vi "Beampointing_Multi_TRA2_BELLA_BTL.vi"() -> ()   [LabVIEW 2020]
uses:
  Shared/GUI_Template/GUI_master/tcp_new_data_event.ctl
  Shared/GUI_Template/GUI_master/tcp new data cluster.ctl
  Ctrs/beam detection.ctl
  GUI_Beampointing_single_TRA/Ctrs/move.ctl
  General GUIs/Device GUIs/GUI_Cameras/Controls/Crosshair type def.ctl
  <vilib>/Utility/file.llb/Read From Spreadsheet File (string).vi
  <userlib>/_OpenG.lib/array/array.llb/Filter 1D Array with Scalar (String)__ogtk.vi
  <vilib>/Analysis/NI_AALBase.lvlib
  <vilib>/vision/NI_Vision_Development_Module.lvlib
  <vilib>/Utility/file.llb/Write To Spreadsheet File (string).vi
panel:
  out "error out 3":errorcluster
  out "Array 3":sgl[](array[numeric])
  in  "GUIdevice 97":string="BELLA_ESP_2"
  in  "GUIdevice 98":string="BellaESP"
  in  "Position.Axis 1::97":dbl=77.0 caption="Motor Axis 1" min=-10.0 max=10.0 format="%#_6f"
  in  "Position.Axis 2::97":dbl=77.0 caption="Motor Axis 1" min=-12.0 max=10.0 format="%#_6f"
  in  "Position.Axis 3::97":dbl=77.0 caption="Motor Axis 1" min=-12.0 max=12.0 format="%#_6f"
  in  "Position.Axis 1::98":dbl=77.0 caption="Motor Axis 1" min=-8.0 max=6.0 format="%#_6f"
  in  "Position.Axis 2::98":dbl=77.0 caption="Motor Axis 1" min=-6.0 max=6.0 format="%#_6f"
  in  "Position.Axis 3::98":dbl=77.0 caption="Motor Axis 1" min=-10.0 max=10.0 format="%#_6f"
  in  "save path":path=path "W:/BP_DATA"
  out "size(s) 6":i32
  out "config path":string
  out "motor refs 7":refnum<vi>[](array[refnum])
  out "Moving Y":string
  out "Moving X":string
  out "particles":T1(array[cluster])
  out "motor refs 6":refnum<vi>[](array[refnum])
  out "millisecond timer value":u32
  out "motor refs 5":refnum<vi>[](array[refnum])
  out "appended path":path
  out "motor refs 4":refnum<vi>[](array[refnum])
  in  "active Axis ref 3":cluster{"Ref X":refnum<vi>, "Ref Y":refnum<vi>}
  out "motor refs 3":refnum<vi>[](array[refnum])
  in  "active man refs":cluster{"Ref X":refnum<vi>, "Ref Y":refnum<vi>}
  out "motor refs 2":refnum<vi>[](array[refnum])
  in  "Numeric":dbl
  out "Current State":string
  in  "output cluster 2":T5 {"detection para"."smal para"."Measurement Parameter" items=["Center of Mass X", "Center of Mass Y", "First Pixel X", "First Pixel Y", "Bounding Rect Left", "Bounding Rect Top", "Bounding Rect Right", "Bounding Rect Bottom", "Max Feret Diameter Start X", "Max Feret Diameter Start Y", "Max Feret Diameter End X", "Max Feret Diameter End Y", "Max Horiz. Segment Length Left", "Max Horiz. Segment Length Right", "Max Horiz. Segment Length Row", "-", "Bounding Rect Width", "Bounding Rect Height", "Bounding Rect Diagonal", "Perimeter", "Convex Hull Perimeter", "Holes' Perimeter", "Max Feret Diameter", "Equivalent Ellipse Major Axis", "Equivalent Ellipse Minor Axis", "Equivalent Ellipse Minor Axis (Feret)", "Equivalent Rect Long Side", "Equivalent Rect Short Side", "Equivalent Rect Diagonal", "Equivalent Rect Short Side (Feret)", "Average Horiz. Segment Length", "Average Vert. Segment Length", "Hydraulic Radius", "Waddel Disk Diameter", "-", "Area", "Holes' Area", "Particle & Holes' Area", "Convex Hull Area", "Image Area", "-", "Number of Holes", "Number of Horiz. Segments", "Number of Vert. Segments", "-", "Orientation", "Max Feret Diameter Orientation", "-", "% Area/Image Area", "% Area/(Particle & Holes' Area)", "Ratio of Equivalent Ellipse Axes", "Ratio of Equivalent Rect Sides", "-", "Elongation Factor", "Compactness Factor", "Heywood Circularity Factor", "Type Factor", "-", "Sum X", "Sum Y", "Sum XX", "Sum XY", "Sum YY", "Sum XXX", "Sum XXY", "Sum XYY", "Sum YYY", "-", "Moment of Inertia XX", "Moment of Inertia XY", "Moment of Inertia YY", "Moment of Inertia XXX", "Moment of Inertia XXY", "Moment of Inertia XYY", "Moment of Inertia YYY", "Norm. Moment of Inertia XX", "Norm. Moment of Inertia XY", "Norm. Moment of Inertia YY", "Norm. Moment of Inertia XXX", "Norm. Moment of Inertia XXY", "Norm. Moment of Inertia XYY", "Norm. Moment of Inertia YYY", "Hu Moment 1", "Hu Moment 2", "Hu Moment 3", "Hu Moment 4", "Hu Moment 5", "Hu Moment 6", "Hu Moment 7"]; "detection para"."smal para"."Range Lower Value" format="%.2f"; "detection para"."smal para"."Range Upper Value" format="%.2f"; "detection para"."detection method" items=["clustering", "entropy", "metric", "moments", "inter-class variance"]; "detection para"."Filter" items=["No Filter", "Median Filter", "Low Pass Filter"]}
  out "CCDs":string[](array[string])
  in  "GUIdevice 12":string
  in  "GUIdevice 11":string
  in  "GUIdevice 10":string
  in  "GUIdevice 9":string
  out "error out 2":errorcluster
  in  "active cams":string[](array[string])
  in  "Motor Y":dbl[][](array[numeric])
  in  "Motor X":dbl[][](array[numeric])
  out "Names":string[](array[string])
  in  "Offset X stats":dbl[][](array[numeric])
  in  "Offset Y stats":dbl[][](array[numeric])
  out "Box":T6(array[cluster])
  in  "Tab Cams":enum32{"Config ", "Main", "History"}(tab)=enum."Main"
  in  "associated motors":T7 {"Motor CCD 12" items=["M1", "M2", "M4", "M5"]; "Motor CCD 11" items=["M1", "M2", "M4", "M5"]; "Motor CCD 10" items=["M1", "M2", "M4", "M5"]; "Motor CCD 9" items=["M1", "M2", "M4", "M5"]; "Motor CCD 8" items=["M1", "M2", "M4", "M5"]; "Motor CCD 7" items=["M1", "M2", "M4", "M5"]; "Motor CCD 6" items=["M1", "M2", "M4", "M5"]; "Motor CCD 5" items=["M1", "M2", "M4", "M5"]; "Motor CCD 4" items=["M1", "M2", "M4", "M5"]; "Motor CCD 3" items=["M1", "M2", "M4", "M5"]; "Motor CCD 2" items=["M1", "M2", "M4", "M5"]; "Motor CCD 1" items=["M1", "M2", "M4", "M5"]}
  out "Cameras":T8
  out "Status":cluster{i32, i32, "Centroid X":dbl[][]}(graph)
  in  "Exposure:12":dbl=0.095 min=0.0001 max=1.0 format="%#_6f"
  in  "Triggerdelay::12":dbl=0.003 min=0.0 max=0.09 format="%#_6f"
  in  "Exposure::11":dbl=0.095 min=0.0001 max=1.0 format="%#_6f"
  in  "Triggerdelay::11":dbl=0.003 min=0.0 max=0.09 format="%#_6f"
  in  "Exposure::10":dbl=0.095 min=0.0001 max=1.0 format="%#_6f"
  in  "Triggerdelay::10":dbl=0.003 min=0.0 max=0.09 format="%#_6f"
  in  "Exposure::9":dbl=0.095 min=0.0001 max=1.0 format="%#_6f"
  in  "Triggerdelay::9":dbl=0.003 min=0.0 max=0.09 format="%#_6f"
  in  "Trigger::9":bool
  in  "Trigger::10":bool caption="Trigger:10"
  in  "Trigger::11":bool
  in  "Trigger::12":bool
  in  "Target.Y::9":dbl=45.0 caption="T9y" min=0.0 max=2000.0 format="%#_6f"
  in  "Target.X::9":dbl=47.0 caption="Tx9" min=0.0 max=2000.0 format="%#_6f"
  in  "Target.Y::10":dbl=45.0 caption="T10y" min=0.0 max=2000.0 format="%#_6f"
  in  "Target.X::10":dbl=47.0 caption="T10x" min=0.0 max=2000.0 format="%#_6f"
  in  "Target.Y::11":dbl=45.0 caption="T11y" min=0.0 max=2000.0 format="%#_6f"
  in  "Target.X::11":dbl=47.0 caption="T11x" min=0.0 max=2000.0 format="%#_6f"
  in  "Target.Y::12":dbl=45.0 caption="T12y" min=0.0 max=2000.0 format="%#_6f"
  in  "Target.X::12":dbl=47.0 caption="T12x" min=0.0 max=2000.0 format="%#_6f"
  in  "Exposure::8":dbl=0.095 min=0.0001 max=1.0 format="%#_6f"
  in  "Triggerdelay::8":dbl=0.003 min=0.0 max=0.09 format="%#_6f"
  in  "Trigger::8":bool
  in  "Target.Y::8":dbl=45.0 caption="T8y" min=0.0 max=2000.0 format="%#_6f"
  in  "Target.X::8":dbl=47.0 caption="T8x" min=0.0 max=2000.0 format="%#_6f"
  in  "Target.Y::7":dbl=45.0 caption="T7x" min=0.0 max=2000.0 format="%#_6f"
  in  "Target.X::7":dbl=47.0 caption="T7y" min=0.0 max=2000.0 format="%#_6f"
  in  "Target.Y::6":dbl=45.0 caption="T6y" min=0.0 max=2000.0 format="%#_6f"
  in  "Target.X::6":dbl=47.0 caption="T6x" min=0.0 max=2000.0 format="%#_6f"
  in  "Target.Y::5":dbl=45.0 caption="T5y" min=0.0 max=2000.0 format="%#_6f"
  in  "Target.X::5":dbl=47.0 caption="T5x" min=0.0 max=2000.0 format="%#_6f"
  in  "Target.Y::4":dbl=45.0 caption="T4y" min=0.0 max=2000.0 format="%#_6f"
  in  "Target.X::4":dbl=47.0 caption="T4x" min=0.0 max=2000.0 format="%#_6f"
  in  "Target.Y::3":dbl=163.0 caption="T3y" min=0.0 max=2000.0 format="%#_6f"
  in  "Target.X::3":dbl=152.0 caption="T3x" min=0.0 max=2000.0 format="%#_6f"
  in  "Target.Y::2":dbl=74.0 caption="T2y" min=0.0 max=2000.0 format="%#_6f"
  in  "Target.X::2":dbl=75.0 caption="T2x" min=0.0 max=2000.0 format="%#_6f"
  in  "Target.Y::1":dbl=61.0 caption="T1y" min=0.0 max=2000.0 format="%#_6f"
  in  "Target.X::1":dbl=77.0 caption="T1x" min=0.0 max=2000.0 format="%#_6f"
  in  "Exposure::7":dbl=0.095 min=3.8e-05 max=1.0 format="%#_6f"
  in  "Triggerdelay::7":dbl=0.003 min=0.0 max=0.09 format="%#_6f"
  in  "Trigger::7":bool
  in  "Exposure::6":dbl=0.095 min=3.8e-05 max=1.0 format="%#_6f"
  in  "Triggerdelay::6":dbl=0.003 min=0.0 max=0.09 format="%#_6f"
  in  "Trigger::6":bool
  in  "Exposure::5":dbl=0.095 min=3.8e-05 max=1.0 format="%#_6f"
  in  "Triggerdelay::5":dbl=0.003 min=0.0 max=0.09 format="%#_6f"
  in  "Trigger::5":bool
  in  "Exposure::4":dbl=0.095 min=3.8e-05 max=1.0 format="%#_6f"
  in  "Triggerdelay::4":dbl=0.003 min=0.0 max=0.09 format="%#_6f"
  in  "Trigger::4":bool
  in  "Exposure::3":dbl=0.095 min=3.8e-05 max=1.0 format="%#_6f"
  in  "Triggerdelay::3":dbl=0.003 min=0.0 max=0.09 format="%#_6f"
  in  "Trigger::3":bool
  in  "Exposure::2":dbl=0.095 min=3.8e-05 max=1.0 format="%#_6f"
  in  "Triggerdelay::2":dbl=0.003 min=0.0 max=0.09 format="%#_6f"
  in  "Trigger::2":bool
  out "image::1":T9(plugin-control) caption="M2Cam"
  out "image::2":T9(plugin-control) caption="HPDccd2"
  out "image::3":T9(plugin-control) caption="M3HPD_CCD_Near"
  out "image::4":T9(plugin-control)
  out "image::5":T9(plugin-control)
  out "image::6":T9(plugin-control)
  out "image::7":T9(plugin-control)
  out "image::8":T9(plugin-control)
  in  "Exposure::1":dbl=0.095 min=3.8e-05 max=1.0 format="%#_6f"
  in  "Triggerdelay::1":dbl=0.003 min=0.0 max=0.09 format="%#_6f"
  in  "Trigger::1":bool
  in  "UDP error message":string
  out "required Y":bool[](array[boolean])
  out "required X":bool[](array[boolean])
  out "detected":bool[](array[boolean])
  out "name array":string[](array[string])
  out "image::9":T9(plugin-control)
  out "image::10":T9(plugin-control)
  out "image::11":T9(plugin-control)
  out "image::12":T9(plugin-control)
  out "speedmode X":bool[](array[boolean])
  out "speedmode Y":bool[](array[boolean])
  out "CCD 9":cluster{timestamp[], dbl[]}[](graph)
  out "CCD 10":cluster{timestamp[], dbl[]}[](graph)
  out "CCD 11":cluster{timestamp[], dbl[]}[](graph)
  out "CCD 12":cluster{timestamp[], dbl[]}[](graph)
  out "CCD 5":cluster{timestamp[], dbl[]}[](graph)
  out "CCD 6":cluster{timestamp[], dbl[]}[](graph)
  out "CCD 7":cluster{timestamp[], dbl[]}[](graph)
  out "CCD 8":cluster{timestamp[], dbl[]}[](graph)
  out "CCD 2":cluster{timestamp[], dbl[]}[](graph)
  out "CCD 1":cluster{timestamp[], dbl[]}[](graph)
  out "CCD 3":cluster{timestamp[], dbl[]}[](graph)
  out "CCD 4":cluster{timestamp[], dbl[]}[](graph)
  in  "History Size":i32=500
  out "History Index":i32
  in  "Feedback Global":bool
  in  "detection para":T3[](array[typedef])=[{"Filter"=1, "Filter Para"={"X Size"=5, "Y Size"=5, "% Tolerance"=1}, "detection method"=4, "smal para"=[{"Measurement Parameter"=35, "Range Lower Value"=0.0, "Range Upper Value"=0.0, "Range"=TRUE, "Measurement Type"=FALSE}], "Remove small Objects"=TRUE, "Restrict to round Objects"=FALSE}, {"Filter"=1, "Filter Para"={"X Size"=5, "Y Size"=5, "% Tolerance"=1}, "detection method"=4, "smal para"=[{"Measurement Parameter"=35, "Range Lower Value"=0.0, "Range Upper Value"=500.0, "Range"=FALSE, "Measurement Type"=FALSE}], "Remove small Objects"=TRUE, "Restrict to round Objects"=FALSE}, {"Filter"=1, "Filter Para"={"X Size"=5, "Y Size"=5, "% Tolerance"=1}, "detection method"=4, "smal para"=[{"Measurement Parameter"=35, "Range Lower Value"=0.0, "Range Upper Value"=500.0, "Range"=TRUE, "Measurement Type"=FALSE}], "Remove small Objects"=TRUE, "Restrict to round Objects"=FALSE}, {"Filter"=1, "Filter Para"={"X Size"=5, "Y Size"=5, "% Tolerance"=1}, "detection method"=4, "smal para"=[{"Measurement Parameter"=35, "Range Lower Value"=0.0, "Range Upper Value"=500.0, "Range"=TRUE, "Measurement Type"=FALSE}], "Remove small Objects"=TRUE, "Restrict to round Objects"=FALSE}, {"Filter"=1, "Filter Para"={"X Size"=5, "Y Size"=5, "% Tolerance"=1}, "detection method"=4, "smal para"=[{"Measurement Parameter"=35, "Range Lower Value"=0.0, "Range Upper Value"=500.0, "Range"=TRUE, "Measurement Type"=FALSE}], "Remove small Objects"=TRUE, "Restrict to round Objects"=FALSE}, {"Filter"=1, "Filter Para"={"X Size"=5, "Y Size"=5, "% Tolerance"=1}, "detection method"=4, "smal para"=[{"Measurement Parameter"=35, "Range Lower Value"=0.0, "Range Upper Value"=500.0, "Range"=TRUE, "Measurement Type"=FALSE}], "Remove small Objects"=TRUE, "Restrict to round Objects"=FALSE}, {"Filter"=1, "Filter Para"={"X Size"=5, "Y Size"=5, "% Tolerance"=1}, "detection method"=4, "smal para"=[{"Measurement Parameter"=35, "Range Lower Value"=0.0, "Range Upper Value"=500.0, "Range"=TRUE, "Measurement Type"=FALSE}], "Remove small Objects"=TRUE, "Restrict to round Objects"=FALSE}, {"Filter"=1, "Filter Para"={"X Size"=5, "Y Size"=5, "% Tolerance"=1}, "detection method"=3, "smal para"=[{"Measurement Parameter"=35, "Range Lower Value"=0.0, "Range Upper Value"=0.0, "Range"=FALSE, "Measurement Type"=FALSE}], "Remove small Objects"=TRUE, "Restrict to round Objects"=FALSE}, {"Filter"=1, "Filter Para"={"X Size"=5, "Y Size"=5, "% Tolerance"=1}, "detection method"=4, "smal para"=[{"Measurement Parameter"=35, "Range Lower Value"=0.0, "Range Upper Value"=0.0, "Range"=FALSE, "Measurement Type"=FALSE}], "Remove small Objects"=TRUE, "Restrict to round Objects"=FALSE}, {"Filter"=1, "Filter Para"={"X Size"=5, "Y Size"=5, "% Tolerance"=1}, "detection method"=4, "smal para"=[{"Measurement Parameter"=35, "Range Lower Value"=0.0, "Range Upper Value"=500.0, "Range"=TRUE, "Measurement Type"=FALSE}], "Remove small Objects"=TRUE, "Restrict to round Objects"=FALSE}, {"Filter"=1, "Filter Para"={"X Size"=5, "Y Size"=5, "% Tolerance"=1}, "detection method"=4, "smal para"=[{"Measurement Parameter"=35, "Range Lower Value"=0.0, "Range Upper Value"=500.0, "Range"=TRUE, "Measurement Type"=FALSE}], "Remove small Objects"=TRUE, "Restrict to round Objects"=FALSE}, {"Filter"=1, "Filter Para"={"X Size"=5, "Y Size"=5, "% Tolerance"=1}, "detection method"=4, "smal para"=[{"Measurement Parameter"=35, "Range Lower Value"=0.0, "Range Upper Value"=500.0, "Range"=TRUE, "Measurement Type"=FALSE}], "Remove small Objects"=TRUE, "Restrict to round Objects"=FALSE}] {"smal para"."Measurement Parameter" items=["Center of Mass X", "Center of Mass Y", "First Pixel X", "First Pixel Y", "Bounding Rect Left", "Bounding Rect Top", "Bounding Rect Right", "Bounding Rect Bottom", "Max Feret Diameter Start X", "Max Feret Diameter Start Y", "Max Feret Diameter End X", "Max Feret Diameter End Y", "Max Horiz. Segment Length Left", "Max Horiz. Segment Length Right", "Max Horiz. Segment Length Row", "-", "Bounding Rect Width", "Bounding Rect Height", "Bounding Rect Diagonal", "Perimeter", "Convex Hull Perimeter", "Holes' Perimeter", "Max Feret Diameter", "Equivalent Ellipse Major Axis", "Equivalent Ellipse Minor Axis", "Equivalent Ellipse Minor Axis (Feret)", "Equivalent Rect Long Side", "Equivalent Rect Short Side", "Equivalent Rect Diagonal", "Equivalent Rect Short Side (Feret)", "Average Horiz. Segment Length", "Average Vert. Segment Length", "Hydraulic Radius", "Waddel Disk Diameter", "-", "Area", "Holes' Area", "Particle & Holes' Area", "Convex Hull Area", "Image Area", "-", "Number of Holes", "Number of Horiz. Segments", "Number of Vert. Segments", "-", "Orientation", "Max Feret Diameter Orientation", "-", "% Area/Image Area", "% Area/(Particle & Holes' Area)", "Ratio of Equivalent Ellipse Axes", "Ratio of Equivalent Rect Sides", "-", "Elongation Factor", "Compactness Factor", "Heywood Circularity Factor", "Type Factor", "-", "Sum X", "Sum Y", "Sum XX", "Sum XY", "Sum YY", "Sum XXX", "Sum XXY", "Sum XYY", "Sum YYY", "-", "Moment of Inertia XX", "Moment of Inertia XY", "Moment of Inertia YY", "Moment of Inertia XXX", "Moment of Inertia XXY", "Moment of Inertia XYY", "Moment of Inertia YYY", "Norm. Moment of Inertia XX", "Norm. Moment of Inertia XY", "Norm. Moment of Inertia YY", "Norm. Moment of Inertia XXX", "Norm. Moment of Inertia XXY", "Norm. Moment of Inertia XYY", "Norm. Moment of Inertia YYY", "Hu Moment 1", "Hu Moment 2", "Hu Moment 3", "Hu Moment 4", "Hu Moment 5", "Hu Moment 6", "Hu Moment 7"]; "smal para"."Range Lower Value" format="%.2f"; "smal para"."Range Upper Value" format="%.2f"; "detection method" items=["clustering", "entropy", "metric", "moments", "inter-class variance"]; "Filter" items=["No Filter", "Median Filter", "Low Pass Filter"]}
  in  "GUIdevice 8":string
  in  "Tab Control":T10(tab)
  in  "alarms":bool
  in  "new tdms":bool
  in  "Save Stats":bool
  in  "Save Config":bool
  in  "Load Config":bool
  in  "update speed [ms]":i32=2000
  in  "img to avg":i32=6 min=3 max=200
  in  "Reset History":bool
  in  "autodetect":bool
  in  "Detection Rate":dbl=0.9 min=0.001 max=1.0
  in  "Center":bool
  in  "Align":bool
  in  "Speedmode":dbl=5.0 min=1.0 max=20.0
  in  "device ini":bool
  in  "average centroid":bool
  in  "beam detection para":T3={"Filter"=1, "Filter Para"={"X Size"=5, "Y Size"=5, "% Tolerance"=1}, "detection method"=4, "smal para"=[{"Measurement Parameter"=35, "Range Lower Value"=0.0, "Range Upper Value"=500.0, "Range"=FALSE, "Measurement Type"=FALSE}], "Remove small Objects"=TRUE, "Restrict to round Objects"=FALSE} {"smal para"."Measurement Parameter" items=["Center of Mass X", "Center of Mass Y", "First Pixel X", "First Pixel Y", "Bounding Rect Left", "Bounding Rect Top", "Bounding Rect Right", "Bounding Rect Bottom", "Max Feret Diameter Start X", "Max Feret Diameter Start Y", "Max Feret Diameter End X", "Max Feret Diameter End Y", "Max Horiz. Segment Length Left", "Max Horiz. Segment Length Right", "Max Horiz. Segment Length Row", "-", "Bounding Rect Width", "Bounding Rect Height", "Bounding Rect Diagonal", "Perimeter", "Convex Hull Perimeter", "Holes' Perimeter", "Max Feret Diameter", "Equivalent Ellipse Major Axis", "Equivalent Ellipse Minor Axis", "Equivalent Ellipse Minor Axis (Feret)", "Equivalent Rect Long Side", "Equivalent Rect Short Side", "Equivalent Rect Diagonal", "Equivalent Rect Short Side (Feret)", "Average Horiz. Segment Length", "Average Vert. Segment Length", "Hydraulic Radius", "Waddel Disk Diameter", "-", "Area", "Holes' Area", "Particle & Holes' Area", "Convex Hull Area", "Image Area", "-", "Number of Holes", "Number of Horiz. Segments", "Number of Vert. Segments", "-", "Orientation", "Max Feret Diameter Orientation", "-", "% Area/Image Area", "% Area/(Particle & Holes' Area)", "Ratio of Equivalent Ellipse Axes", "Ratio of Equivalent Rect Sides", "-", "Elongation Factor", "Compactness Factor", "Heywood Circularity Factor", "Type Factor", "-", "Sum X", "Sum Y", "Sum XX", "Sum XY", "Sum YY", "Sum XXX", "Sum XXY", "Sum XYY", "Sum YYY", "-", "Moment of Inertia XX", "Moment of Inertia XY", "Moment of Inertia YY", "Moment of Inertia XXX", "Moment of Inertia XXY", "Moment of Inertia XYY", "Moment of Inertia YYY", "Norm. Moment of Inertia XX", "Norm. Moment of Inertia XY", "Norm. Moment of Inertia YY", "Norm. Moment of Inertia XXX", "Norm. Moment of Inertia XXY", "Norm. Moment of Inertia XYY", "Norm. Moment of Inertia YYY", "Hu Moment 1", "Hu Moment 2", "Hu Moment 3", "Hu Moment 4", "Hu Moment 5", "Hu Moment 6", "Hu Moment 7"]; "smal para"."Range Lower Value" format="%.2f"; "smal para"."Range Upper Value" format="%.2f"; "detection method" items=["clustering", "entropy", "metric", "moments", "inter-class variance"]; "Filter" items=["No Filter", "Median Filter", "Low Pass Filter"]}
  in  "move config":T2={"Tolerance [%]"=0.1, "Stepsize"=0.0001, "Invert Axis"=TRUE, "Invert Direction X"=FALSE, "Invert Direction Y"=TRUE, "enable feedback"=FALSE, "Set Centriod Target"=FALSE}
  in  "Position 2":dbl=0.001 caption="Stepsize" min=0.0 max=999999.0 format="%_6f"
  in  "Position 1":dbl=0.001 caption="Stepsize" min=0.0 max=999999.0 format="%_6f"
  in  "Right":bool caption="RelativeMove.Axis 1.CCW::1"
  in  "Left":bool caption="RelativeMove.Axis 1.CW::1"
  in  "Down":bool caption="RelativeMove.Axis. 2.CCW::1"
  in  "Up":bool caption="RelativeMove.Axis 2.CW::1"
  in  "StepSize":dbl=1.0 caption="Stepsize" min=0.0 max=1.0 step=0.001 format="%#_6p"
  in  "active axis refs 2":T11(array[cluster])
  in  "active Axis ref":cluster{"Ref X":refnum<vi>, "Ref Y":refnum<vi>}
  in  "CCDs":u16(ring) items=["M2Cam", "HPDccd2", "M3HPD_CCD_Near", "", "", "", "", "", "", "", "", ""]
  out "motor refs":refnum<vi>[](array[refnum])
  in  "Position.Axis 2::99":dbl=77.0 caption="Motor Axis 1" min=-3.0 max=3.0 format="%#_6f"
  in  "Position.Axis 1::99":dbl=77.0 caption="Motor Axis 1" min=-10.0 max=10.0 format="%#_6f"
  in  "GUIdevice 99":string="BELLA_ESP_M1"
  in  "move properties":T2[](array[typedef])=[{"Tolerance [%]"=0.1, "Stepsize"=0.0001, "Invert Axis"=TRUE, "Invert Direction X"=FALSE, "Invert Direction Y"=TRUE, "enable feedback"=FALSE, "Set Centriod Target"=FALSE}, {"Tolerance [%]"=0.1, "Stepsize"=0.0001, "Invert Axis"=TRUE, "Invert Direction X"=FALSE, "Invert Direction Y"=TRUE, "enable feedback"=FALSE, "Set Centriod Target"=FALSE}, {"Tolerance [%]"=0.1, "Stepsize"=0.0001, "Invert Axis"=TRUE, "Invert Direction X"=FALSE, "Invert Direction Y"=TRUE, "enable feedback"=FALSE, "Set Centriod Target"=FALSE}, {"Tolerance [%]"=0.1, "Stepsize"=0.0001, "Invert Axis"=TRUE, "Invert Direction X"=FALSE, "Invert Direction Y"=TRUE, "enable feedback"=FALSE, "Set Centriod Target"=FALSE}, {"Tolerance [%]"=0.1, "Stepsize"=0.0001, "Invert Axis"=TRUE, "Invert Direction X"=FALSE, "Invert Direction Y"=TRUE, "enable feedback"=FALSE, "Set Centriod Target"=FALSE}, {"Tolerance [%]"=0.1, "Stepsize"=0.0001, "Invert Axis"=TRUE, "Invert Direction X"=FALSE, "Invert Direction Y"=TRUE, "enable feedback"=FALSE, "Set Centriod Target"=FALSE}, {"Tolerance [%]"=0.1, "Stepsize"=0.0001, "Invert Axis"=TRUE, "Invert Direction X"=FALSE, "Invert Direction Y"=TRUE, "enable feedback"=FALSE, "Set Centriod Target"=FALSE}, {"Tolerance [%]"=0.1, "Stepsize"=0.0001, "Invert Axis"=TRUE, "Invert Direction X"=FALSE, "Invert Direction Y"=TRUE, "enable feedback"=FALSE, "Set Centriod Target"=FALSE}, {"Tolerance [%]"=0.1, "Stepsize"=0.0001, "Invert Axis"=TRUE, "Invert Direction X"=FALSE, "Invert Direction Y"=TRUE, "enable feedback"=FALSE, "Set Centriod Target"=FALSE}, {"Tolerance [%]"=0.1, "Stepsize"=0.0001, "Invert Axis"=TRUE, "Invert Direction X"=FALSE, "Invert Direction Y"=TRUE, "enable feedback"=FALSE, "Set Centriod Target"=FALSE}, {"Tolerance [%]"=0.1, "Stepsize"=0.0001, "Invert Axis"=TRUE, "Invert Direction X"=FALSE, "Invert Direction Y"=TRUE, "enable feedback"=FALSE, "Set Centriod Target"=FALSE}, {"Tolerance [%]"=0.1, "Stepsize"=0.0001, "Invert Axis"=TRUE, "Invert Direction X"=FALSE, "Invert Direction Y"=TRUE, "enable feedback"=FALSE, "Set Centriod Target"=FALSE}, {"Tolerance [%]"=0.1, "Stepsize"=0.0001, "Invert Axis"=TRUE, "Invert Direction X"=FALSE, "Invert Direction Y"=TRUE, "enable feedback"=FALSE, "Set Centriod Target"=FALSE}]
  in  "Time":timestamp[][](array[timestamp])
  in  "Mean Size":dbl[][](array[numeric])
  in  "Size":dbl[][](array[numeric])
  in  "active CCDs":i32(listbox)
  in  "Offset Y":dbl[][](array[numeric])
  in  "Offset X":dbl[][](array[numeric])
  in  "Mean Centroid X":dbl[][](array[numeric])
  in  "Mean Centroid Y":dbl[][](array[numeric])
  in  "Centroid Y":dbl[][](array[numeric])
  in  "Centroid X":dbl[][](array[numeric])
  in  "GUIdevice 7":string
  in  "GUIdevice 6":string
  in  "GUIdevice 5":string
  in  "GUIdevice 4":string
  in  "GUIdevice 3":string="TargetCam10Hz_Diode"
  in  "GUIdevice 2":string="StagingM1Far"
  in  "insert tag":bool=TRUE
  in  "stop":bool
  in  "GUIdevice 1":string="StagingM1Near"
  out "tcp data event":T12
  out "error IO 2":errorcluster
  # "max"
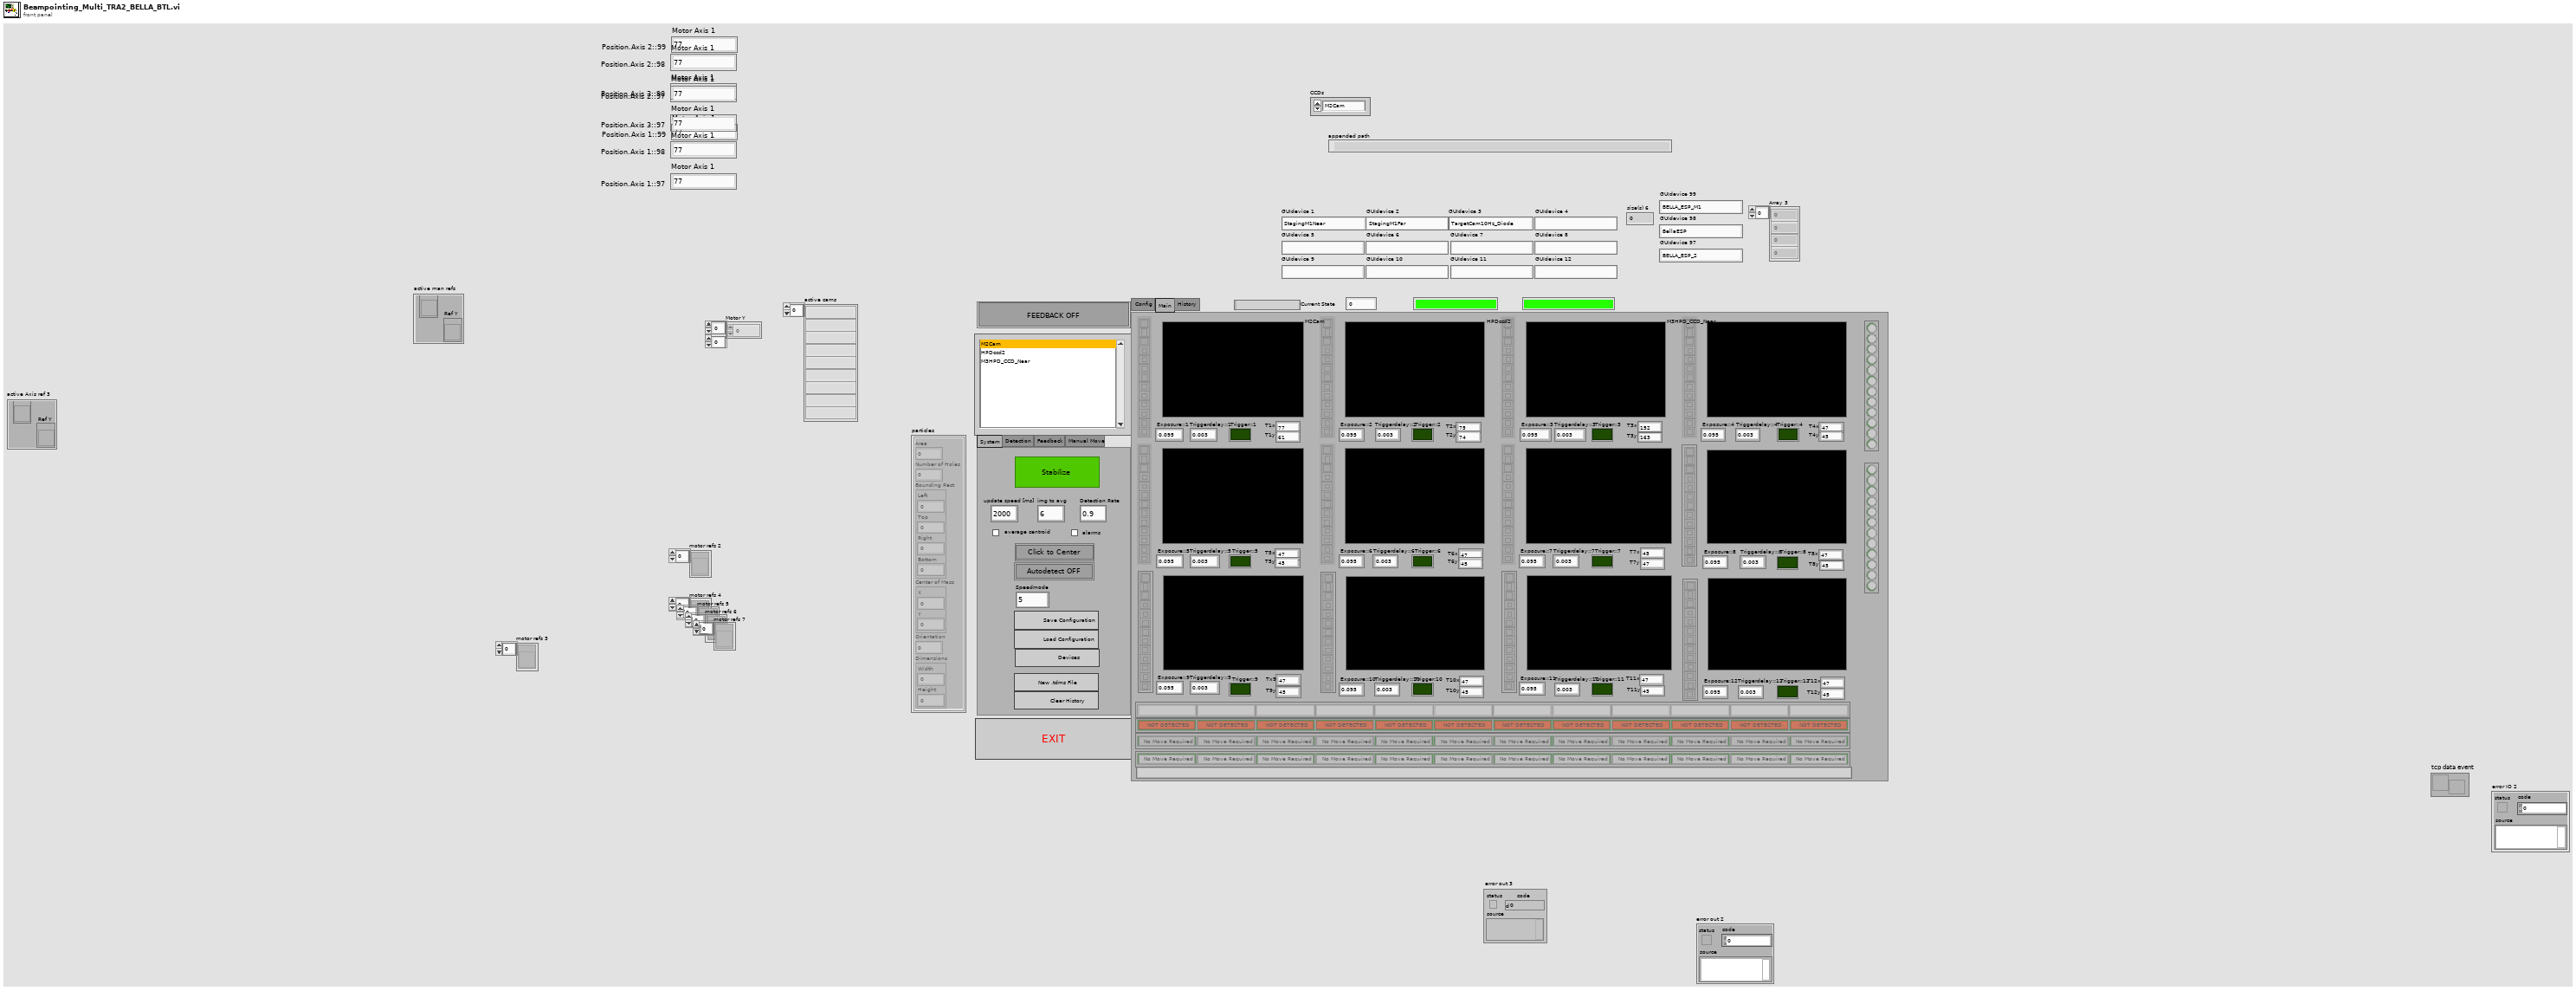
[diagram p1: front panel]
types:
  T1 = cluster{"Area":dbl, "Number of Holes":dbl, "Bounding Rect":cluster{"Left":dbl, "Top":dbl, "Right":dbl, "Bottom":dbl}, "Center of Mass":cluster{"X":dbl, "Y":dbl}, "Orientation":dbl, "Dimensions":cluster{"Width":dbl, "Height":dbl}}[]
  T2 = typedef "move.ctl" = cluster{"Tolerance [%]":dbl, "Stepsize":dbl, "Invert Axis":bool, "Invert Direction X":bool, "Invert Direction Y":bool, "enable feedback":bool, "Set Centriod Target":bool}
  T3 = typedef "beam detection.ctl" = cluster{"Filter":u16, "Filter Para":cluster{"X Size":i32, "Y Size":i32, "% Tolerance":i32}, "detection method":i32, "smal para":cluster{"Measurement Parameter":T4, "Range Lower Value":dbl, "Range Upper Value":dbl, "Range":bool, "Measurement Type":bool}[], "Remove small Objects":bool, "Restrict to round Objects":bool}
  T4 = typedef "Particle Parameters" = i32
  T5 = cluster{"CCDs":string[], "move properties":T2[], "detection para":T3[], "thresholds":cluster{"Lower value":sgl, "Upper value":sgl}[], "Value":cluster{"Motor CCD 1":u16, "Motor CCD 2":u16, "Motor CCD 3":u16, "Motor CCD 4":u16, "Motor CCD 5":u16, "Motor CCD 6":u16, "Motor CCD 7":u16, "Motor CCD 8":u16, "Motor CCD 9":u16, "Motor CCD 10":u16, "Motor CCD 11":u16, "Motor CCD 12":u16}}
  T6 = cluster{"Left":dbl, "Top":dbl, "Right":dbl, "Bottom":dbl}[]
  T7 = cluster{"Motor CCD 1":u16, "Motor CCD 2":u16, "Motor CCD 3":u16, "Motor CCD 4":u16, "Motor CCD 5":u16, "Motor CCD 6":u16, "Motor CCD 7":u16, "Motor CCD 8":u16, "Motor CCD 9":u16, "Motor CCD 10":u16, "Motor CCD 11":u16, "Motor CCD 12":u16}
  T8 = cluster{"[0]":string, "[1]":string, "[2]":string, "[3]":string, "[4]":string, "[5]":string, "[6]":string, "[7]":string, "[8]":string, "[8] 2":string, "[8] 3":string, "[8] 4":string}
  T9 = typedef "IMAQ Image.ctl" = refnum<image>
  T10 = enum32{"System", "Detection", "Feedback", "Manual Move"}
  T11 = cluster{"Ref X":refnum<vi>, "Ref Y":refnum<vi>}[]
  T12 = typedef "tcp_new_data_event.ctl" = refnum<user-event>
  T13 = typedef "tcp new data cluster.ctl" = cluster{"EventEnum":enum16{"new data", "connection status update"}, "Device name":string}
  T14 = enum32{"invalid app kind", "Development System", "Run Time System", "Student Edition", "Embedded LabVIEW", "Evaluation", "Custom"}
  T15 = enum16{"open", "open or create", "create or replace", "create", "open (read-only)"}
  T16 = enum32{"Invalid", "Standard", "Closed", "Hidden", "Minimized", "Maximized"}
  T17 = enum16{"open", "replace", "create", "open or create", "replace or create", "replace or create with confirmation"}
  T18 = enum8{"Enabled", "Disabled", "Disabled and Grayed Out"}
  T19 = typedef "Image Type" = u32
  T20 = cluster{"[0]":string, "[1]":string, "[2]":string, "[3]":string, "[4]":string, "[5]":string, "[6]":string, "[7]":string, "[8]":string, "[9]":string, "[10]":string, "[11]":string}
  T21 = cluster{"Target.X::1":refnum<vi>, "Target.Y::1":refnum<vi>}
  T22 = cluster{"Target.X::2":refnum<vi>, "Target.Y::2":refnum<vi>}
  T23 = cluster{"Target.X::3":refnum<vi>, "Target.Y::3":refnum<vi>}
  T24 = cluster{"Target.X::4":refnum<vi>, "Target.Y::4":refnum<vi>}
  T25 = cluster{"Target.X::5":refnum<vi>, "Target.Y::5":refnum<vi>}
  T26 = cluster{"Target.X::6":refnum<vi>, "Target.Y::6":refnum<vi>}
  T27 = cluster{"Target.X::7":refnum<vi>, "Target.Y::7":refnum<vi>}
  T28 = cluster{"Target.X::8":refnum<vi>, "Target.Y::8":refnum<vi>}
  T29 = cluster{"Target.X::12":refnum<vi>, "Target.Y::12":refnum<vi>}
  T30 = cluster{"Target.X::9":refnum<vi>, "Target.Y::9":refnum<vi>}
  T31 = cluster{"Target.X::10":refnum<vi>, "Target.Y::10":refnum<vi>}
  T32 = cluster{"Target.X::11":refnum<vi>, "Target.Y::11":refnum<vi>}
  T33 = cluster{"Target.X::12":refnum<vi>, "Target.Y::12":refnum<vi>}[]
  T34 = cluster{"Left":dbl, "Top":dbl, "Right":dbl, "Bottom":dbl}
  T35 = cluster{"Core":cluster{"Current VI Reference":refnum<vi>, "Close Panel on Exit?":bool}, "detection para":T3[], "thresholds":cluster{"Lower value":sgl, "Upper value":sgl}[], "Centroid X":dbl[][], "Centroid Y":dbl[][], "img to avg":i32, "Mean Centroid X":dbl[][], "Mean Centroid Y":dbl[][], "Offset X":dbl[][], "Offset Y":dbl[][], "Offset X stats ":dbl[][], "Offset Y stats ":dbl[][], "Size":dbl[][], "Mean Size":dbl[][], "Time":timestamp[][], "move properties":T2[], "active axis refs 2":cluster{"Ref X":refnum<vi>, "Ref Y":refnum<vi>}[], "active ccd":i32, "Feedback global":bool, "Motor X":dbl[][], "Motor Y":dbl[][], "active cams":string[], "Data Value Reference out":refnum<k34>, "active man refs":cluster{"Ref X":refnum<vi>, "Ref Y":refnum<vi>}, "detected":bool[], "speedmode X":bool[], "speedmode Y":bool[], "steps speed X":dbl[], "steps speed Y":dbl[]}
  T36 = cluster{"Current VI Reference":refnum<vi>, "Close Panel on Exit?":bool}
  T37 = cluster{"appended array":timestamp[], "appended array":dbl[]}
  T38 = cluster{"appended array":timestamp[], "appended array":dbl[]}[]
  T39 = typedef "Crosshair type def.ctl" = cluster{"Draw":bool, "Target":cluster{"x":dbl, "y":dbl}, "Size":cluster{"x":dbl, "y":dbl}, "Angle":dbl, "Color":u32, "Thickness":u8, "CrosshairLabel":string}
  T40 = cluster{"Left":i32, "Top":i32, "Right":i32, "Bottom":i32}
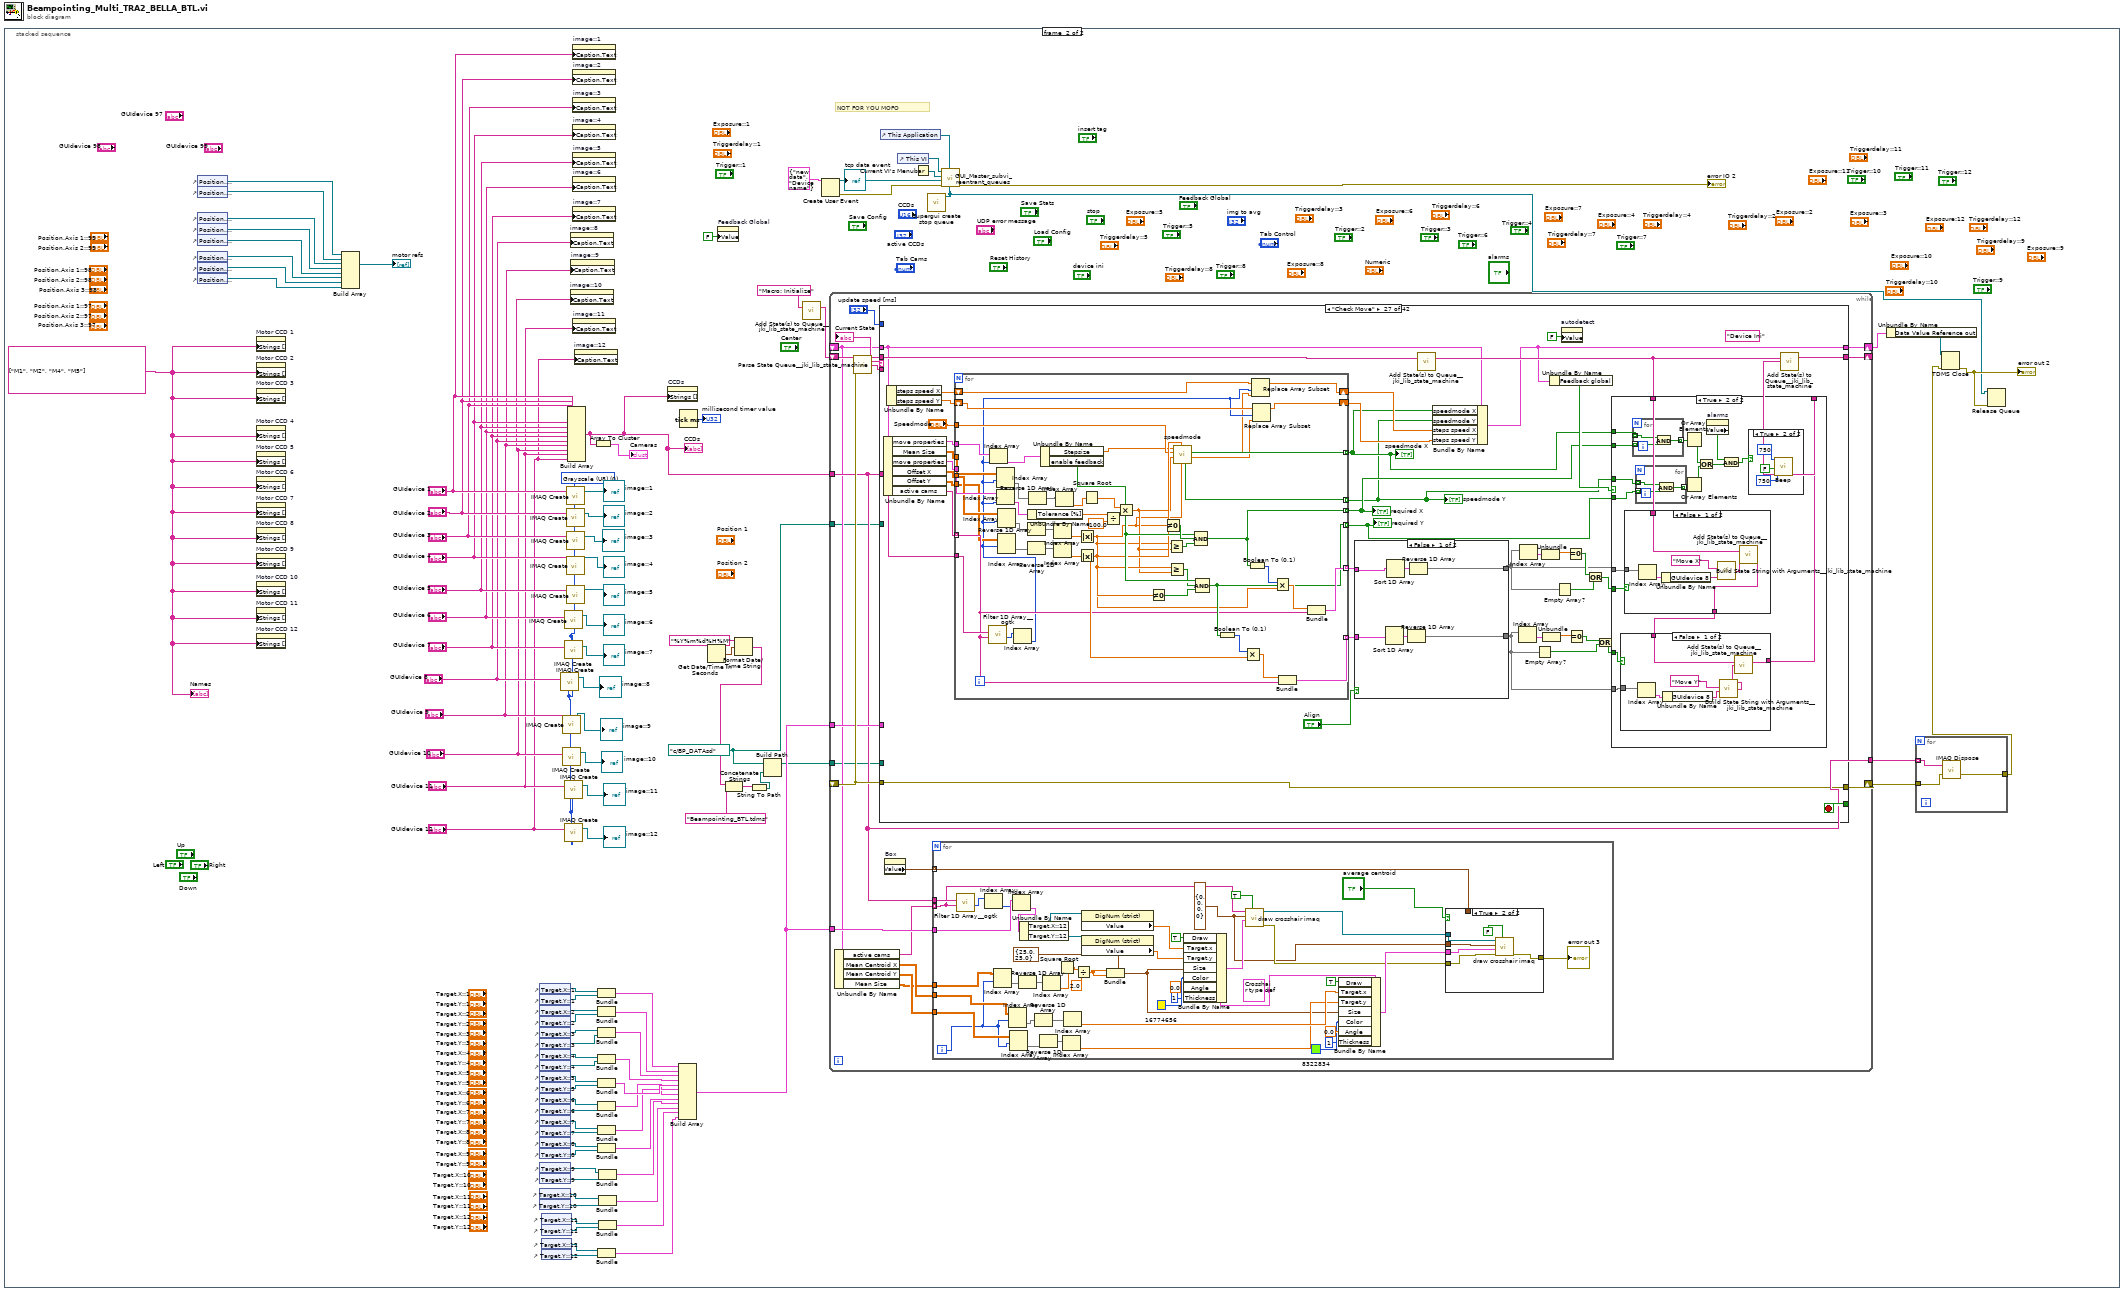
[diagram p0: block diagram]
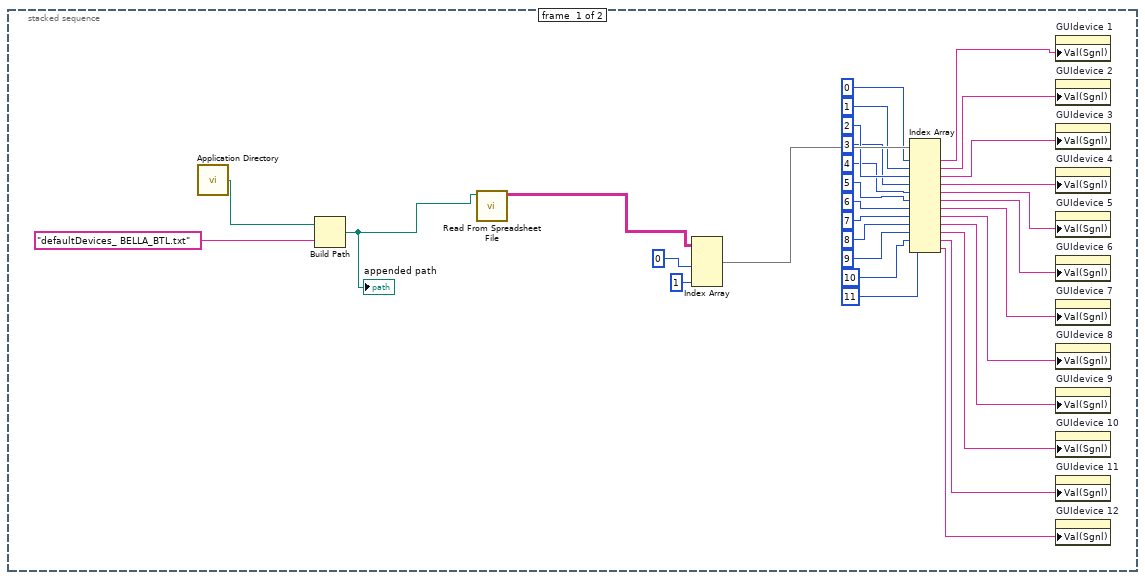
[diagram p2: hidden frame]
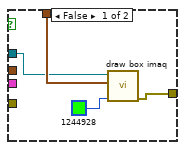
[diagram p3: hidden frame]
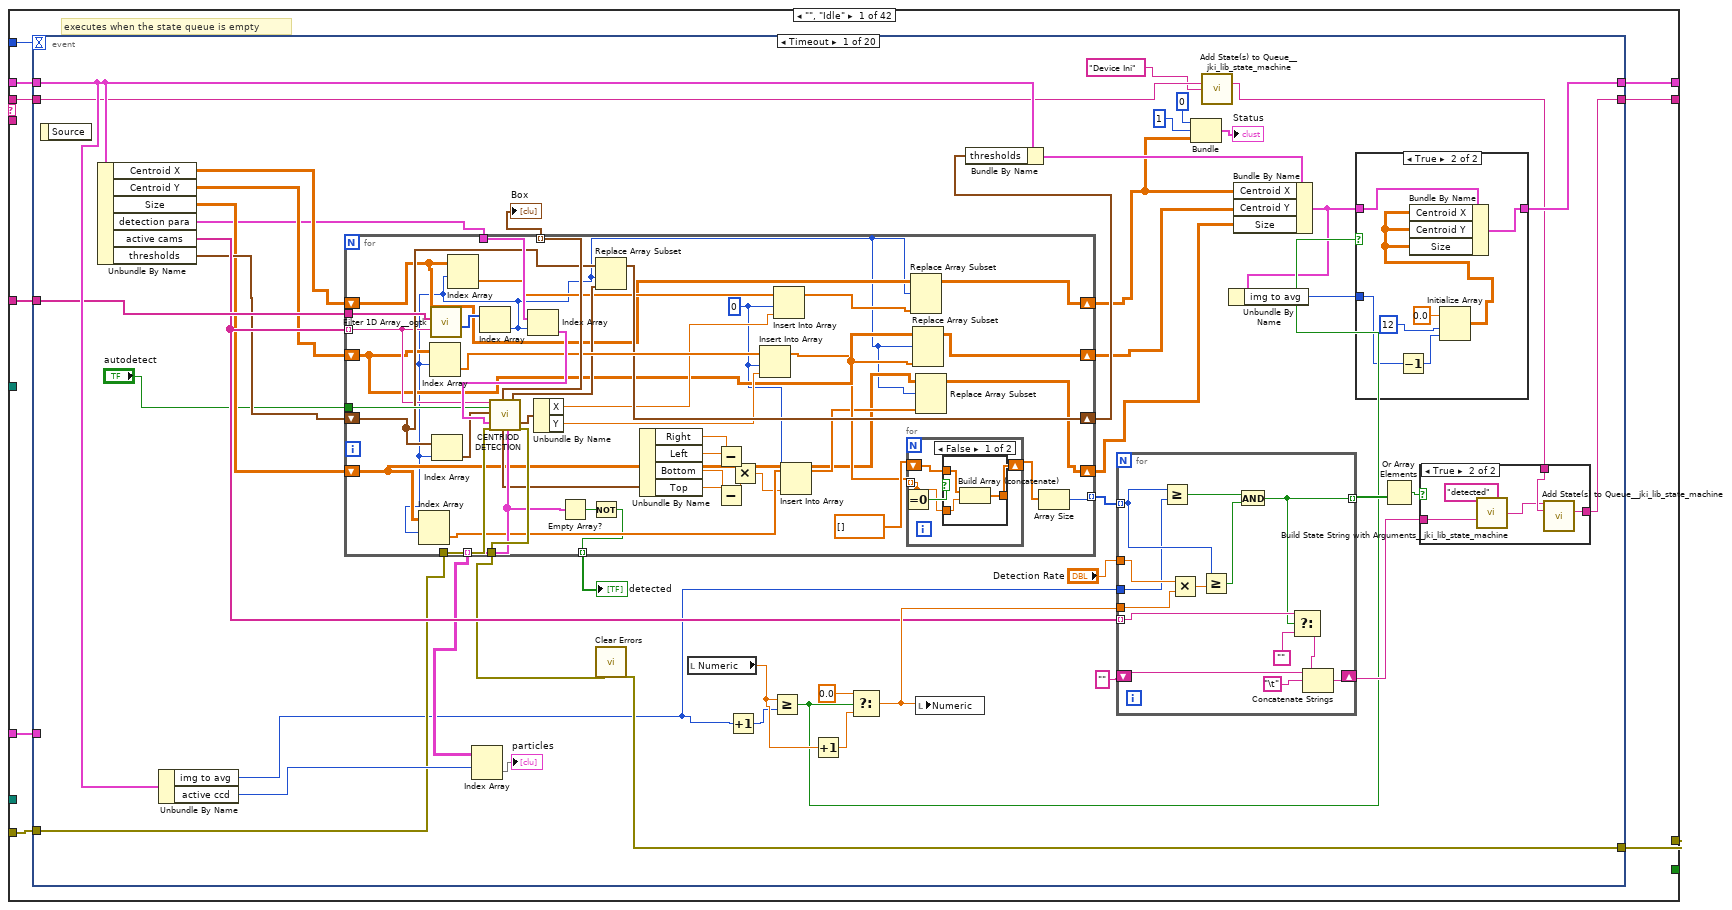
[diagram p4: hidden frame]
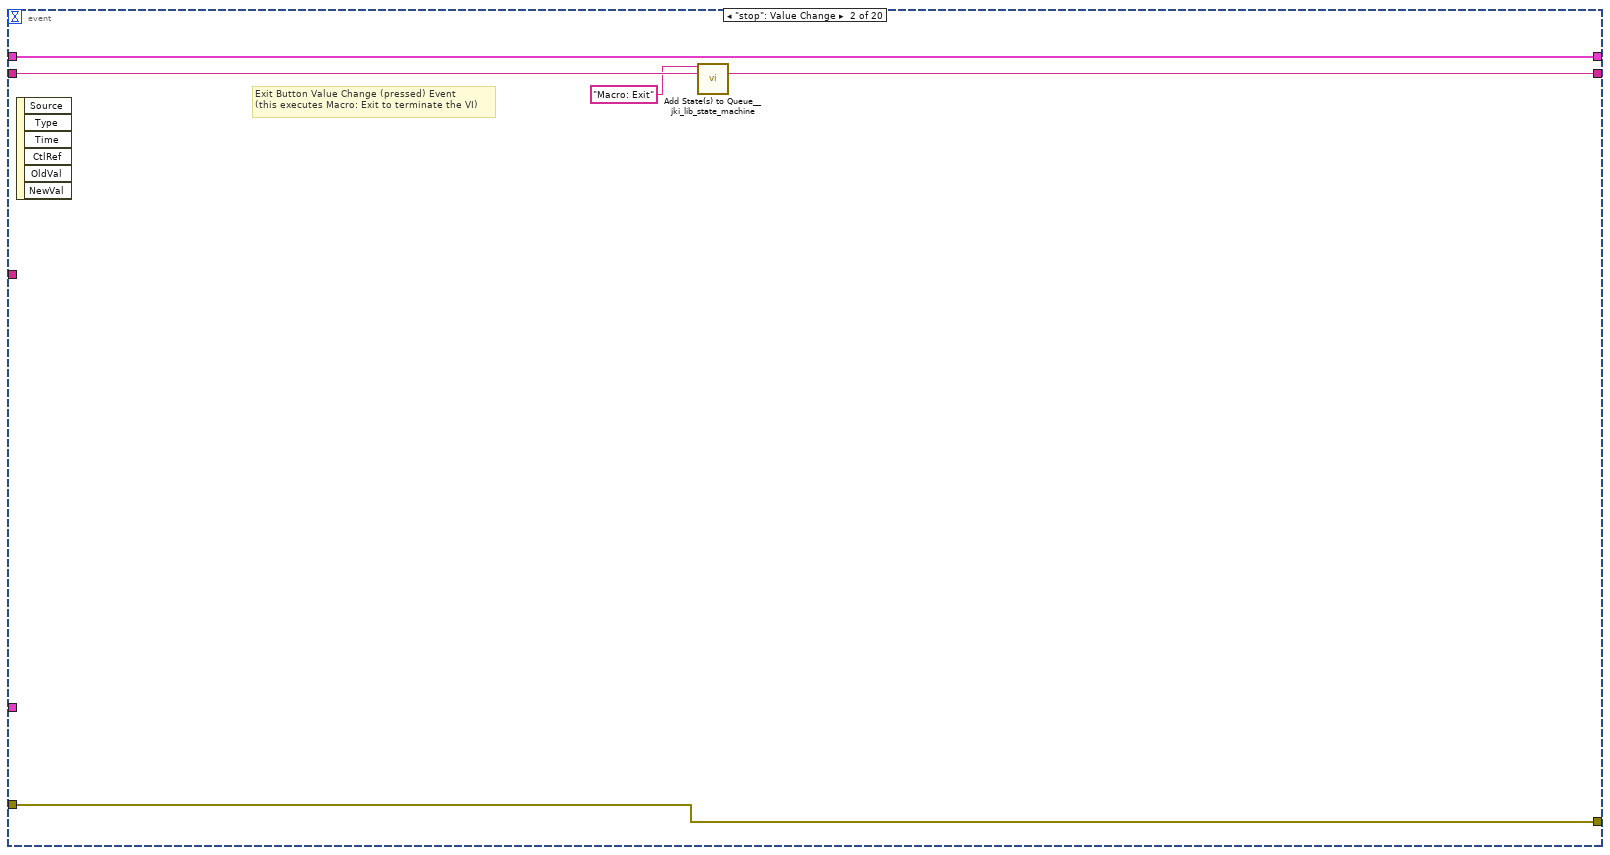
[diagram p8: hidden frame]
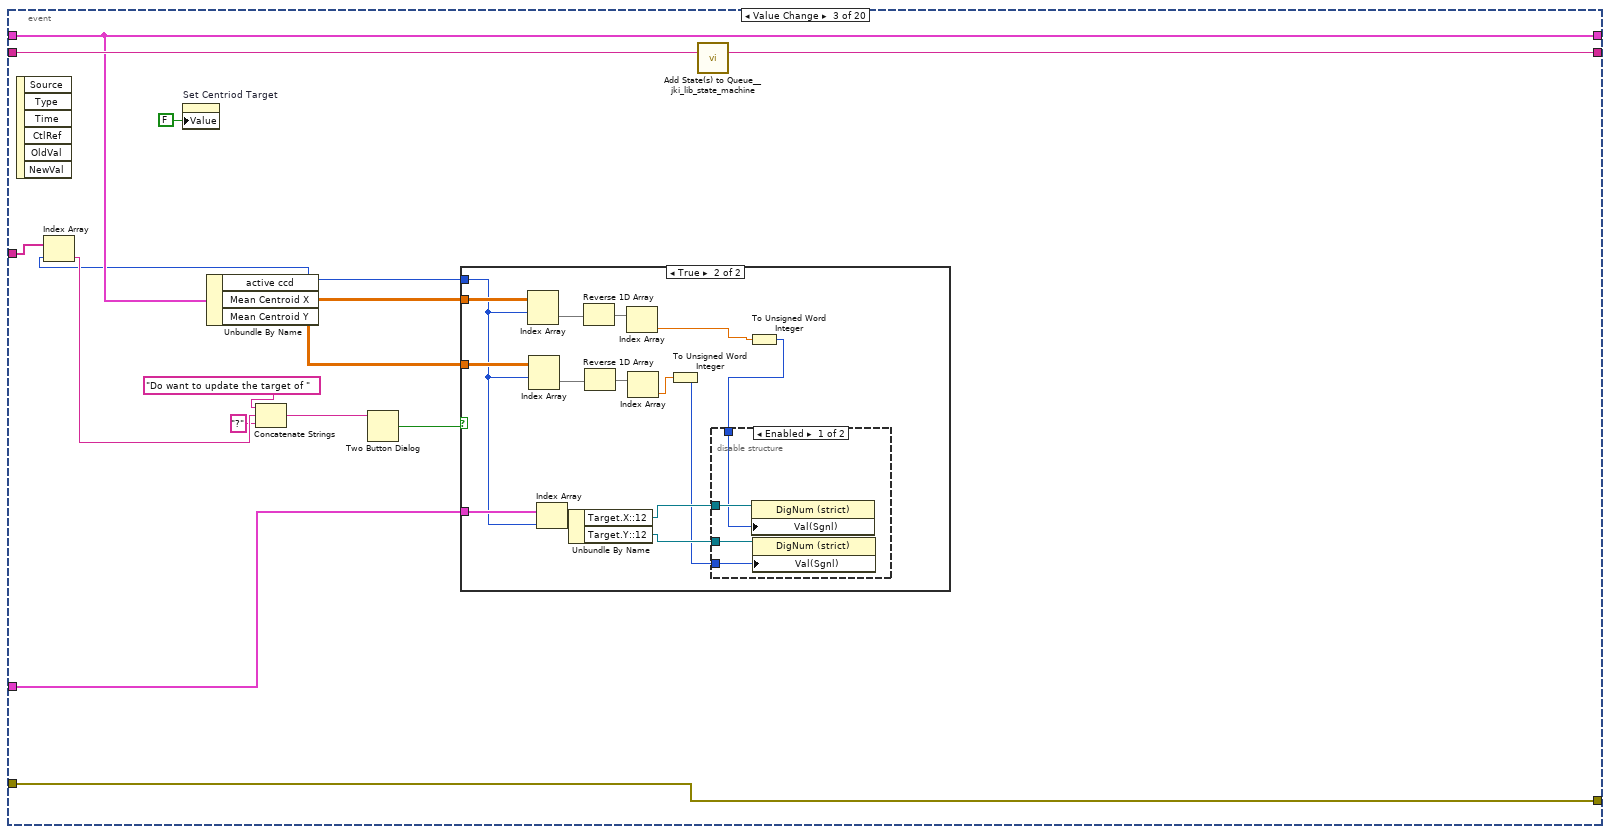
[diagram p9: hidden frame]
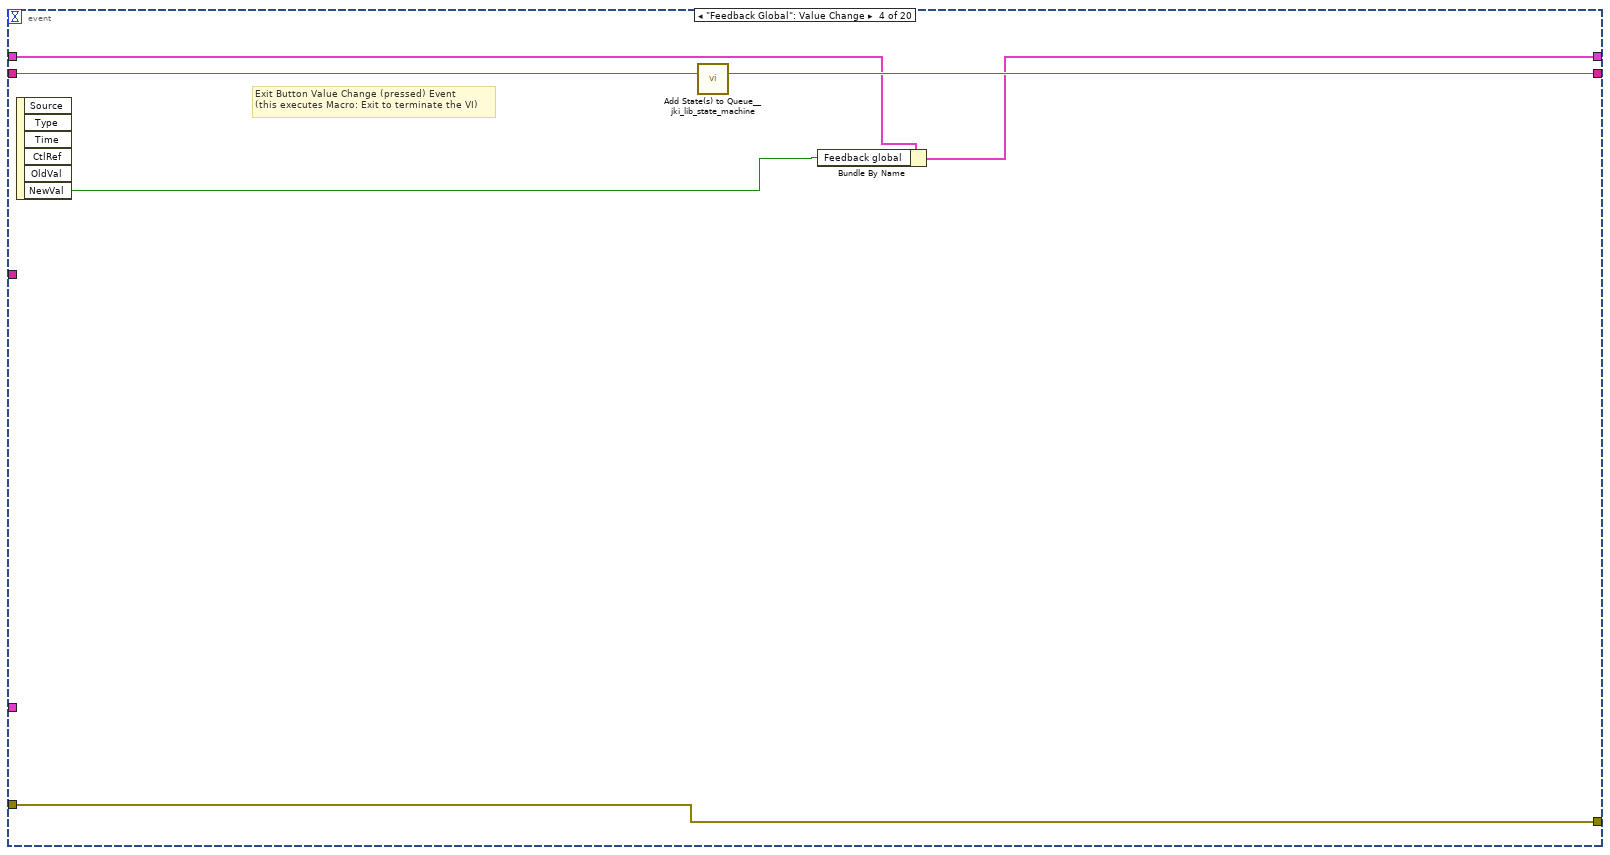
[diagram p12: hidden frame]
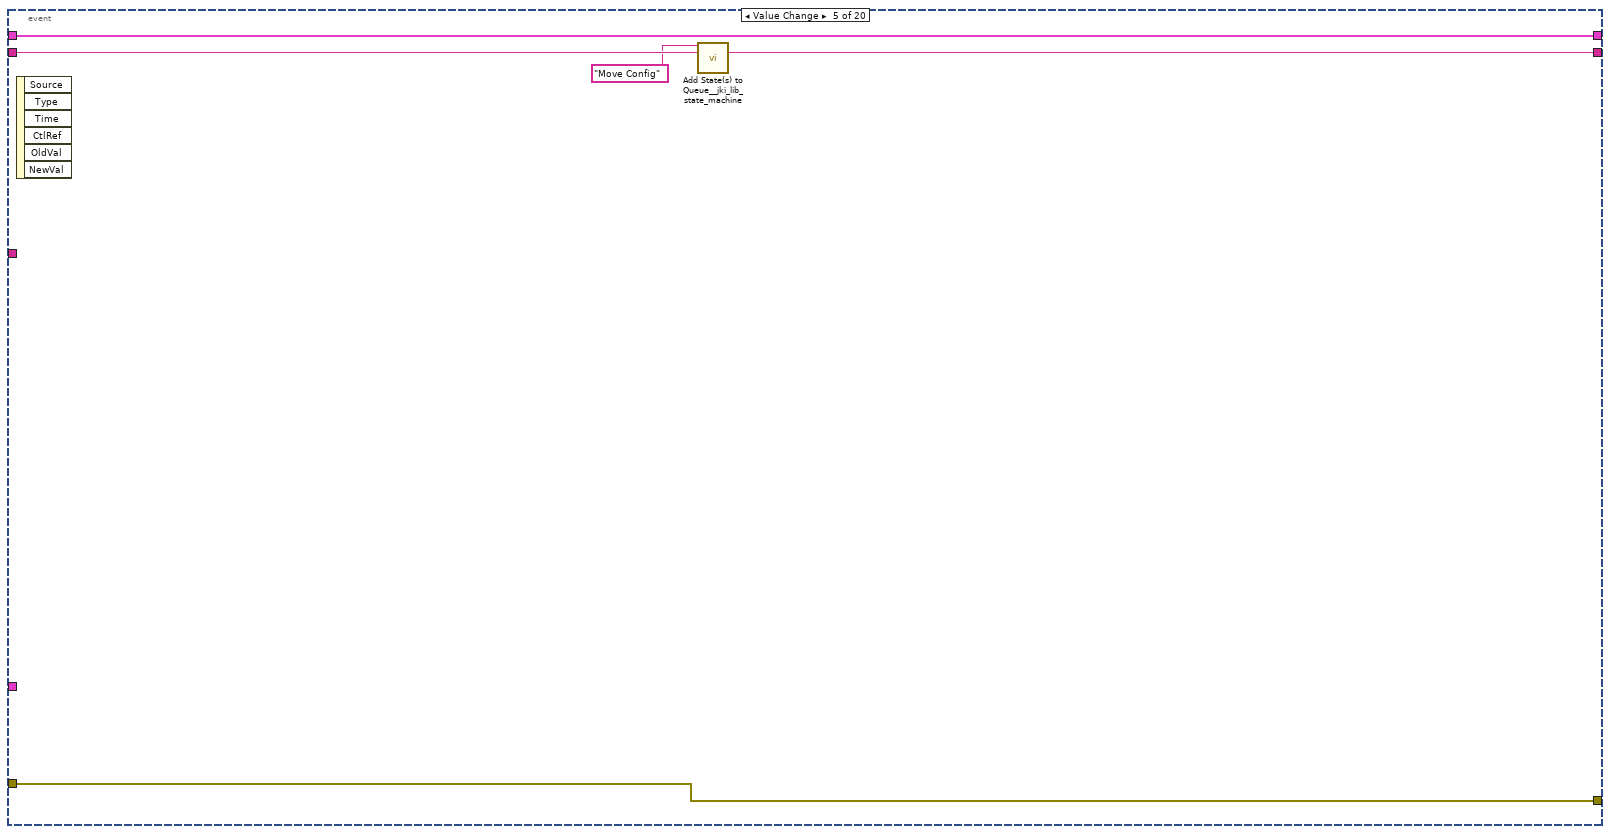
[diagram p13: hidden frame]
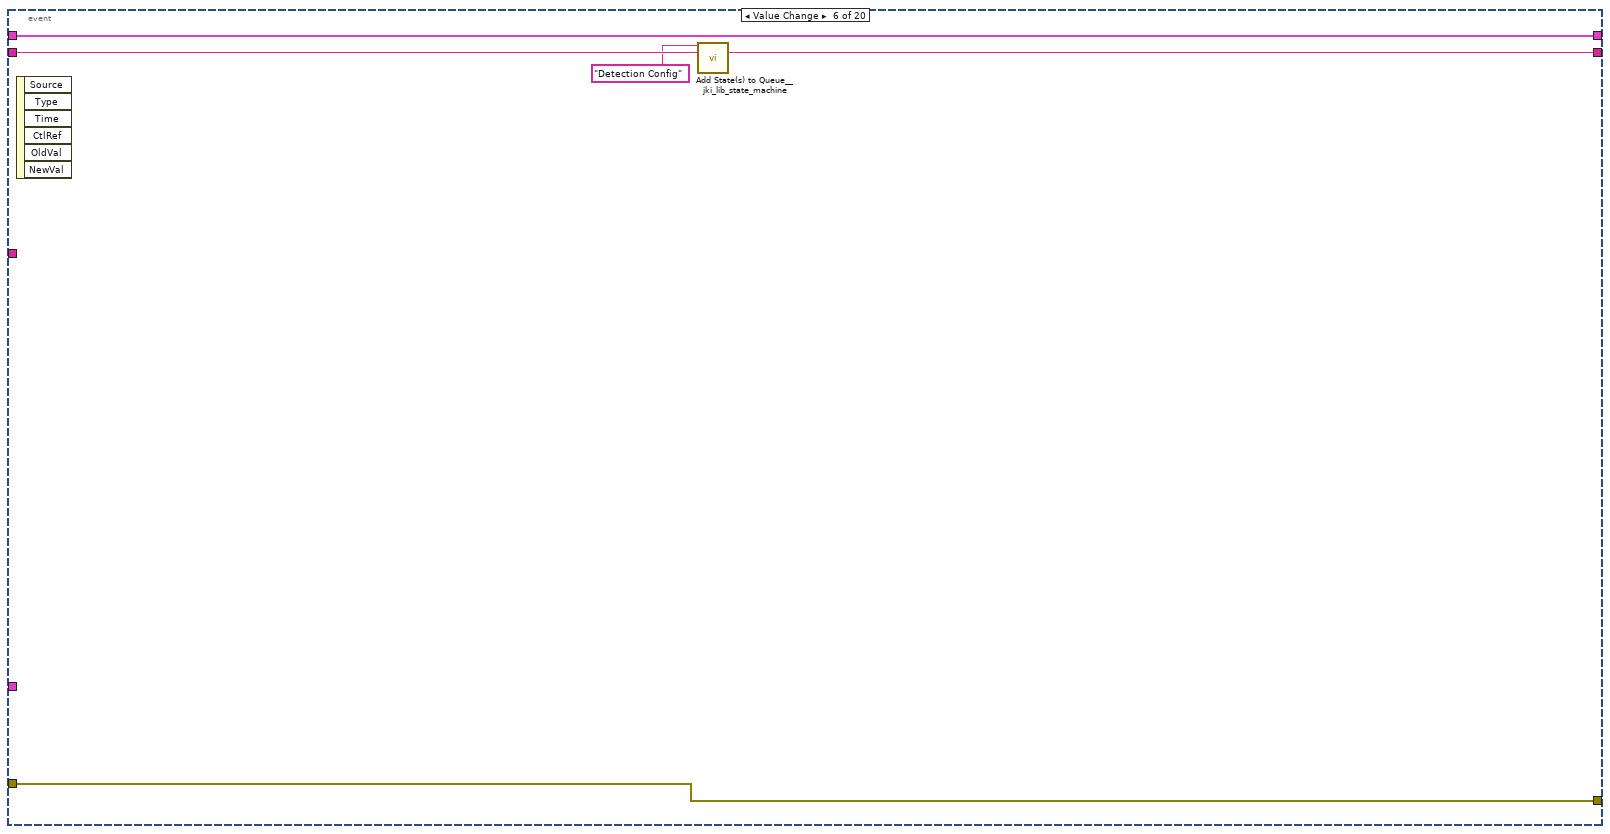
[diagram p14: hidden frame]
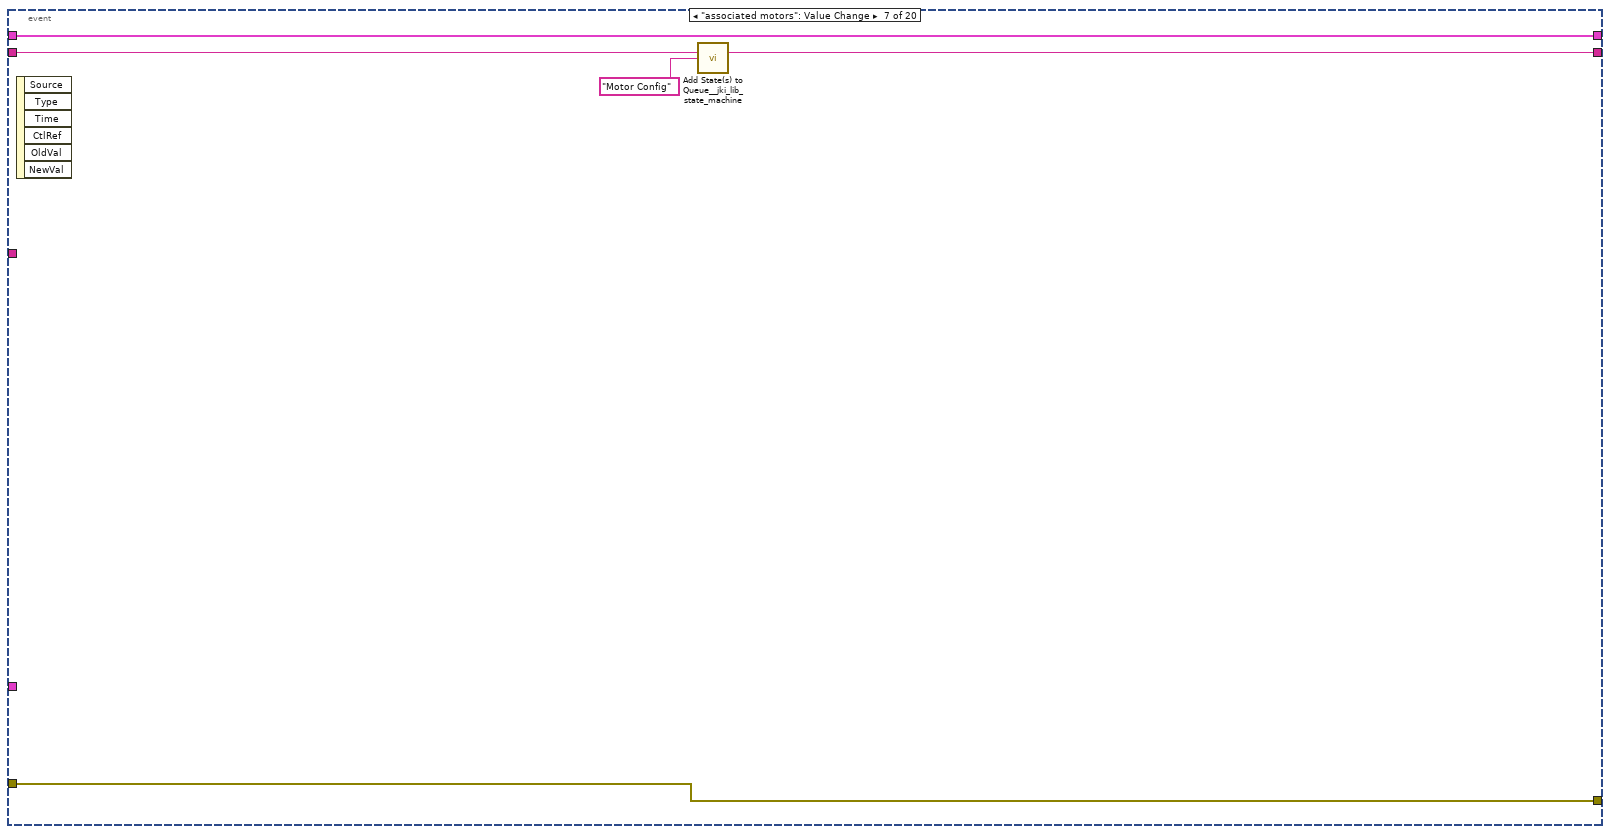
[diagram p15: hidden frame]
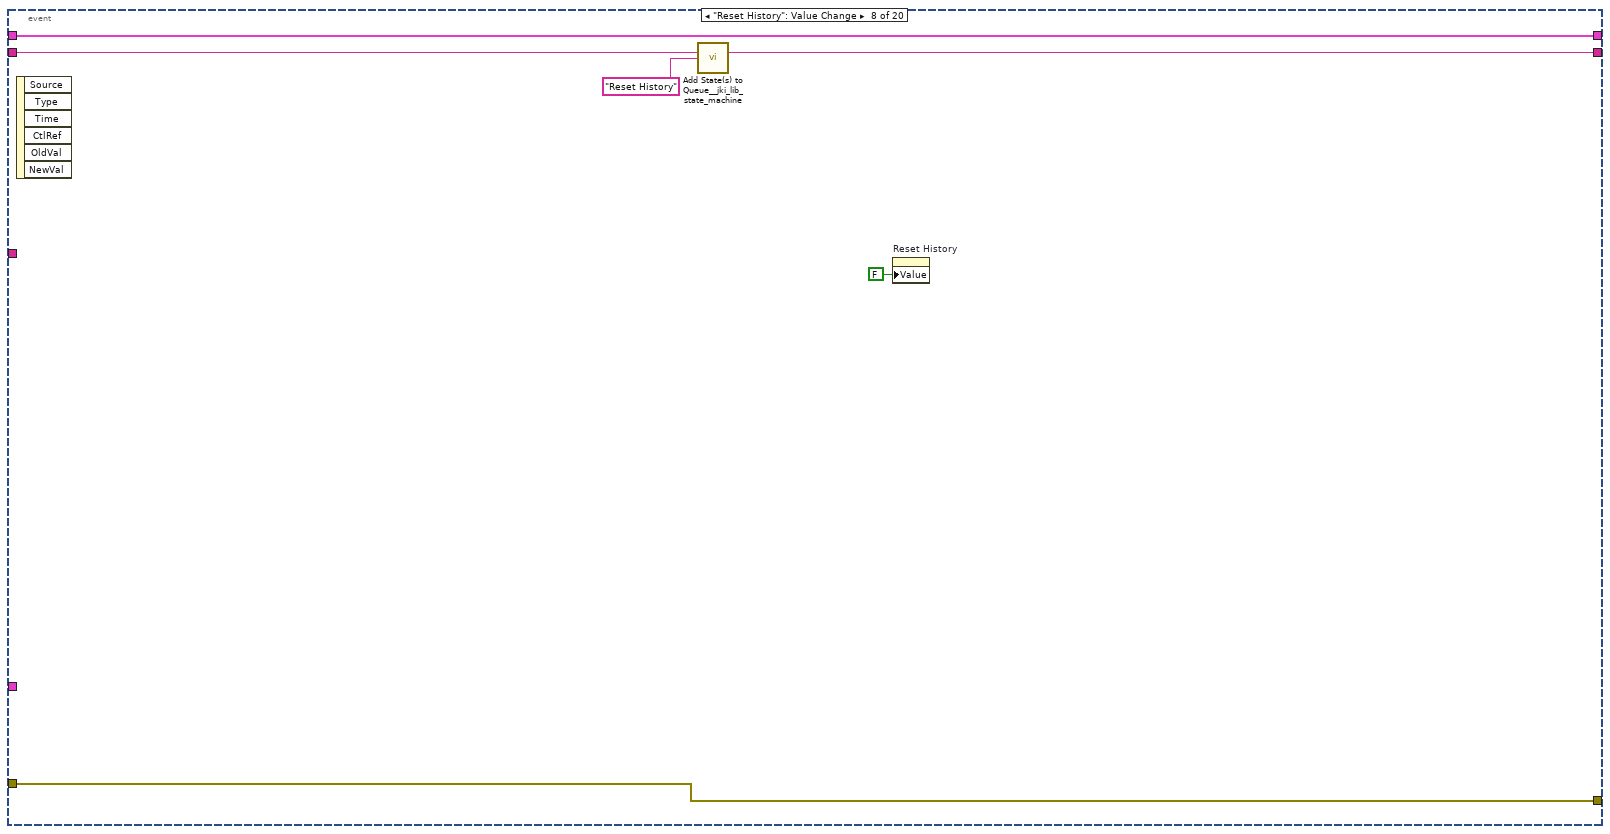
[diagram p16: hidden frame]
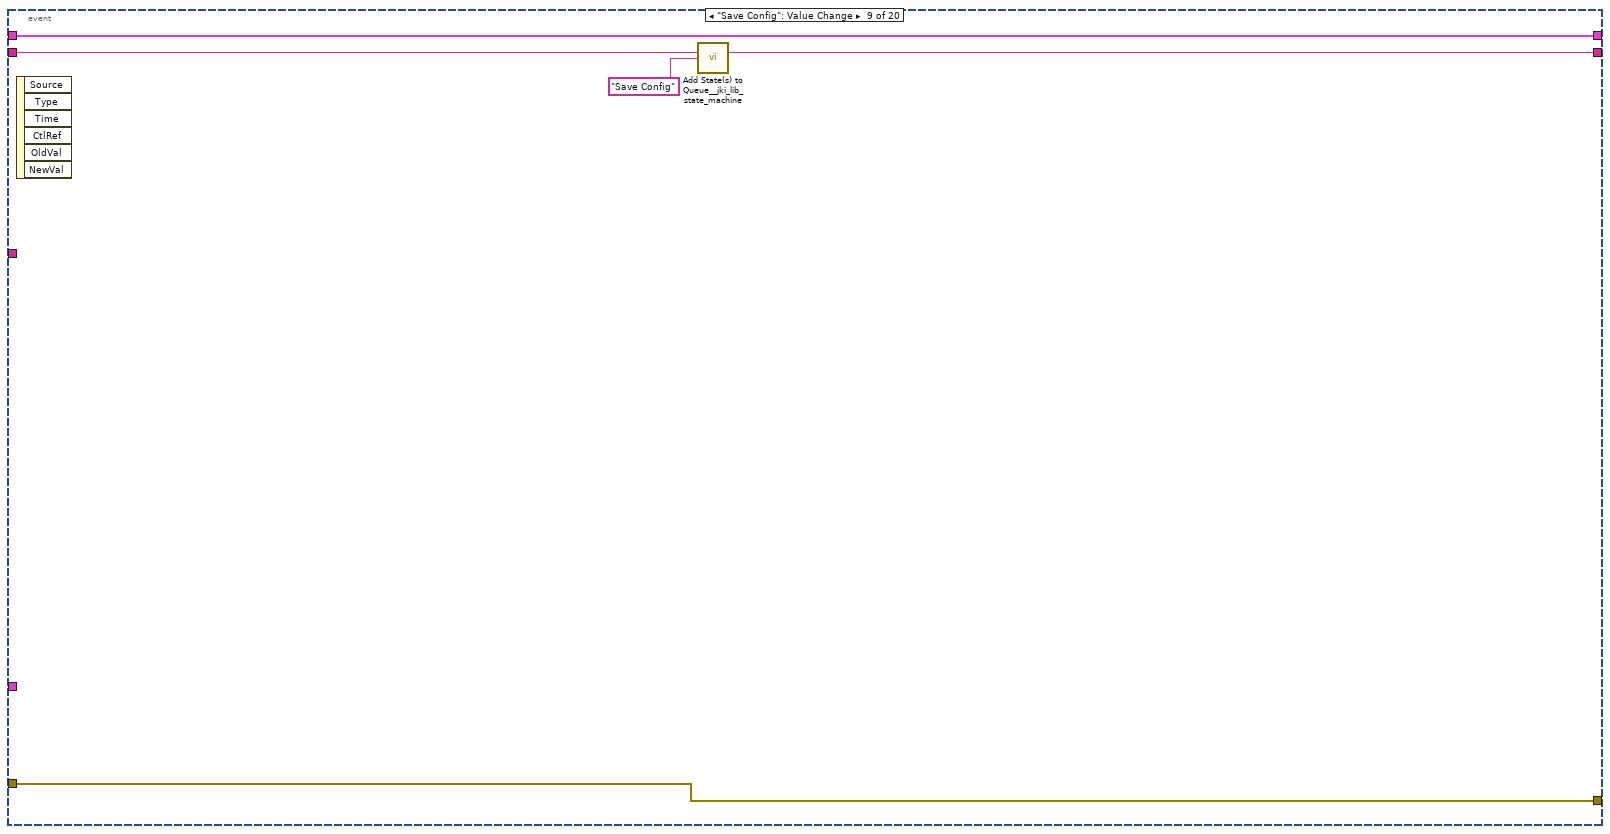
[diagram p17: hidden frame]
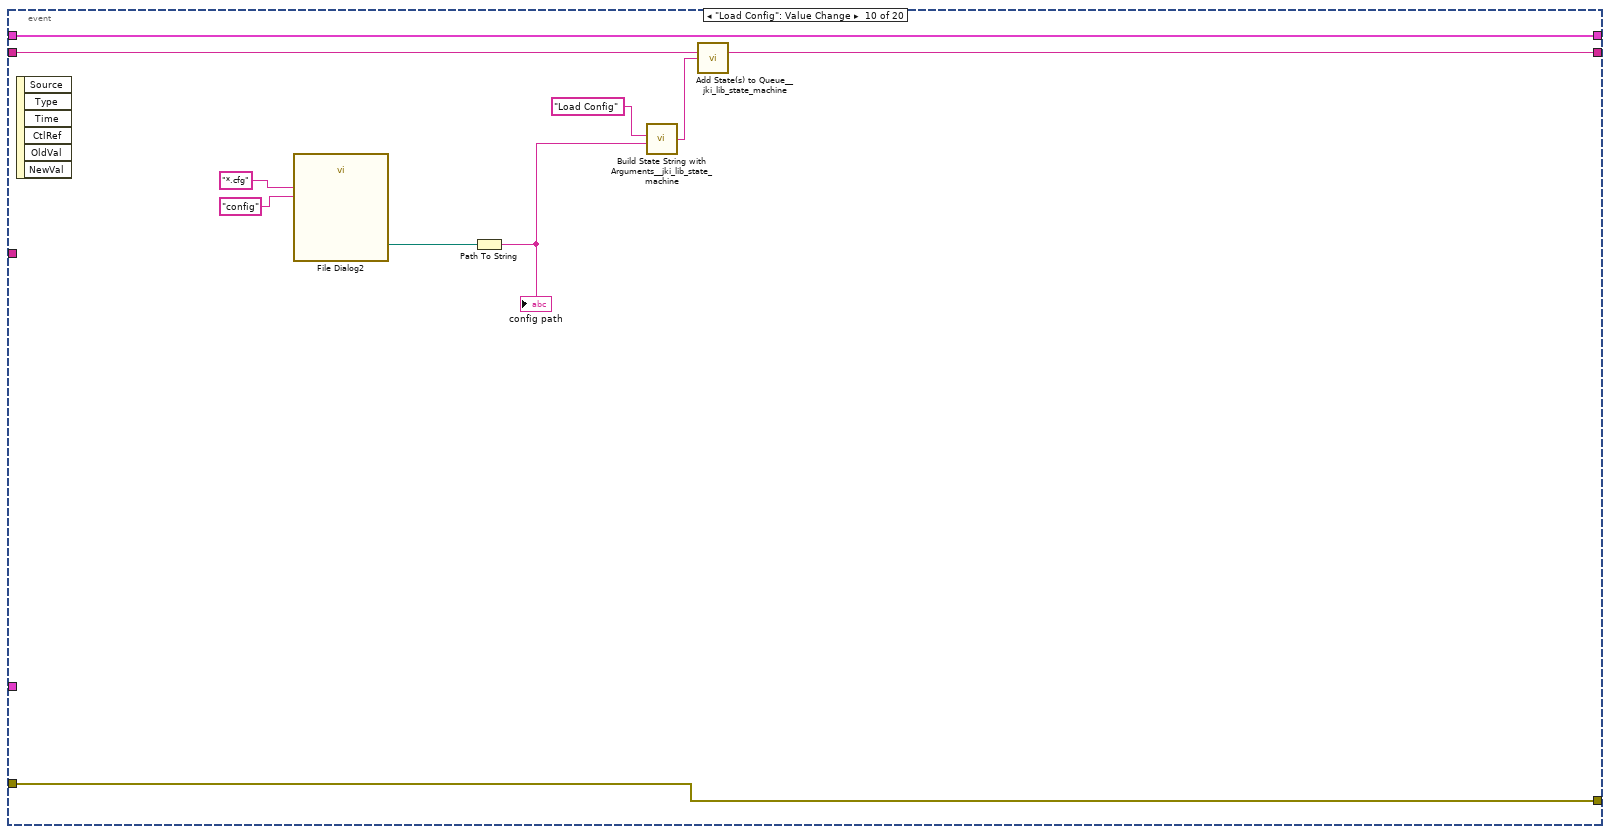
[diagram p18: hidden frame]
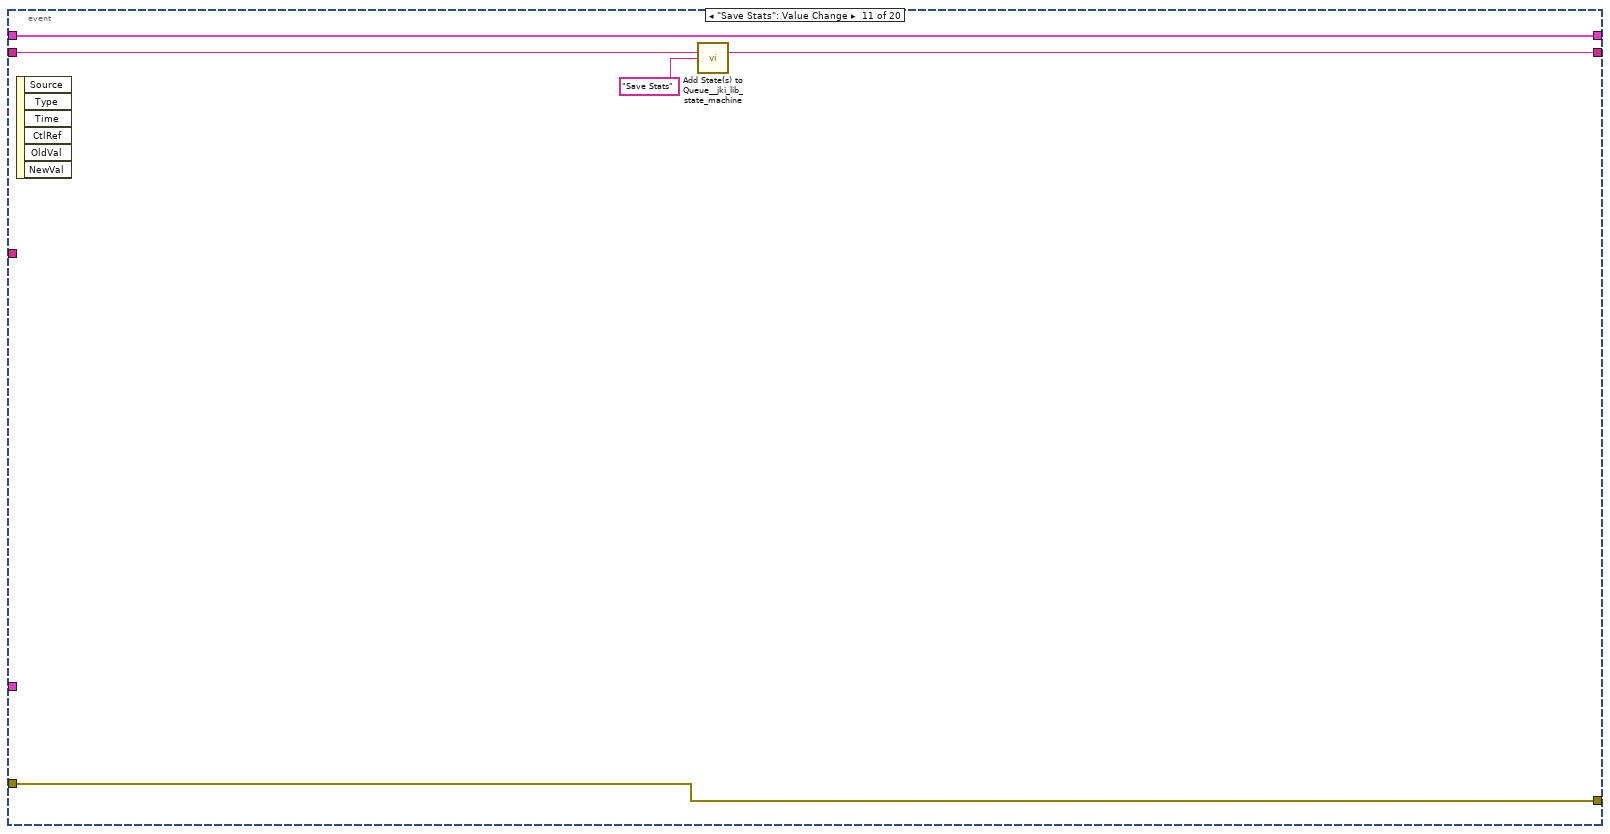
[diagram p19: hidden frame]
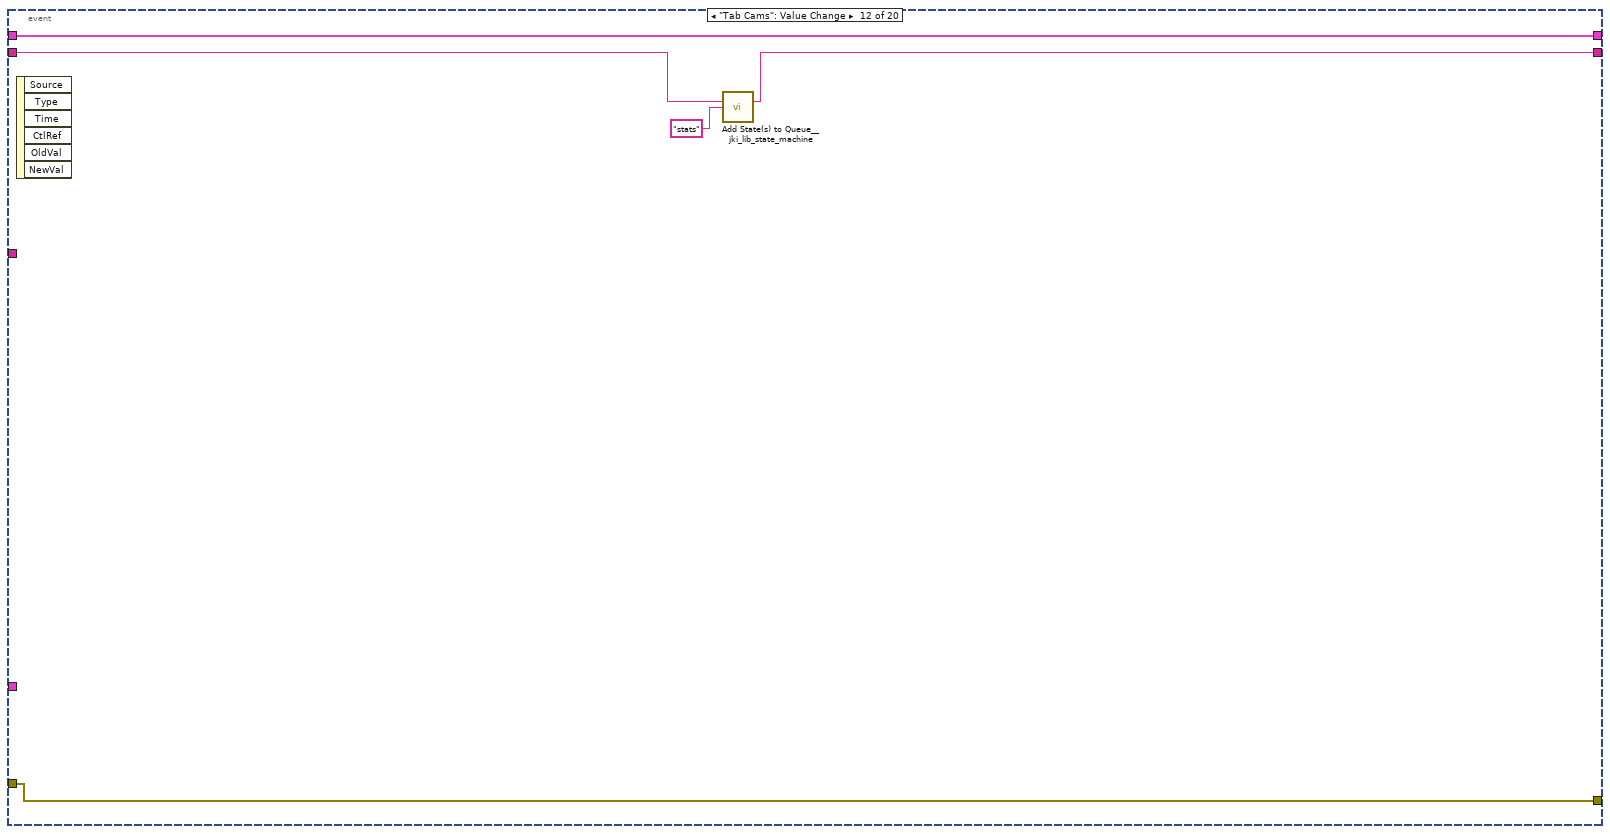
[diagram p20: hidden frame]
diagram:
  n1 = stacked-sequence {
    frame #0 {
      n2 = call <vilib>:"Application Directory.vi"() -> ("Application Directory"=w31:path)
      n3 = Build Path(base path=w31, name or relative path="defaultDevices_ BELLA_BTL.txt") -> (appended path=w29:path)
      "appended path" <- w29
      n4 = call-poly <vilib>:"Read From Spreadsheet File.vi"("file path (dialog if empty)"=w29) -> ("all rows"=w28:string[][])  [unwired: 6 in, 4 out]
      n5 = Index Array(array=w28, index (col) #1=0 ("disabled index (col)"), index (col) #2=1 ("index (col)")) -> (element #1=w25:string[])  [unwired: 2 in, 1 out]
      n6 = Index Array(array=w25, index #1=0 ("index"), index #2=1 ("index"), index #3=2 ("index"), index #4=3 ("index"), index #5=4 ("index"), index #6=5 ("index"), index #7=6 ("index"), index #8=7 ("index"), index #9=8 ("index"), index #10=9 ("index"), index #11=10 ("index"), index #12=11 ("index")) -> (element #1=w12:string, element #2=w11:string, element #3=w10:string, element #4=w9:string, element #5=w8:string, element #6=w7:string, element #7=w6:string, element #8=w5:string, element #9=w4:string, element #10=w3:string, element #11=w2:string, element #12=w1:string)
      n7 = property on="GUIdevice 1" class="Str"("Val(Sgnl)"=w12) -> ()  [unwired: 2 in, 2 out]
      n8 = property on="GUIdevice 2" class="Str"("Val(Sgnl)"=w11) -> ()  [unwired: 2 in, 2 out]
      n9 = property on="GUIdevice 3" class="Str"("Val(Sgnl)"=w10) -> ()  [unwired: 2 in, 2 out]
      n10 = property on="GUIdevice 4" class="Str"("Val(Sgnl)"=w9) -> ()  [unwired: 2 in, 2 out]
      n11 = property on="GUIdevice 5" class="Str"("Val(Sgnl)"=w8) -> ()  [unwired: 2 in, 2 out]
      n12 = property on="GUIdevice 6" class="Str"("Val(Sgnl)"=w7) -> ()  [unwired: 2 in, 2 out]
      n13 = property on="GUIdevice 7" class="Str"("Val(Sgnl)"=w6) -> ()  [unwired: 2 in, 2 out]
      n14 = property on="GUIdevice 8" class="Str"("Val(Sgnl)"=w5) -> ()  [unwired: 2 in, 2 out]
      n15 = property on="GUIdevice 9" class="Str"("Val(Sgnl)"=w4) -> ()  [unwired: 2 in, 2 out]
      n16 = property on="GUIdevice 10" class="Str"("Val(Sgnl)"=w3) -> ()  [unwired: 2 in, 2 out]
      n17 = property on="GUIdevice 11" class="Str"("Val(Sgnl)"=w2) -> ()  [unwired: 2 in, 2 out]
      n18 = property on="GUIdevice 12" class="Str"("Val(Sgnl)"=w1) -> ()  [unwired: 2 in, 2 out]
    }
    frame #1 {
      w40 = path "c:/BP_DATAsd" ("base path")
      w42 = string[] ["M1", "M2", "M4", "M5"] ("elements")
      w46 = T19 0 items=["Grayscale (U8)", "Grayscale (I16)", "Grayscale (SGL)", "Complex (CSG)", "RGB (U32)", "HSL (U32)", "RGB (U64)", "Grayscale (U16)"] ("Image Type")
      # "NOT FOR YOU MOFO"
      n19 = control-ref of="Position.Axis 1::99"() -> (w115:refnum<vi>)
      n20 = control-ref of="Position.Axis 2::99"() -> (w114:refnum<vi>)
      n21 = control-ref of="Position.Axis 1::98"() -> (w39:refnum<vi>)
      n22 = control-ref of="Position.Axis 2::98"() -> (w38:refnum<vi>)
      n23 = control-ref of="Position.Axis 3::98"() -> (w37:refnum<vi>)
      n24 = control-ref of="Position.Axis 1::97"() -> (w36:refnum<vi>)
      n25 = control-ref of="Position.Axis 2::97"() -> (w35:refnum<vi>)
      n26 = control-ref of="Position.Axis 3::97"() -> (w34:refnum<vi>)
      n27 = property on="Motor CCD 1" class="Ring (strict)"("Strings []"=w42) -> ()  [unwired: 2 in, 2 out]
      n28 = property on="Motor CCD 2" class="Ring (strict)"("Strings []"=w42) -> ()  [unwired: 2 in, 2 out]
      n29 = property on="Motor CCD 3" class="Ring (strict)"("Strings []"=w42) -> ()  [unwired: 2 in, 2 out]
      n30 = property on="Motor CCD 4" class="Ring (strict)"("Strings []"=w42) -> ()  [unwired: 2 in, 2 out]
      n31 = property on="Motor CCD 5" class="Ring (strict)"("Strings []"=w42) -> ()  [unwired: 2 in, 2 out]
      n32 = property on="Motor CCD 6" class="Ring (strict)"("Strings []"=w42) -> ()  [unwired: 2 in, 2 out]
      n33 = property on="Motor CCD 7" class="Ring (strict)"("Strings []"=w42) -> ()  [unwired: 2 in, 2 out]
      n34 = property on="Motor CCD 8" class="Ring (strict)"("Strings []"=w42) -> ()  [unwired: 2 in, 2 out]
      n35 = property on="Motor CCD 9" class="Ring (strict)"("Strings []"=w42) -> ()  [unwired: 2 in, 2 out]
      n36 = property on="Motor CCD 10" class="Ring (strict)"("Strings []"=w42) -> ()  [unwired: 2 in, 2 out]
      n37 = property on="Motor CCD 11" class="Ring (strict)"("Strings []"=w42) -> ()  [unwired: 2 in, 2 out]
      n38 = property on="Motor CCD 12" class="Ring (strict)"("Strings []"=w42) -> ()  [unwired: 2 in, 2 out]
      n39 = Build Array(w115, w114, w39, w38, w37, w36, w35, w34) -> (→"motor refs":refnum<vi>[])
      n40 = control-ref of="Target.X::1"() -> (w100:refnum<vi>)
      n41 = control-ref of="Target.Y::1"() -> (w99:refnum<vi>)
      n42 = control-ref of="Target.X::2"() -> (w98:refnum<vi>)
      n43 = control-ref of="Target.Y::2"() -> (w97:refnum<vi>)
      n44 = control-ref of="Target.X::3"() -> (w96:refnum<vi>)
      n45 = control-ref of="Target.Y::3"() -> (w95:refnum<vi>)
      n46 = control-ref of="Target.X::4"() -> (w94:refnum<vi>)
      n47 = control-ref of="Target.Y::4"() -> (w93:refnum<vi>)
      n48 = control-ref of="Target.X::5"() -> (w92:refnum<vi>)
      n49 = control-ref of="Target.Y::5"() -> (w91:refnum<vi>)
      n50 = control-ref of="Target.X::6"() -> (w90:refnum<vi>)
      n51 = control-ref of="Target.Y::6"() -> (w89:refnum<vi>)
      n52 = control-ref of="Target.X::7"() -> (w88:refnum<vi>)
      n53 = control-ref of="Target.Y::7"() -> (w87:refnum<vi>)
      n54 = control-ref of="Target.X::8"() -> (w86:refnum<vi>)
      n55 = control-ref of="Target.Y::8"() -> (w85:refnum<vi>)
      n56 = control-ref of="Target.X::9"() -> (w63:refnum<vi>)
      n57 = control-ref of="Target.Y::9"() -> (w62:refnum<vi>)
      n58 = control-ref of="Target.X::10"() -> (w61:refnum<vi>)
      n59 = control-ref of="Target.Y::10"() -> (w60:refnum<vi>)
      n60 = control-ref of="Target.X::11"() -> (w59:refnum<vi>)
      n61 = control-ref of="Target.Y::11"() -> (w58:refnum<vi>)
      n62 = control-ref of="Target.X::12"() -> (w57:refnum<vi>)
      n63 = control-ref of="Target.Y::12"() -> (w56:refnum<vi>)
      n64 = call "IMAQ Create"("Image Name"="GUIdevice 8", "Image Type"=w46) -> ("New Image"=→"image::8":T9)  [unwired: 3 in, 1 out]
      n65 = call "IMAQ Create"("Image Name"="GUIdevice 9", "Image Type"=w46) -> ("New Image"=→"image::9":T9)  [unwired: 3 in, 1 out]
      n66 = call "IMAQ Create"("Image Name"="GUIdevice 10", "Image Type"=w46) -> ("New Image"=→"image::10":T9)  [unwired: 3 in, 1 out]
      n67 = call "IMAQ Create"("Image Name"="GUIdevice 6", "Image Type"=w46) -> ("New Image"=→"image::6":T9)  [unwired: 3 in, 1 out]
      n68 = call "IMAQ Create"("Image Name"="GUIdevice 7", "Image Type"=w46) -> ("New Image"=→"image::7":T9)  [unwired: 3 in, 1 out]
      n69 = call "IMAQ Create"("Image Name"="GUIdevice 11", "Image Type"=w46) -> ("New Image"=→"image::11":T9)  [unwired: 3 in, 1 out]
      n70 = call "IMAQ Create"("Image Name"="GUIdevice 12", "Image Type"=w46) -> ("New Image"=→"image::12":T9)  [unwired: 3 in, 1 out]
      n71 = call "IMAQ Create"("Image Name"="GUIdevice 2") -> ("New Image"=→"image::2":T9)  [unwired: 4 in, 1 out]
      n72 = call "IMAQ Create"("Image Name"="GUIdevice 4", "Image Type"=w46) -> ("New Image"=→"image::4":T9)  [unwired: 3 in, 1 out]
      n73 = call "IMAQ Create"("Image Name"="GUIdevice 1", "Image Type"=w46) -> ("New Image"=→"image::1":T9)  [unwired: 3 in, 1 out]
      n74 = call "IMAQ Create"("Image Name"="GUIdevice 3", "Image Type"=w46) -> ("New Image"=→"image::3":T9)  [unwired: 3 in, 1 out]
      n75 = call "IMAQ Create"("Image Name"="GUIdevice 5", "Image Type"=w46) -> ("New Image"=→"image::5":T9)  [unwired: 3 in, 1 out]
      n76 = Build Array("GUIdevice 1", "GUIdevice 2", "GUIdevice 3", "GUIdevice 4", "GUIdevice 5", "GUIdevice 6", "GUIdevice 7", "GUIdevice 8", "GUIdevice 9", "GUIdevice 10", "GUIdevice 11", "GUIdevice 12") -> (w74:string[])
      "CCDs" <- w74
      n77 = property on="image::8" class="ImageControl"("Caption.Text"="GUIdevice 8") -> ()  [unwired: 2 in, 2 out]
      n78 = property on="image::10" class="ImageControl"("Caption.Text"="GUIdevice 10") -> ()  [unwired: 2 in, 2 out]
      n79 = property on="image::9" class="ImageControl"("Caption.Text"="GUIdevice 9") -> ()  [unwired: 2 in, 2 out]
      n80 = property on="image::1" class="ImageControl"("Caption.Text"="GUIdevice 1") -> ()  [unwired: 2 in, 2 out]
      n81 = property on="image::2" class="ImageControl"("Caption.Text"="GUIdevice 2") -> ()  [unwired: 2 in, 2 out]
      n82 = property on="image::3" class="ImageControl"("Caption.Text"="GUIdevice 3") -> ()  [unwired: 2 in, 2 out]
      n83 = property on="image::4" class="ImageControl"("Caption.Text"="GUIdevice 4") -> ()  [unwired: 2 in, 2 out]
      n84 = property on="image::5" class="ImageControl"("Caption.Text"="GUIdevice 5") -> ()  [unwired: 2 in, 2 out]
      n85 = property on="image::6" class="ImageControl"("Caption.Text"="GUIdevice 6") -> ()  [unwired: 2 in, 2 out]
      n86 = property on="image::7" class="ImageControl"("Caption.Text"="GUIdevice 7") -> ()  [unwired: 2 in, 2 out]
      n87 = property on="image::11" class="ImageControl"("Caption.Text"="GUIdevice 11") -> ()  [unwired: 2 in, 2 out]
      n88 = property on="image::12" class="ImageControl"("Caption.Text"="GUIdevice 12") -> ()  [unwired: 2 in, 2 out]
      n89 = Array To Cluster(array=w74) -> (cluster=→"Cameras":T20)
      n90 = Bundle("Target.X::1"=w100, "Target.Y::1"=w99) -> (w84:T21)  [unwired: 1 in]
      n91 = Bundle("Target.X::2"=w98, "Target.Y::2"=w97) -> (w83:T22)  [unwired: 1 in]
      n92 = Bundle("Target.X::3"=w96, "Target.Y::3"=w95) -> (w82:T23)  [unwired: 1 in]
      n93 = Bundle("Target.X::4"=w94, "Target.Y::4"=w93) -> (w75:T24)  [unwired: 1 in]
      n94 = Bundle("Target.X::5"=w92, "Target.Y::5"=w91) -> (w81:T25)  [unwired: 1 in]
      n95 = Bundle("Target.X::6"=w90, "Target.Y::6"=w89) -> (w80:T26)  [unwired: 1 in]
      n96 = Bundle("Target.X::7"=w88, "Target.Y::7"=w87) -> (w79:T27)  [unwired: 1 in]
      n97 = Bundle("Target.X::8"=w86, "Target.Y::8"=w85) -> (w78:T28)  [unwired: 1 in]
      n98 = Bundle("Target.X::12"=w57, "Target.Y::12"=w56) -> (w52:T29)  [unwired: 1 in]
      n99 = Bundle("Target.X::9"=w63, "Target.Y::9"=w62) -> (w55:T30)  [unwired: 1 in]
      n100 = Bundle("Target.X::10"=w61, "Target.Y::10"=w60) -> (w54:T31)  [unwired: 1 in]
      n101 = Bundle("Target.X::11"=w59, "Target.Y::11"=w58) -> (w53:T32)  [unwired: 1 in]
      n102 = property on="CCDs" class="Ring (strict)"("Strings []"=w74) -> ()  [unwired: 2 in, 2 out]
      n103 = Build Array(w84, w83, w82, w75, w81, w80, w79, w78, w55, w54, w53, w52) -> (w77:T33)
      n104 = Tick Count (ms)() -> (millisecond timer value=→"millisecond timer value":u32)
      n105 = Get Date/Time In Seconds() -> (seconds since 1Jan1904=w65:timestamp)
      n106 = property on="Feedback Global" class="Bool (strict)"("Value"=FALSE ("Feedback Global")) -> ()  [unwired: 2 in, 2 out]
      n107 = Format Date/Time String(time format string (%c)="%Y%m%d%H%M", seconds (now)=w65) -> (date/time string=w64:string)  [unwired: 1 in]
      n108 = Concatenate Strings(w64, "Beampointing_BTL.tdms" ("string")) -> (w68:string)
      n109 = String To Path(string=w68) -> (path=w67:path)
      n110 = Build Path(base path=w40, name or relative path=w67) -> (appended path=w70:path)
      n111 = call <vilib>:"Add State(s) to Queue__jki_lib_state_machine.vi"("State(s) in (\"\")"="Macro: Initialize") -> ("States Out"=w117:string)  [unwired: 14 in]
      n112 = Create User Event(user event datatype=T13 {"EventEnum"=enum."new data", "Device name"="Device name"} ("New Event")) -> (user event=w125:refnum<user-event>, error out=w127:errorcluster)  [unwired: 1 in]
      "tcp data event" <- w125
      n113 = while "JKI - String-Based Queued State Machine (Basic) v1.0" {
        shift-right: [w148] -> w73
        shift-left: _ -> [w141]
        shift-right: [w151] -> w101
        shift-left: _ -> [w147]
        shift-right: [w150] -> _
        shift-left: w117 -> [w152]
        tunnel: w77 -> [w145]
        tunnel: w74 -> [w143]
        tunnel: [w143] -> w102
        tunnel: w77 -> [w144]
        tunnel: w70 -> [w139]
        tunnel: w40 -> [w138]
        stop <- w149 stop-if-true
        n114 = Unbundle By Name(w141) -> ("active cams"=w140:string[], "Mean Centroid X"=w137:dbl[][], "Mean Centroid Y"=w136:dbl[][], "Mean Size"=w135:dbl[][])
        n115 = call <vilib>:"Parse State Queue__jki_lib_state_machine.vi"("State Queue"=w152, "Error In (no error)"=w147) -> ("Remaining States"=w154:string, "Current State"=w155:string, "Arguments"=w153:string)  [unwired: 11 in]
        "Current State" <- w155
        n116 = case shown="\"Check Move\"" w155 {
          selector: w155 -> [_ _ w503 _ _ _ _ _ _ _ _ _ _ _ _ _ _ _ _ _ _ _ _ _ _ _ _ _ _ _ _ _ _ _ _ _ _ _ _ _ _ _]
          tunnel: w154 -> [w220 w502 w507 w525 w531 w536 w540 w581 w597 w601 w605 w611 w622 w646 w655 w665 w669 w697 w818 w870 w900 w909 w931 w952 w956 w975 w1120 w1288 w1368 w1432 w1507 w1583 w1607 w1622 w1696 w1748 w1758 w1799 w1894 w1920 w1934 w1957]
          tunnel: w153 -> [_ _ _ _ _ _ _ _ _ _ _ w606 w617 _ _ _ _ w673 w771 _ w885 _ _ _ _ w976 _ w1268 w1354 w1418 w1487 w1577 _ _ _ _ _ _ _ _ w1938 _]
          tunnel: w141 -> [w218 w499 w505 w515 w528 w534 w537 _ w592 w598 w603 w609 w616 w643 w652 w657 w666 w688 w808 w868 w881 w905 w923 w945 w953 w964 w1103 w1264 w1364 w1428 w1478 w1579 w1604 w1619 w1692 w1745 w1755 w1773 w1892 w1917 w1937 w1948]
          tunnel: [w217 w500 w509 w523 errorcluster {"status"=FALSE, "code"=0, "source"=""} ("error out") w533 w538 w548 w594 w599 w602 w607 w619 w644 w653 w663 w667 w691 w774 w859 w889 w907 w929 w950 w954 w1005 w1133 w1286 w1366 w1430 w1505 w1572 w1605 w1620 w1693 w1746 w1756 w1766 w1856 w1918 w1932 w1955] -> w151
          tunnel: w147 -> [w216 w500 w508 w523 w527 w533 w538 w549 w595 w599 w602 w608 w620 w644 w653 w663 w667 w692 w772 w860 w888 w907 w929 w950 w954 w1005 w1133 w1286 w1366 w1430 w1505 w1573 w1605 w1620 w1694 w1746 w1756 w1767 w1890 w1918 w1932 w1955]
          tunnel: [w219 w501 w506 w524 w530 w535 w539 w580 w596 w600 w604 w610 w621 w645 w654 w664 w668 w682 w817 w869 w899 w908 w930 w951 w955 w958 w1134 w1287 w1367 w1431 w1506 w1582 w1606 w1621 w1695 w1747 w1757 w1798 w1893 w1919 w1933 w1956] -> w150
          tunnel: [_ _ _ _ _ TRUE _ _ _ _ _ _ _ _ _ _ _ _ _ _ _ _ _ _ _ _ _ _ _ _ _ _ _ _ _ _ _ _ _ _ _ _] -> w149
          tunnel: [w213 w499 w505 w514 w528 w534 w537 w550 w592 w598 w603 w609 w616 w643 w652 w657 w666 w694 w807 w868 w894 w904 w922 w944 w953 w957 w1104 w1264 w1364 w1428 w1478 w1581 w1604 w1619 w1692 w1744 w1755 w1773 w1891 w1917 w1936 w1947] -> w148
          tunnel: "update speed [ms]" -> [w215 _ _ _ _ _ _ _ _ _ _ _ _ _ _ _ _ _ _ _ _ _ _ _ _ _ _ _ _ _ _ _ _ _ _ _ _ _ _ _ _ _]
          tunnel: w145 -> [w212 _ _ _ _ _ _ _ _ _ _ _ _ _ _ _ _ _ _ _ _ _ _ _ _ w997 _ _ _ _ _ _ _ _ _ _ _ _ _ w1902 _ _]
          tunnel: w143 -> [w214 _ _ _ _ _ _ w545 _ _ _ _ _ _ _ _ _ w696 w806 _ w895 _ _ _ _ w968 w1105 w1285 _ _ w1504 w1578 _ w1609 _ _ _ w1772 _ _ _ _]
          tunnel: w139 -> [_ _ _ _ _ _ _ w547 _ _ _ _ _ _ _ _ _ w693 _ _ _ _ _ _ _ _ _ _ _ _ _ _ _ _ _ _ _ _ _ _ _ _]
          tunnel: w138 -> [_ _ _ _ _ _ _ _ _ _ _ _ _ _ _ _ _ _ _ _ _ _ _ _ _ _ _ _ _ _ _ _ _ _ _ _ _ _ w1862 _ _ _]
          frame "", "Idle" {
            # "executes when the state queue is empty"
            n117 = event shown="[0] Timeout" {
              selector: _ -> [_ _ _ _ _ _ _ _ _ _ _ _ _ _ _ _ _ _ _ _]
              dyn-events: _ -> [_ _ _ _ _ _ _ _ _ _ _ _ _ _ _ _ _ _ _ _]
              timeout: w215 -> [_ _ _ _ _ _ _ _ _ _ _ _ _ _ _ _ _ _ _ _]
              tunnel: w220 -> [w225 w349 w364 w389 w394 w399 w404 w410 w415 w425 w430 w432 w444 w456 w468 w473 w478 w484 w488 w498]
              tunnel: [w250 w348 w363 w388 w393 w398 w403 w409 w414 w424 w429 w431 w443 w455 w467 w472 w477 w483 w487 w497] -> w219
              tunnel: w218 -> [w246 w346 w360 w385 w391 w396 w401 w407 w412 w422 w427 w435 w437 w454 w466 w471 w476 w482 w489 w495]
              tunnel: [w261 w347 w362 w387 w392 w397 w402 w408 w413 w423 w428 w434 w442 w449 w461 w470 w475 w481 w486 w496] -> w217
              tunnel: w216 -> [w237 w347 w362 w387 w392 w397 w402 w408 w413 w423 w428 w434 w442 w450 w462 w470 w475 w481 w486 w496]
              tunnel: [w249 w346 w360 w384 w391 w396 w401 w407 w412 w422 w427 w435 w437 w454 w466 w471 w476 w482 w489 w495] -> w213
              tunnel: w214 -> [w242 _ w356 _ _ _ _ _ _ _ _ _ _ _ _ _ _ _ _ _]
              tunnel: w212 -> [_ _ w358 _ _ _ _ _ _ _ _ _ _ _ _ _ _ _ _ _]
              event Timeout {
                n118 = event-data() -> ()  [unwired: 1 in, 1 out]
                n119 = Unbundle By Name(w246) -> ("Centroid X"=w243:dbl[][], "Centroid Y"=w240:dbl[][], "Size"=w238:dbl[][], "detection para"=w233:T3[], "active cams"=w241:string[], "thresholds"=w239:cluster{"Lower value":sgl, "Upper value":sgl}[])
                n120 = Unbundle By Name(w246) -> ("img to avg"=w222:i32, "active ccd"=w245:i32)
                n121 = for {
                  tunnel: w241 -> [w282] mode=indexing
                  tunnel: [w283] -> w229 mode=indexing
                  tunnel: w242 -> [w305]
                  tunnel: w233 -> [w303]
                  tunnel: [w266] -> w228 mode=indexing
                  tunnel: [w301] -> w236 mode=indexing
                  tunnel: [w299] -> w244 mode=indexing
                  tunnel: "autodetect" -> [w293]
                  tunnel: w237 -> [w306]
                  tunnel: [w307] -> w235
                  shift-right: [w290] -> w232
                  shift-left: w239 -> [w292]
                  shift-right: [w277] -> w221
                  shift-left: w243 -> [w279]
                  shift-right: [w273] -> w231
                  shift-left: w240 -> [w275]
                  shift-right: [w267] -> w230
                  shift-left: w238 -> [w269]
                  w271 = 0 ("index")
                  n122 = call-poly <userlib>:"Filter 1D Array__ogtk.vi"("items to filter"=w282, "array"=w305) -> ("filtered item indices"=w304:i32[])  [unwired: 4 in, 1 out]
                  n123 = Index Array(array=w304) -> (element=w268:i32)  [unwired: 1 in]
                  n124 = Index Array(array=w269, index (row)=w268) -> (element=w297:dbl[])  [unwired: 1 in]
                  n125 = Index Array(array=w275, index (row)=w268) -> (element=w298:dbl[])  [unwired: 1 in]
                  n126 = Index Array(array=w292, index=w268) -> (element=w296:cluster{"Lower value":sgl, "Upper value":sgl})
                  n127 = Index Array(array=w279, index (row)=w268) -> (element=w281:dbl[])  [unwired: 1 in]
                  n128 = Index Array(array=w303, index=w268) -> (element=w300:T3)
                  n129 = call "CENTRIOD DETECTION.vi"("Refnum in"=w282, "auto threshold"=w293, "Threshold Range In"=w296, "beam detection para"=w300, "error in (no error)"=w306) -> ("Bounding Rect"=w299:T34, "Particle Reports (Pixels)"=w301:T1, "Threshold Range Out"=w291:cluster{"Lower value":sgl, "Upper value":sgl}, "Centriod"=w308:cluster{"X":dbl, "Y":dbl}, "error out"=w307:errorcluster)  [unwired: 7 in, 3 out]
                  n130 = Unbundle By Name(w308) -> ("X"=w280:dbl, "Y"=w276:dbl)
                  n131 = Empty Array?(array=w301) -> (empty?=w302:bool)
                  n132 = Not(x=w302) -> (.not. x?=w266:bool)
                  n133 = Replace Array Subset(array=w292, new element=w291, index=w268) -> (w290:cluster{"Lower value":sgl, "Upper value":sgl}[])
                  n134 = Unbundle By Name(w299) -> ("Right"=w289:dbl, "Left"=w288:dbl, "Bottom"=w287:dbl, "Top"=w286:dbl)
                  n135 = Subtract(x=w289, y=w288) -> (x-y=w284:dbl)
                  n136 = Subtract(x=w287, y=w286) -> (x-y=w285:dbl)
                  n137 = Multiply(x=w284, y=w285) -> (x*y=w272:dbl)
                  n138 = Insert Into Array(array=w298, index=w271, new element=w276) -> (w274:dbl[])
                  n139 = Insert Into Array(array=w281, index=w271, new element=w280) -> (w278:dbl[])
                  n140 = Insert Into Array(array=w297, index=w271, new element=w272) -> (w270:dbl[])
                  n141 = for {
                    shift-right: [w309] -> w294
                    shift-left: dbl[] [] ("Array 4") -> [w312]
                    tunnel: w274 -> [w310] mode=indexing
                    n142 = Equal To 0?(x=w310) -> (x = 0?=w311:bool)
                    n143 = case shown="False" w311 {
                      tunnel: w312 -> [w315 w316]
                      tunnel: w310 -> [w314 _]
                      tunnel: [w313 w316] -> w309
                      frame False {
                        n144 = Build Array (concatenate)(w315, w314) -> (w313:dbl[])
                      }
                      frame True {
                      }
                    }
                  }
                  n145 = Replace Array Subset(array=w279, new element=w278, index (row)=w268) -> (w277:dbl[][])  [unwired: 1 in]
                  n146 = Replace Array Subset(array=w275, new element=w274, index (row)=w268) -> (w273:dbl[][])  [unwired: 1 in]
                  n147 = Replace Array Subset(array=w269, new element=w270, index (row)=w268) -> (w267:dbl[][])  [unwired: 1 in]
                  n148 = Array Size(array=w294) -> (size(s)=w283:i32)
                }
                "detected" <- w228
                "Box" <- w244
                n149 = Index Array(array=w236, index (row)=w245) -> (element=→"particles":T1)  [unwired: 1 in]
                n150 = call <vilib>:"Clear Errors.vi"("error in (no error)"=w235) -> ("error out"=w261:errorcluster)  [unwired: 5 in, 1 out]
                n151 = local read "Numeric"() -> (w254:dbl)
                n152 = Increment(x=w222) -> (x+1=w251:i32)
                n153 = Greater Or Equal?(x=w254, y=w251) -> (x >= y?=w248:bool)
                n154 = Increment(x=w254) -> (x+1=w253:dbl)
                n155 = Select(t=0.0, s=w248, f=w253) -> (s? t:f=w252:dbl)
                n156 = local write "Numeric"(w252) -> ()
                n157 = Bundle By Name(cluster=w246, "thresholds"=w232) -> (w257:T35)
                n158 = for {
                  tunnel: w229 -> [w338] mode=indexing
                  tunnel: w241 -> [w344] mode=indexing
                  shift-right: [w339] -> w262
                  shift-left: "" ("GUIdevice 7") -> [w342]
                  tunnel: [w333] -> w264 mode=indexing
                  tunnel: "Detection Rate" -> [w337]
                  tunnel: w252 -> [w335]
                  tunnel: w222 -> [w331]
                  n159 = Greater Or Equal?(x=w338, y=w331) -> (x >= y?=w334:bool)
                  n160 = Multiply(x=w337, y=w335) -> (x*y=w336:dbl)
                  n161 = Greater Or Equal?(x=w338, y=w336) -> (x >= y?=w332:bool)
                  n162 = And(x=w334, y=w332) -> (x .and. y?=w333:bool)
                  n163 = Select(t=w344, s=w333, f="") -> (s? t:f=w340:string)
                  n164 = Concatenate Strings(w342, "\t", w340) -> (w339:string)
                }
                n165 = Bundle(0, 1, "Centroid X"=w221) -> (→"Status":cluster{i32, i32, "Centroid X":dbl[][]})  [unwired: 1 in]
                n166 = call <vilib>:"Add State(s) to Queue__jki_lib_state_machine.vi"("State(s) in (\"\")"=w225, "State(s) at Back (\"\")"="Device Ini" ("State(s) at Back (\"\")")) -> ("States Out"=w224:string)  [unwired: 13 in]
                n167 = Bundle By Name(cluster=w257, "Centroid X"=w221, "Centroid Y"=w231, "Size"=w230) -> (w227:T35)
                n168 = Unbundle By Name(w227) -> ("img to avg"=w226:i32)
                n169 = case shown="True" w248 {
                  tunnel: w227 -> [w317 w324]
                  tunnel: [w317 w323] -> w249
                  tunnel: w226 -> [_ w319]
                  frame False {
                  }
                  frame True {
                    n170 = Decrement(x=w319) -> (x-1=w322:i32)
                    n171 = Initialize Array(0.0 ("element"), 12 ("dimension size"), w322) -> (w318:dbl[][])
                    n172 = Bundle By Name(cluster=w324, "Centroid X"=w318, "Centroid Y"=w318, "Size"=w318) -> (w323:T35)
                  }
                }
                n173 = Or Array Elements(Boolean array=w264) -> (logical OR=w263:bool)
                n174 = case shown="True" w263 {
                  tunnel: w262 -> [_ w329]
                  tunnel: w224 -> [w325 w328]
                  tunnel: [w325 w327] -> w250
                  frame False {
                  }
                  frame True {
                    n175 = call <vilib>:"Build State String with Arguments__jki_lib_state_machine.vi"("Arguments (\"\")"=w329, "State"="detected") -> ("State with Arguments"=w326:string)  [unwired: 4 in]
                    n176 = call <vilib>:"Add State(s) to Queue__jki_lib_state_machine.vi"("State(s) in Front (\"\")"=w326, "State(s) in (\"\")"=w328) -> ("States Out"=w327:string)  [unwired: 13 in]
                  }
                }
              }
              event "stop": Value Change {
                # "Exit Button Value Change (pressed) Event\n(this executes Macro: Exit to terminate the VI)"
                n177 = event-data() -> ()  [unwired: 1 in, 6 out]
                n178 = call <vilib>:"Add State(s) to Queue__jki_lib_state_machine.vi"("State(s) in Front (\"\")"="Macro: Exit", "State(s) in (\"\")"=w349) -> ("States Out"=w348:string)  [unwired: 13 in]
              }
              event Value Change {
                n179 = event-data() -> ()  [unwired: 1 in, 6 out]
                n180 = property on="Set Centriod Target" class="Bool (strict)"("Value"=FALSE) -> ()  [unwired: 2 in, 2 out]
                n181 = Unbundle By Name(w360) -> ("active ccd"=w352:i32, "Mean Centroid X"=w351:dbl[][], "Mean Centroid Y"=w350:dbl[][])
                n182 = Index Array(array=w356, index=w352) -> (element=w355:string)
                n183 = Concatenate Strings("Do want to update the target of " ("message"), w355, "?" ("string")) -> (w353:string)
                n184 = Two Button Dialog(message=w353) -> (T button?=w359:bool)  [unwired: 2 in]
                n185 = case shown="True" w359 {
                  tunnel: w358 -> [_ w373]
                  tunnel: w352 -> [_ w372]
                  tunnel: w351 -> [_ w379]
                  tunnel: w350 -> [_ w374]
                  frame False {
                  }
                  frame True {
                    n186 = Index Array(array=w379, index (row)=w372) -> (element=w378:dbl[])  [unwired: 1 in]
                    n187 = Index Array(array=w374, index (row)=w372) -> (element=w375:dbl[])  [unwired: 1 in]
                    n188 = Index Array(array=w373, index=w372) -> (element=w371:T29)
                    n189 = Unbundle By Name(w371) -> ("Target.X::12"=w370:refnum<vi>, "Target.Y::12"=w369:refnum<vi>)
                    n190 = Reverse 1D Array(array=w378) -> (reversed array=w377:dbl[])
                    n191 = Reverse 1D Array(array=w375) -> (reversed array=w376:dbl[])
                    n192 = Index Array(array=w377) -> (element=w368:dbl)  [unwired: 1 in]
                    n193 = Index Array(array=w376) -> (element=w366:dbl)  [unwired: 1 in]
                    n194 = To Unsigned Word Integer(number=w366) -> (unsigned 16bit integer=w365:u16)
                    n195 = To Unsigned Word Integer(number=w368) -> (unsigned 16bit integer=w367:u16)
                    n196 = disable-structure shown="Enabled" {
                      disable-tunnel: w370 -> [w383 _]
                      disable-tunnel: w367 -> [w382 _]
                      disable-tunnel: w369 -> [w381 _]
                      disable-tunnel: w365 -> [w380 _]
                      frame Enabled {
                        n197 = property class="DigNum (strict)"(reference=w383, "Val(Sgnl)"=w382) -> ()  [unwired: 1 in, 2 out]
                        n198 = property class="DigNum (strict)"(reference=w381, "Val(Sgnl)"=w380) -> ()  [unwired: 1 in, 2 out]
                      }
                      frame Disabled {
                      }
                    }
                  }
                }
                n199 = call <vilib>:"Add State(s) to Queue__jki_lib_state_machine.vi"("State(s) in (\"\")"=w364) -> ("States Out"=w363:string)  [unwired: 14 in]
              }
              event "Feedback Global": Value Change {
                # "Exit Button Value Change (pressed) Event\n(this executes Macro: Exit to terminate the VI)"
                n200 = event-data() -> ("NewVal"=w386:bool)  [unwired: 1 in, 5 out]
                n201 = call <vilib>:"Add State(s) to Queue__jki_lib_state_machine.vi"("State(s) in (\"\")"=w389) -> ("States Out"=w388:string)  [unwired: 14 in]
                n202 = Bundle By Name(cluster=w385, "Feedback global"=w386) -> (w384:T35)
              }
              event Value Change {
                n203 = event-data() -> ()  [unwired: 1 in, 6 out]
                n204 = call <vilib>:"Add State(s) to Queue__jki_lib_state_machine.vi"("State(s) in Front (\"\")"="Move Config", "State(s) in (\"\")"=w394) -> ("States Out"=w393:string)  [unwired: 13 in]
              }
              event Value Change {
                n205 = event-data() -> ()  [unwired: 1 in, 6 out]
                n206 = call <vilib>:"Add State(s) to Queue__jki_lib_state_machine.vi"("State(s) in Front (\"\")"="Detection Config", "State(s) in (\"\")"=w399) -> ("States Out"=w398:string)  [unwired: 13 in]
              }
              event "associated motors": Value Change {
                n207 = event-data() -> ()  [unwired: 1 in, 6 out]
                n208 = call <vilib>:"Add State(s) to Queue__jki_lib_state_machine.vi"("State(s) in (\"\")"=w404, "State(s) at Back (\"\")"="Motor Config" ("State(s) at Back (\"\")")) -> ("States Out"=w403:string)  [unwired: 13 in]
              }
              event "Reset History": Value Change {
                n209 = event-data() -> ()  [unwired: 1 in, 6 out]
                n210 = call <vilib>:"Add State(s) to Queue__jki_lib_state_machine.vi"("State(s) in (\"\")"=w410, "State(s) at Back (\"\")"="Reset History" ("State(s) at Back (\"\")")) -> ("States Out"=w409:string)  [unwired: 13 in]
                n211 = property on="Reset History" class="Bool (strict)"("Value"=FALSE ("Reset History")) -> ()  [unwired: 2 in, 2 out]
              }
              event "Save Config": Value Change {
                n212 = event-data() -> ()  [unwired: 1 in, 6 out]
                n213 = call <vilib>:"Add State(s) to Queue__jki_lib_state_machine.vi"("State(s) in (\"\")"=w415, "State(s) at Back (\"\")"="Save Config" ("State(s) at Back (\"\")")) -> ("States Out"=w414:string)  [unwired: 13 in]
              }
              event "Load Config": Value Change {
                n214 = event-data() -> ()  [unwired: 1 in, 6 out]
                n215 = call "File Dialog2"("pattern (all files)"="*.cfg", "pattern label"="config") -> ("selected path"=w419:path)  [unwired: 10 in, 3 out]
                n216 = Path To String(path=w419) -> (string=w417:string)
                "config path" <- w417
                n217 = call <vilib>:"Build State String with Arguments__jki_lib_state_machine.vi"("Arguments (\"\")"=w417, "State"="Load Config" ("State(s) at Back (\"\")")) -> ("State with Arguments"=w416:string)  [unwired: 4 in]
                n218 = call <vilib>:"Add State(s) to Queue__jki_lib_state_machine.vi"("State(s) in (\"\")"=w425, "State(s) at Back (\"\")"=w416) -> ("States Out"=w424:string)  [unwired: 13 in]
              }
              event "Save Stats": Value Change {
                n219 = event-data() -> ()  [unwired: 1 in, 6 out]
                n220 = call <vilib>:"Add State(s) to Queue__jki_lib_state_machine.vi"("State(s) in (\"\")"=w430, "State(s) at Back (\"\")"="Save Stats" ("State(s) at Back (\"\")")) -> ("States Out"=w429:string)  [unwired: 13 in]
              }
              event "Tab Cams": Value Change {
                n221 = event-data() -> ()  [unwired: 1 in, 6 out]
                n222 = call <vilib>:"Add State(s) to Queue__jki_lib_state_machine.vi"("State(s) in (\"\")"=w432, "State(s) at Back (\"\")"="stats" ("State")) -> ("States Out"=w431:string)  [unwired: 13 in]
              }
              event "active CCDs": Value Change {
                n223 = event-data() -> ("NewVal"=w441:i32)  [unwired: 1 in, 5 out]
                n224 = Unbundle By Name(w437) -> ("active cams"=w436:string[])
                n225 = Index Array(array=w436, index=w441) -> (element=w439:string)
                n226 = call <vilib>:"Build State String with Arguments__jki_lib_state_machine.vi"("Arguments (\"\")"=w439, "State"="active" ("State(s) at Back (\"\")")) -> ("State with Arguments"=w438:string)  [unwired: 4 in]
                n227 = call <vilib>:"Add State(s) to Queue__jki_lib_state_machine.vi"("State(s) in (\"\")"=w444, "State(s) at Back (\"\")"=w438) -> ("States Out"=w443:string)  [unwired: 13 in]
              }
              event "Left", "Right": Value Change {
                n228 = event-data() -> ("CtlRef"=w453:refnum<vi>)  [unwired: 1 in, 5 out]
                n229 = property class="Bool (strict)"(reference=w453, error in=w450) -> (reference out=w452:refnum<vi>, error out=w451:errorcluster, "Label.Text"=w447:string)
                n230 = property class="Bool (strict)"(reference=w452, error in=w451, "Value"=FALSE) -> (error out=w449:errorcluster)  [unwired: 1 out]
                n231 = call <vilib>:"Build State String with Arguments__jki_lib_state_machine.vi"("Arguments (\"\")"=w447, "State"="ManMove X") -> ("State with Arguments"=w446:string)  [unwired: 4 in]
                n232 = call <vilib>:"Add State(s) to Queue__jki_lib_state_machine.vi"("State(s) in (\"\")"=w456, "State(s) at Back (\"\")"=w446) -> ("States Out"=w455:string)  [unwired: 13 in]
              }
              event "Up", "Down": Value Change {
                n233 = event-data() -> ("CtlRef"=w465:refnum<vi>)  [unwired: 1 in, 5 out]
                n234 = property class="Bool (strict)"(reference=w465, error in=w462) -> (reference out=w464:refnum<vi>, error out=w463:errorcluster, "Label.Text"=w459:string)
                n235 = property class="Bool (strict)"(reference=w464, error in=w463, "Value"=FALSE) -> (error out=w461:errorcluster)  [unwired: 1 out]
                n236 = call <vilib>:"Build State String with Arguments__jki_lib_state_machine.vi"("Arguments (\"\")"=w459, "State"="ManMove Y") -> ("State with Arguments"=w458:string)  [unwired: 4 in]
                n237 = call <vilib>:"Add State(s) to Queue__jki_lib_state_machine.vi"("State(s) in (\"\")"=w468, "State(s) at Back (\"\")"=w458) -> ("States Out"=w467:string)  [unwired: 13 in]
              }
              event "Center": Value Change {
                n238 = event-data() -> ()  [unwired: 1 in, 6 out]
                n239 = call <vilib>:"Add State(s) to Queue__jki_lib_state_machine.vi"("State(s) in (\"\")"=w473, "State(s) at Back (\"\")"="Center" ("State(s) at Back (\"\")")) -> ("States Out"=w472:string)  [unwired: 13 in]
              }
              event "new tdms": Value Change {
                n240 = event-data() -> ()  [unwired: 1 in, 6 out]
                n241 = call <vilib>:"Add State(s) to Queue__jki_lib_state_machine.vi"("State(s) in (\"\")"=w478, "State(s) at Back (\"\")"="newtdms" ("State(s) at Back (\"\")")) -> ("States Out"=w477:string)  [unwired: 13 in]
              }
              event "device ini": Value Change {
                n242 = event-data() -> ()  [unwired: 1 in, 6 out]
                n243 = property on="device ini" class="Bool (strict)"("Value"=FALSE ("test")) -> ()  [unwired: 2 in, 2 out]
                n244 = call <vilib>:"Add State(s) to Queue__jki_lib_state_machine.vi"("State(s) in (\"\")"=w484, "State(s) at Back (\"\")"="Device Ini" ("State(s) at Back (\"\")")) -> ("States Out"=w483:string)  [unwired: 13 in]
              }
              event "img to avg": Value Change {
                n245 = event-data() -> ("NewVal"=w490:i32)  [unwired: 1 in, 5 out]
                n246 = Number To Decimal String(number=w490) -> (decimal integer string=w492:string)  [unwired: 1 in]
                n247 = call <vilib>:"Build State String with Arguments__jki_lib_state_machine.vi"("Arguments (\"\")"=w492, "State"="ImgToAvg" ("State(s) at Back (\"\")")) -> ("State with Arguments"=w485:string)  [unwired: 4 in]
                n248 = call <vilib>:"Add State(s) to Queue__jki_lib_state_machine.vi"("State(s) in Front (\"\")"=w485, "State(s) in (\"\")"=w488) -> ("States Out"=w487:string)  [unwired: 13 in]
              }
              event Panel Close? {
                # "Discard the event because we'll close the front panel ourselves in Macro: Exit"
                # "Close Panel button (pressed) Event\n(this executes Macro: Exit to terminate the VI)"
                n249 = event-data() -> ()  [unwired: 1 in, 1 out]
                n250 = call <vilib>:"Add State(s) to Queue__jki_lib_state_machine.vi"("State(s) in Front (\"\")"="Macro: Exit", "State(s) in (\"\")"=w498) -> ("States Out"=w497:string)  [unwired: 13 in]
                n251 = event-data("Discard?"=TRUE) -> ()  [unwired: 1 in, 1 out]
              }
            }
          }
          frame "---------- Core ----------" {
            # "Do not put any code in this frame.\n(it is a separator no-op)"
            n252 = call <vilib>:"Add State(s) to Queue__jki_lib_state_machine.vi"("State(s) in (\"\")"=w502) -> ("States Out"=w501:string)  [unwired: 14 in]
          }
          frame Default {
            w512 = 42 items=["No error", "Argument error", "Memory is full", "Out of zone", "End of file", "File already open", "Generic file I/O error", "File not found", "File permission error", "Disk is full", "Duplicate path", "Too many files open", "System feature not enabled", "Resource file not found", "Cannot add resource", "Resource not found", "Image not found", "Image memory error", "Pen does not exist", "Config type invalid", "Config token not found", "Config parse error", "Config memory error", "Bad external code format", "Bad external code offset", "External code not present", "Null window", "Destroy window error", "Null menu", "Print aborted", "Bad print record", "Print driver error", "Windows error during printing", "Memory error during printing", "Print dialog error", "Generic print error", "Invalid device refnum", "Device not found", "Device parameter error", "Device unit error", "Cannot open device", "Device call aborted", "Generic error", "Cancelled by user", "Object ID too low", "Object ID too high", "Object not in heap", "Unknown heap", "Unknown object (invalid DefProc)", "Unknown object (DefProc not in table)", "Message out of range", "Invalid (null) method", "Unknown message", "Manager call not supported", "Bad address", "Network operation in progress", "Network operation timed out", "Connection is busy", "Network attribute not supported", "Network error", "Address in use", "System out of memory", "Connection aborted", "Connection refused", "Not connected", "Already connected", "Connection closed", "Initialization error (interapplication manager)", "Bad occurrence", "Wait on unbound occurrence handler", "Occurrence queue overflow", "Datalog type conflict", "Unused", "Unrecognized type (interapplication manager)", "Memory corrupt", "Failed to make temporary DLL", "Old CIN version", "Drag socket not found", "Failed to load drop-object", "Failed to register OLE object", "Failed to release OLE object", "Format specifier type mismatch", "Unknown format specifier", "Too few format specifiers", "Too many format specifiers", "Scan failed", "Newer CIN version", "Error converting to variant", "Runtime menu error", "Password tampered", "Variant attribute not found", "Incompatible variant data type", "Event data is not available", "Event Store is not present", "Occurrence is not found", "Event Queue is not created", "Event info is not available", "Refnum passed is NULL", "Error retrieving Class GUID", "Error retrieving CoClass GUID", "Error retrieving TypeLib GUID.", "Bad built application magic bytes.", "Specific driver is different from the specific driver associated with the Logical Name.", "There is no session opened to the class driver.", "Max Error", "MAX - Error with config objects", "MAX - Error loading configuration", "MAX - Group not supported"]
            # "Current State"
            # "Do not delete, rename, or modify this frame.\n(this is used to capture unhandled states and typos)"
            # "Handle mistyped state name (developer tool)"
            n253 = Format Into String(format string="Software Exception: Unhandled State \"%s\"." ("message"), error in=w508, w503) -> (resulting string=w511:string, error out=w510:errorcluster)  [unwired: 1 in]
            n254 = call <vilib>:"Error Cluster From Error Code.vi"("show call chain? (False)"=TRUE, "error in (no error)"=w510, "error message (\"\")"=w511, "error code (0)"=w512) -> ("error out"=w509:errorcluster)  [unwired: 5 in]
            n255 = call <vilib>:"Add State(s) to Queue__jki_lib_state_machine.vi"("State(s) in (\"\")"=w507) -> ("States Out"=w506:string)  [unwired: 14 in]
          }
          frame "Initialize Core Data" {
            # "Do not delete, rename, or modify this frame.\n(this is used to determine panel behavior on exit)"
            # "originally closed?"
            # "exe?"
            # "If panel starts closed or is an EXE, then close it when we exit"
            n256 = property class="VI"() -> ("Front Panel.Open"=w522:bool)  [unwired: 2 in, 2 out]
            n257 = property class="App"() -> ("App.Kind"=w521:T14)  [unwired: 2 in, 2 out]
            n258 = control-ref of="Current VI Reference"() -> (w516:refnum<vi>)
            n259 = Not(x=w522) -> (.not. x?=w519:bool)
            n260 = Equal?(x=w521, y=T14."Run Time System" ("Application:Kind")) -> (x = y?=w518:bool)
            n261 = Or(x=w519, y=w518) -> (x .or. y?=w517:bool)
            n262 = Bundle By Name(cluster=w515, "Core.Current VI Reference"=w516, "Core.Close Panel on Exit?"=w517) -> (w514:T35)
            n263 = call <vilib>:"Add State(s) to Queue__jki_lib_state_machine.vi"("State(s) in (\"\")"=w525) -> ("States Out"=w524:string)  [unwired: 14 in]
          }
          frame "Error Handler" {
            # "Unhandled Error -- Display it"
            # "Handle any errors here.\nYou can also output any states to clean-up after errors occur"
            # "Clear error"
            n264 = call <vilib>:"General Error Handler.vi"("error in (no error)"=w527) -> ()  [unwired: 10 in, 5 out]
            n265 = call <vilib>:"Add State(s) to Queue__jki_lib_state_machine.vi"("State(s) in Front (\"\")"="/* Post Error States", "State(s) in (\"\")"=w531) -> ("States Out"=w530:string)  [unwired: 13 in]
          }
          frame "Exit" {
            # "Do not put any code in this frame.\n(No errors that occur here will be handled.)"
            n266 = call <vilib>:"Add State(s) to Queue__jki_lib_state_machine.vi"("State(s) in (\"\")"=w536) -> ("States Out"=w535:string)  [unwired: 14 in]
          }
          frame "---------- Data ----------" {
            # "Do not put any code in this frame.\n(It is a separator no-op. You can make a copy of this frame to create a new Data frame)"
            n267 = call <vilib>:"Add State(s) to Queue__jki_lib_state_machine.vi"("State(s) in (\"\")"=w540) -> ("States Out"=w539:string)  [unwired: 14 in]
          }
          frame "Data: Initialize" {
            w541 = dbl[] [0.0, 0.0, 0.0, 0.0, 0.0, 0.0, 0.0, 0.0, 0.0, 0.0, 0.0, 0.0]  # steps speed Y
            w542 = dbl[] [0.0, 0.0, 0.0, 0.0, 0.0, 0.0, 0.0, 0.0, 0.0, 0.0, 0.0, 0.0]  # steps speed X
            w546 = bool[] [FALSE, FALSE, FALSE, FALSE, TRUE, TRUE, TRUE, FALSE, FALSE, FALSE, FALSE, FALSE]  # detected
            w556 = bool[] [FALSE, FALSE, FALSE, FALSE, FALSE, FALSE, FALSE, FALSE, FALSE, FALSE, FALSE, TRUE]  # speedmode Y
            w557 = bool[] [FALSE, FALSE, FALSE, FALSE, FALSE, FALSE, FALSE, FALSE, FALSE, FALSE, FALSE, TRUE]  # speedmode X
            w559 = cluster{"Lower value":sgl, "Upper value":sgl}[] [{"Lower value"=93.0, "Upper value"=255.0}, {"Lower value"=105.0, "Upper value"=255.0}, {"Lower value"=0.0, "Upper value"=255.0}, {"Lower value"=127.0, "Upper value"=255.0}, {"Lower value"=0.0, "Upper value"=255.0}, {"Lower value"=0.0, "Upper value"=255.0}, {"Lower value"=0.0, "Upper value"=255.0}, {"Lower value"=0.0, "Upper value"=255.0}, {"Lower value"=0.0, "Upper value"=255.0}, {"Lower value"=0.0, "Upper value"=255.0}, {"Lower value"=0.0, "Upper value"=255.0}, {"Lower value"=0.0, "Upper value"=255.0}]  # thresholds
            w566 = FALSE  # Feedback global
            w568 = 0  # active ccd
            w552 = 6  # img to avg
            w579 = T36 {"Current VI Reference"=refnum, "Close Panel on Exit?"=FALSE}  # Core
            # "Initialize the shift-register data, here.\n(data names are defined by what you wire into the bundle function)"
            n268 = disable-structure shown="Disabled" {
              disable-tunnel: w549 -> [w591 _]
              disable-tunnel: [w590 _] -> w548
              disable-tunnel: w547 -> [w589 _]
              disable-tunnel: [w588 _] -> _
              disable-tunnel: w545 -> [w582 _]
              frame Disabled {
                n269 = TDMS Open(6:FALSE ("disable buffering (T)"), 7:enum16{"1.0", "2.0"}."2.0" ("file format version (2.0)"), 8:w591, 10:T15."create or replace" ("operation"), 11:w589) -> (0:w586:errorcluster, 3:w587:refnum<k34>)  [unwired: 2 in]
                n270 = call "TDMSbuffersize.vi"("error in (no error)"=w586, "group names"=w582, "Data Value Reference in"=w587) -> ("error out"=w590:errorcluster, "Data Value Reference out"=w588:refnum<k34>)  [unwired: 7 in]
              }
              frame Enabled {
              }
            }
            n271 = call <vilib>:"Add State(s) to Queue__jki_lib_state_machine.vi"("State(s) in Front (\"\")"="newtdms" ("State(s) in Front (\"\")"), "State(s) in (\"\")"=w581) -> ("States Out"=w580:string)  [unwired: 13 in]
            n272 = Bundle("Core"=w579, "detection para"="detection para", "thresholds"=w559, "Centroid X"="Centroid X", "Centroid Y"="Centroid Y", "img to avg"=w552, "Mean Centroid X"="Mean Centroid X", "Mean Centroid Y"="Mean Centroid Y", "Offset X"="Offset X", "Offset Y"="Offset Y", "Offset X stats"="Offset X stats", "Offset Y stats"="Offset Y stats", "Size"="Size", "Mean Size"="Mean Size", "Time"="Time", "move properties"="move properties", "active axis refs 2"="active axis refs 2", "active ccd"=w568, "Feedback global"=w566, "Motor X"="Motor X", "Motor Y"="Motor Y", "active cams"="active cams", "Data Value Reference out"=refnum<k34> refnum, "active man refs"="active man refs", "detected"=w546, "speedmode X"=w557, "speedmode Y"=w556, "steps speed X"=w542, "steps speed Y"=w541) -> (w551:T35)  [unwired: 1 in]
            n273 = Initialize Array(0.0 ("element"), 12 ("dimension size"), w552) -> (w555:dbl[][])
            n274 = Bundle By Name(cluster=w551, "Centroid X"=w555, "Centroid Y"=w555, "Size"=w555) -> (w550:T35)
          }
          frame "Data: Cleanup" {
            # "Cleanup any data and references, here.\n(this is called automatically, by the Macro: Exit)"
            n275 = Unbundle By Name(w592) -> ("Core.Current VI Reference"=w593:refnum<vi>)
            n276 = Close Reference(reference=w593, error in (no error)=w595) -> (error out=w594:errorcluster)
            n277 = call <vilib>:"Add State(s) to Queue__jki_lib_state_machine.vi"("State(s) in (\"\")"=w597) -> ("States Out"=w596:string)  [unwired: 14 in]
          }
          frame "---------- UI ----------" {
            # "Do not put any code in this frame.\n(It is a separator no-op. You can make a copy of this frame to create a new UI frame)"
            n278 = call <vilib>:"Add State(s) to Queue__jki_lib_state_machine.vi"("State(s) in (\"\")"=w601) -> ("States Out"=w600:string)  [unwired: 14 in]
          }
          frame "UI: Initialize" {
            # "Initialize the User Interface, here.\n(this is called automatically, by the Macro: Init)"
            n279 = call <vilib>:"Add State(s) to Queue__jki_lib_state_machine.vi"("State(s) in (\"\")"=w605) -> ("States Out"=w604:string)  [unwired: 14 in]
          }
          frame "UI: Cursor Set" {
            # "Argument"
            # "Set and Unset Cursor Busy.\n(Usage: \"UI: Cursor Set >> Busy|Idle\")"
            n280 = case shown="\"Idle\", Default" w606 {
              tunnel: w608 -> [w613 w615]
              tunnel: [w612 w614] -> w607
              frame "Idle", Default {
                n281 = call <vilib>:"Unset Busy.vi"("error in (no error)"=w613) -> ("error out"=w612:errorcluster)  [unwired: 10 in]
              }
              frame "Busy" {
                n282 = call <vilib>:"Set Busy.vi"("error in (no error)"=w615) -> ("error out"=w614:errorcluster)  [unwired: 9 in, 1 out]
              }
            }
            n283 = call <vilib>:"Add State(s) to Queue__jki_lib_state_machine.vi"("State(s) in (\"\")"=w611) -> ("States Out"=w610:string)  [unwired: 14 in]
          }
          frame "UI: Front Panel State" {
            # "Argument"
            # "Set Front Panel Open or Closed\n(Usage: \"UI: Front Panel State >> Open|Close\")"
            n284 = Unbundle By Name(w616) -> ("Core.Current VI Reference"=w618:refnum<vi>)
            n285 = case shown="\"Open\", Default" w617 {
              tunnel: w620 -> [w626 w637]
              tunnel: [w627 w638] -> w619
              tunnel: w618 -> [_ _]
              frame "Open", Default {
                n286 = property class="VI"(error in=w626) -> (reference out=w624:refnum<vi>, error out=w625:errorcluster, "Front Panel.Open"=w623:bool)  [unwired: 1 in]
                n287 = case shown="False" w623 {
                  tunnel: [w630 w633] -> w627
                  tunnel: w625 -> [w629 w633]
                  tunnel: w624 -> [w628 _]
                  frame False {
                    n288 = invoke class="VI" method="FP.Open"(reference=w628, error in=w629, "Activate"=TRUE, "State"=T16."Standard") -> (error out=w630:errorcluster)  [unwired: 1 in, 4 out]
                  }
                  frame True {
                  }
                }
              }
              frame "Close" {
                n289 = property class="VI"(error in=w637) -> (reference out=w635:refnum<vi>, error out=w636:errorcluster, "Front Panel.Open"=w634:bool)  [unwired: 1 in]
                n290 = case shown="True" w634 {
                  tunnel: [w639 w642] -> w638
                  tunnel: w636 -> [w639 w641]
                  tunnel: w635 -> [_ w640]
                  frame False {
                  }
                  frame True {
                    n291 = invoke class="VI" method="FP.Close"(reference=w640, error in=w641) -> (error out=w642:errorcluster)  [unwired: 1 in, 2 out]
                  }
                }
              }
            }
            n292 = call <vilib>:"Add State(s) to Queue__jki_lib_state_machine.vi"("State(s) in (\"\")"=w622) -> ("States Out"=w621:string)  [unwired: 14 in]
          }
          frame "---------- Macro ----------" {
            # "Do not put any code in this frame.\n(It is a separator no-op. You can make a copy of this frame to create a new Macro frame)"
            n293 = call <vilib>:"Add State(s) to Queue__jki_lib_state_machine.vi"("State(s) in (\"\")"=w646) -> ("States Out"=w645:string)  [unwired: 14 in]
          }
          frame "Macro: Initialize" {
            # "Initialization Macro\n(This is called once, when the VI starts)"
            n294 = property on="img to avg" class="DigNum (strict)"() -> ("Value"=w648:i32)  [unwired: 2 in, 2 out]
            n295 = Number To Decimal String(number=w648) -> (decimal integer string=w650:string)  [unwired: 1 in]
            n296 = call <vilib>:"Build State String with Arguments__jki_lib_state_machine.vi"("Arguments (\"\")"=w650, "State"="ImgToAvg") -> ("State with Arguments"=w647:string)  [unwired: 4 in]
            n297 = call <vilib>:"Add State(s) to Queue__jki_lib_state_machine.vi"("State(s) in Front (\"\")"="Data: Initialize\nInitialize Core Data\nUI: Initialize\nUI: Front Panel State >> Open\nDevice Ini >> 3000", "State(s) in (\"\")"=w655, "State(s) at Back (\"\")"=w647) -> ("States Out"=w654:string)  [unwired: 12 in]
          }
          frame "Macro: Exit" {
            # "Exit Macro\n(This is called once, when the VI exits)"
            n298 = Unbundle By Name(w657) -> ("Core.Close Panel on Exit?"=w656:bool)
            n299 = Select(t="UI: Front Panel State >> Close", s=w656, f="") -> (s? t:f=w660:string)
            n300 = call <vilib>:"Add State(s) to Queue__jki_lib_state_machine.vi"("State(s) in (\"\")"=w660, "State(s) at Back (\"\")"="Data: Cleanup\nExit") -> ("States Out"=w658:string)  [unwired: 13 in]
            n301 = call <vilib>:"Add State(s) to Queue__jki_lib_state_machine.vi"("State(s) in Front (\"\")"=w658, "State(s) in (\"\")"=w665) -> ("States Out"=w664:string)  [unwired: 13 in]
          }
          frame "---------- Ini and Configure ----------" {
            # "Template Separator\n(You can make a copy of, or modify, this frame)"
            n302 = call <vilib>:"Add State(s) to Queue__jki_lib_state_machine.vi"("State(s) in (\"\")"=w669) -> ("States Out"=w668:string)  [unwired: 14 in]
          }
          frame "Device Ini" {
            # "Your code here.\n(You can make a copy of, or modify, this frame)"
            n303 = Empty String/Path?(string/path=w673) -> (empty?=w690:bool)
            n304 = flat-sequence {
              tunnel: w696 -> [w735]
              tunnel: [w735] -> w695
              tunnel: w689 -> [w734]
              tunnel: w695 -> [w741]
              tunnel: [w739] -> w676
              tunnel: [w738] -> _
              frame #0 {
                n305 = Wait (ms)(milliseconds to wait=w734) -> ()  [unwired: 1 out]
              }
              frame #1 {
                n306 = local read "Array 3"() -> (w736:sgl[])
                n307 = disable-structure shown="Disabled" {
                  disable-tunnel: w741 -> [w744 _]
                  disable-tunnel: [w742 _] -> w738
                  frame Disabled {
                    n308 = for {
                      tunnel: w744 -> [w745] mode=indexing
                      shift-right: [w747] -> w742
                      shift-left: string[] [] -> [w748]
                      n309 = call "send command.vi"("Device Name"=w745) -> ("status"=w749:bool)  [unwired: 4 in]
                      n310 = Wait (ms)(milliseconds to wait=u32 1) -> ()  [unwired: 1 out]
                      n311 = case shown="True" w749 {
                        tunnel: w748 -> [w750 w753]
                        tunnel: [w750 w752] -> w747
                        tunnel: w745 -> [_ w751]
                        frame False {
                        }
                        frame True {
                          n312 = Build Array (concatenate)(w753, w751) -> (w752:string[])
                        }
                      }
                    }
                  }
                  frame Enabled {
                  }
                }
                n313 = for {
                  tunnel: w741 -> [w756] mode=indexing
                  shift-right: [w761] -> w739
                  shift-left: string[] [] -> [w762]
                  tunnel: [w755] -> w737 mode=indexing
                  shift-right: [w759] -> _
                  shift-left: w736 -> [w759]
                  i -> [w760]
                  n314 = call "IMAQ Histograph"("Image"=w756) -> ("error out"=w754:errorcluster, "Mean Value"=w755:sgl)  [unwired: 7 in, 2 out]
                  n315 = Index Array(array=w759, index=w760) -> (element=w758:sgl)
                  n316 = call <vilib>:"Clear Errors.vi"("error in (no error)"=w754) -> ()  [unwired: 5 in, 2 out]
                  n317 = Equal?(x=w755, y=w758) -> (x = y?=w757:bool)
                  n318 = case shown="False" w757 {
                    tunnel: w762 -> [w765 w766]
                    tunnel: [w764 w766] -> w761
                    tunnel: w756 -> [w763 _]
                    frame False {
                      n319 = Build Array (concatenate)(w765, w763) -> (w764:string[])
                    }
                    frame True {
                    }
                  }
                }
                "Array 3" <- w737
              }
            }
            n320 = case shown="False" w690 {
              tunnel: w673 -> [w732 _]
              tunnel: [w731 0] -> w689
              frame False {
                n321 = Decimal String To Number(string=w732) -> (number=w731:i32)  [unwired: 2 in, 1 out]
              }
              frame True {
              }
            }
            n322 = Equal?(x=w673, y="T") -> (x = y?=w671:bool)
            n323 = Unbundle By Name(w688) -> ("active cams"=w681:string[])
            n324 = call <vilib>:"Add State(s) to Queue__jki_lib_state_machine.vi"("State(s) in (\"\")"=w697) -> ("States Out"=w683:string)  [unwired: 14 in]
            n325 = Equal?(x=w681, y=w676) -> (x = y?=w687:bool[])
            n326 = Empty Array?(array=w681) -> (empty?=w686:bool)
            n327 = Not(x=w686) -> (.not. x?=w685:bool)
            n328 = Build Array (concatenate)(w687, w685) -> (w684:bool[])
            n329 = Array Size(array=w676) -> (size(s)=w680:i32)
            n330 = Array Size(array=w681) -> (size(s)=w679:i32)
            n331 = And Array Elements(Boolean array=w684) -> (logical AND=w677:bool)
            n332 = Equal?(x=w680, y=w679) -> (x = y?=w678:bool)
            n333 = And(x=w678, y=w677) -> (x .and. y?=w675:bool)
            n334 = Not(x=w675) -> (.not. x?=w672:bool)
            n335 = Or(x=w672, y=w671) -> (x .or. y?=w670:bool)
            n336 = case shown="True" w670 {
              tunnel: [w700 w716] -> w694
              tunnel: w693 -> [_ _]
              tunnel: w692 -> [w699 w714]
              tunnel: [w699 w714] -> w691
              tunnel: w688 -> [w700 w710]
              tunnel: w676 -> [_ w711]
              tunnel: w683 -> [w698 _]
              tunnel: [w698 w704] -> w682
              frame False {
              }
              frame True {
                n337 = property on="active CCDs" class="LstBox (strict)"("Item Names"=w711) -> ()  [unwired: 2 in, 2 out]
                n338 = Array Size(array=w711) -> (size(s)=w723:i32)
                n339 = Initialize Array(0.0 ("element"), w723, 0 ("dimension size")) -> (w718:dbl[][])
                n340 = Unbundle By Name(w710) -> ("img to avg"=w709:i32)
                n341 = Bundle By Name(cluster=w710, "active cams"=w711) -> (w717:T35)
                n342 = Initialize Array(0.0 ("element"), 12 ("dimension size"), w709) -> (w708:dbl[][])
                n343 = local write "Numeric"(0.0 ("Numeric")) -> ()
                n344 = Bundle By Name(cluster=w717, "Offset X stats"=w718, "Offset Y stats"=w718, "Centroid X"=w708, "Centroid Y"=w708, "Mean Centroid X"=w718, "Mean Centroid Y"=w718, "Offset X"=w718, "Offset Y"=w718, "Size"=w708, "Mean Size"=w718, "Motor X"=w718, "Motor Y"=w718) -> (w716:T35)
                n345 = for {
                  N: 1 -> [_]
                  shift-right: [w725] -> w721
                  shift-left: timestamp[][] [] ("Time") -> [w727]
                  n346 = for {
                    N: 12 -> [_]
                    tunnel: w727 -> [w730] mode=indexing
                    tunnel: [w728] -> w725 mode=indexing
                    n347 = Get Date/Time In Seconds() -> (seconds since 1Jan1904=w729:timestamp)
                    n348 = Build Array (concatenate)(w730, w729) -> (w728:timestamp[])
                  }
                }
                n349 = property on="config path" class="Str"() -> ("Value"=w706:string)  [unwired: 2 in, 2 out]
                n350 = call <vilib>:"Add State(s) to Queue__jki_lib_state_machine.vi"("State(s) in Front (\"\")"="Move Config\nMotor Config\nDetection Config\nactive\nCenter" ("State(s) in Front (\"\")"), "State(s) in (\"\")"="" ("State(s) in (\"\")")) -> ("States Out"=w705:string)  [unwired: 13 in]
                n351 = call <vilib>:"Build State String with Arguments__jki_lib_state_machine.vi"("Arguments (\"\")"=w706, "State"="Load Config" ("State(s) in Front (\"\")")) -> ("State with Arguments"=w703:string)  [unwired: 4 in]
                n352 = call <vilib>:"Add State(s) to Queue__jki_lib_state_machine.vi"("State(s) in (\"\")"=w705, "State(s) at Back (\"\")"=w703) -> ("States Out"=w704:string)  [unwired: 13 in]
                n353 = property on="Time" class="Arr (strict)"("Value"=w721) -> ()  [unwired: 2 in, 2 out]
                "name array" <- w711
              }
            }
          }
          frame "Load Config" {
            # "Your code here.\n(You can make a copy of, or modify, this frame)"
            n354 = Unbundle By Name(w808) -> ("detection para"=w814:T3[], "move properties"=w811:T2[], "thresholds"=w804:cluster{"Lower value":sgl, "Upper value":sgl}[])
            n355 = Empty String/Path?(string/path=w771) -> (empty?=w770:bool)
            n356 = case shown="False" w770 {
              tunnel: [w824 T5 {"CCDs"=[], "move properties"=[], "detection para"=[], "thresholds"=[], "Value"={"Motor CCD 1"=0, "Motor CCD 2"=0, "Motor CCD 3"=0, "Motor CCD 4"=0, "Motor CCD 5"=0, "Motor CCD 6"=0, "Motor CCD 7"=0, "Motor CCD 8"=0, "Motor CCD 9"=0, "Motor CCD 10"=0, "Motor CCD 11"=0, "Motor CCD 12"=0}} ("output cluster 2")] -> w816
              tunnel: [w822 w831] -> w775
              tunnel: w772 -> [w821 w831]
              tunnel: w771 -> [w820 _]
              frame False {
                n357 = String To Path(string=w820) -> (path=w819:path)
                n358 = Open/Create/Replace File(file path (use dialog)=w819, error in=w821, operation (0:open)=T17."open or create") -> (refnum out=w826:refnum<file>, error out=w827:errorcluster)  [unwired: 3 in, 1 out]
                n359 = Read from Binary File(5:"output cluster 2", 8:w827, 11:w826) -> (0:w828:errorcluster, 2:w824:T5, 3:w829:refnum<file>)  [unwired: 3 in, 1 out]
                n360 = Close File(refnum=w829, error in=w828) -> (error out=w822:errorcluster)  [unwired: 1 out]
              }
              frame True {
              }
            }
            n361 = property on="Load Config" class="Bool (strict)"("Value"=FALSE ("Load Config")) -> ()  [unwired: 2 in, 2 out]
            n362 = Unbundle By Name(w816) -> ("Value"=w802:T7, "CCDs"=w815:string[], "detection para"=w813:T3[], "move properties"=w812:T2[], "thresholds"=w805:cluster{"Lower value":sgl, "Upper value":sgl}[])
            n363 = Cluster To Array(cluster=w802) -> (array=w803:u16[])
            n364 = call <vilib>:"Add State(s) to Queue__jki_lib_state_machine.vi"("State(s) in (\"\")"=w818, "State(s) at Back (\"\")"="Motor Config" ("State(s) at Back (\"\")")) -> ("States Out"=w817:string)  [unwired: 13 in]
            n365 = for {
              tunnel: w815 -> [w847]
              tunnel: w813 -> [w849]
              tunnel: w812 -> [w848]
              shift-right: [w841] -> w810
              shift-left: w814 -> [w846]
              shift-right: [w839] -> w809
              shift-left: w811 -> [w845]
              tunnel: w806 -> [w844] mode=indexing
              tunnel: w805 -> [w840]
              shift-right: [w836] -> w768
              shift-left: w804 -> [w838]
              tunnel: w803 -> [w835]
              tunnel: [w832] -> w801 mode=indexing
              i -> [w833]
              n366 = call-poly <userlib>:"Filter 1D Array__ogtk.vi"("items to filter"=w844, "array"=w847) -> ("filtered item indices"=w850:i32[])  [unwired: 4 in, 1 out]
              n367 = Index Array(array=w850) -> (element=w834:i32)  [unwired: 1 in]
              n368 = Index Array(array=w835, index=w834) -> (element=w832:u16)
              n369 = Index Array(array=w849, index=w834) -> (element=w843:T3)
              n370 = Index Array(array=w848, index=w834) -> (element=w842:T2)
              n371 = Index Array(array=w840, index=w834) -> (element=w837:cluster{"Lower value":sgl, "Upper value":sgl})
              n372 = Replace Array Subset(array=w846, new element=w843, index=w833) -> (w841:T3[])
              n373 = Replace Array Subset(array=w845, new element=w842, index=w833) -> (w839:T2[])
              n374 = Replace Array Subset(array=w838, new element=w837, index=w833) -> (w836:cluster{"Lower value":sgl, "Upper value":sgl}[])
            }
            n375 = Array Size(array=w768) -> (size(s)=→"size(s) 6":i32)
            n376 = Index Array(array=w801, index #1=0 ("index (row)"), index #2=1 ("index (row)"), index #3=2 ("index (row)"), index #4=3 ("index (row)"), index #5=4 ("index (row)"), index #6=5 ("index (row)"), index #7=6 ("index (row)"), index #8=7 ("index (row)"), index #9=8 ("index (row)"), index #10=9 ("index (row)"), index #11=10 ("index (row)"), index #12=11 ("index (row)")) -> (element #1=w788:u16, element #2=w787:u16, element #3=w786:u16, element #4=w785:u16, element #5=w784:u16, element #6=w783:u16, element #7=w782:u16, element #8=w781:u16, element #9=w780:u16, element #10=w779:u16, element #11=w778:u16, element #12=w777:u16)
            n377 = Bundle By Name(cluster=w802, "Motor CCD 1"=w788, "Motor CCD 2"=w787, "Motor CCD 3"=w786, "Motor CCD 4"=w785, "Motor CCD 5"=w784, "Motor CCD 6"=w783, "Motor CCD 7"=w782, "Motor CCD 8"=w781, "Motor CCD 9"=w780, "Motor CCD 10"=w779, "Motor CCD 11"=w778, "Motor CCD 12"=w777) -> (w776:T7)
            n378 = Bundle By Name(cluster=w808, "detection para"=w810, "move properties"=w809, "thresholds"=w768) -> (w807:T35)
            n379 = property on="associated motors" class="Clust (strict)"(error in=w775, "Val(Sgnl)"=w776) -> (error out=w774:errorcluster)  [unwired: 1 in, 1 out]
          }
          frame "Save Config" {
            # "Your code here.\n(You can make a copy of, or modify, this frame)"
            n380 = Unbundle By Name(w868) -> ("move properties"=w854:T2[], "detection para"=w863:T3[], "thresholds"=w851:cluster{"Lower value":sgl, "Upper value":sgl}[])
            n381 = property on="associated motors" class="Clust (strict)"() -> ("Value"=w862:T7)  [unwired: 2 in, 2 out]
            n382 = property on="Save Config" class="Bool (strict)"("Value"=FALSE ("Save Config")) -> ()  [unwired: 2 in, 2 out]
            n383 = local read "CCDs"() -> (w852:string[])
            n384 = call "File Dialog"("pattern (all files)"="*.cfg", "pattern label"="config") -> ("selected path"=w856:path)  [unwired: 10 in, 3 out]
            n385 = Bundle("CCDs"=w852, "move properties"=w854, "detection para"=w863, "thresholds"=w851, "Value"=w862) -> (w855:T5)  [unwired: 1 in]
            n386 = Open/Create/Replace File(file path (use dialog)=w856, error in=w860, operation (0:open)=T17."replace or create with confirmation") -> (refnum out=w864:refnum<file>, error out=w865:errorcluster)  [unwired: 3 in, 1 out]
            n387 = Write to Binary File(file (use dialog)=w864, data=w855, error in=w865) -> (refnum out=w867:refnum<file>, error out=w866:errorcluster)  [unwired: 3 in, 1 out]
            n388 = Close File(refnum=w867, error in=w866) -> (error out=w859:errorcluster)  [unwired: 1 out]
            n389 = call <vilib>:"Add State(s) to Queue__jki_lib_state_machine.vi"("State(s) in (\"\")"=w870) -> ("States Out"=w869:string)  [unwired: 14 in]
          }
          frame "active" {
            # "Your code here.\n(You can make a copy of, or modify, this frame)"
            n390 = Empty String/Path?(string/path=w885) -> (empty?=w884:bool)
            n391 = Unbundle By Name(w881) -> ("move properties"=w897:T2[], "detection para"=w893:T3[])  [unwired: 1 out]
            n392 = Unbundle By Name(w881) -> ("active axis refs 2"=w880:T11)
            n393 = call-poly <userlib>:"Filter 1D Array__ogtk.vi"("items to filter"=w885, "array"=w895) -> ("filtered item indices"=w898:i32[])  [unwired: 4 in, 1 out]
            n394 = Index Array(array=w898) -> (element=w882:i32)  [unwired: 1 in]
            n395 = Select(t=0, s=w884, f=w882) -> (s? t:f=w878:i32)
            n396 = Index Array(array=w880, index=w878) -> (element=w879:cluster{"Ref X":refnum<vi>, "Ref Y":refnum<vi>})
            n397 = Unbundle By Name(w879) -> ("Ref X"=w877:refnum<vi>, "Ref Y"=w876:refnum<vi>)
            n398 = Index Array(array=w897, index=w878) -> (element=w896:T2)
            n399 = Index Array(array=w893, index=w878) -> (element=w892:T3)
            n400 = property on="move config" class="Clust (strict)"(error in=w888, "Value"=w896) -> (error out=w886:errorcluster)  [unwired: 1 in, 1 out]
            n401 = property on="beam detection para" class="Clust (strict)"(error in=w886, "Value"=w892) -> (error out=w887:errorcluster)  [unwired: 1 in, 1 out]
            n402 = call <vilib>:"Add State(s) to Queue__jki_lib_state_machine.vi"("State(s) in (\"\")"=w900) -> ("States Out"=w899:string)  [unwired: 14 in]
            n403 = Bundle By Name(cluster="active Axis ref 3", "Ref X"=w877, "Ref Y"=w876) -> (w890:cluster{"Ref X":refnum<vi>, "Ref Y":refnum<vi>})
            n404 = property class="DigNum (strict)"(reference=w877, error in=w887) -> (error out=w873:errorcluster, "Value"=w875:dbl)  [unwired: 1 out]
            n405 = Bundle By Name(cluster=w881, "active ccd"=w878, "active man refs"=w890) -> (w894:T35)
            n406 = property on="Position 1" class="DigNum (strict)"(error in=w873, "Value"=w875) -> (error out=w872:errorcluster)  [unwired: 1 in, 1 out]
            n407 = property class="DigNum (strict)"(reference=w876, error in=w872) -> (error out=w871:errorcluster, "Value"=w874:dbl)  [unwired: 1 out]
            n408 = property on="Position 2" class="DigNum (strict)"(error in=w871, "Value"=w874) -> (error out=w889:errorcluster)  [unwired: 1 in, 1 out]
          }
          frame "Detection Config" {
            # "Your code here.\n(You can make a copy of, or modify, this frame)"
            n409 = Unbundle By Name(w905) -> ("detection para"=w901:T3[], "active ccd"=w906:i32)
            n410 = Replace Array Subset(array=w901, new element="beam detection para", index=w906) -> (w902:T3[])
            n411 = Bundle By Name(cluster=w905, "detection para"=w902) -> (w904:T35)
            n412 = call <vilib>:"Add State(s) to Queue__jki_lib_state_machine.vi"("State(s) in (\"\")"=w909) -> ("States Out"=w908:string)  [unwired: 14 in]
          }
          frame "Motor Config" {
            # "Your code here.\n(You can make a copy of, or modify, this frame)"
            n413 = Unbundle By Name("associated motors") -> ("Motor CCD 1"=w926:u16, "Motor CCD 2"=w927:u16, "Motor CCD 3"=w928:u16, "Motor CCD 4"=w921:u16, "Motor CCD 5"=w920:u16, "Motor CCD 6"=w919:u16, "Motor CCD 7"=w918:u16, "Motor CCD 8"=w917:u16, "Motor CCD 9"=w916:u16, "Motor CCD 10"=w915:u16, "Motor CCD 11"=w914:u16, "Motor CCD 12"=w913:u16)
            n414 = Build Array(w926, w927, w928, w921, w920, w919, w918, w917, w916, w915, w914, w913) -> (w912:u16[])
            n415 = local read "motor refs"() -> (w924:refnum<vi>[])
            n416 = Increment(x=w912) -> (x+1=w911:u16[])
            n417 = for {
              tunnel: w911 -> [w943] mode=indexing
              tunnel: w924 -> [w938]
              tunnel: [w932] -> w910 mode=indexing
              n418 = Multiply(x=w943, y=u16 2) -> (x*y=w939:u16)
              n419 = Subtract(x=w939, y=u16 2) -> (x-y=w937:u16)
              n420 = Subtract(x=w939, y=u16 1) -> (x-y=w936:u16)
              n421 = Index Array(array=w938, index=w937) -> (element=w935:refnum<vi>)
              n422 = Index Array(array=w938, index=w936) -> (element=w934:refnum<vi>)
              n423 = Bundle By Name(cluster="active Axis ref", "Ref X"=w935, "Ref Y"=w934) -> (w932:cluster{"Ref X":refnum<vi>, "Ref Y":refnum<vi>})
            }
            n424 = call <vilib>:"Add State(s) to Queue__jki_lib_state_machine.vi"("State(s) in (\"\")"=w931) -> ("States Out"=w930:string)  [unwired: 14 in]
            n425 = Bundle By Name(cluster=w923, "active axis refs 2"=w910) -> (w922:T35)
          }
          frame "Move Config" {
            # "Your code here.\n(You can make a copy of, or modify, this frame)"
            n426 = Unbundle By Name(w945) -> ("move properties"=w949:T2[], "active ccd"=w948:i32)
            n427 = Replace Array Subset(array=w949, new element="move config", index=w948) -> (w946:T2[])
            n428 = Bundle By Name(cluster=w945, "move properties"=w946) -> (w944:T35)
            n429 = call <vilib>:"Add State(s) to Queue__jki_lib_state_machine.vi"("State(s) in (\"\")"=w952) -> ("States Out"=w951:string)  [unwired: 14 in]
          }
          frame "----------Centroid & Move----------" {
            # "Template Separator\n(You can make a copy of, or modify, this frame)"
            n430 = call <vilib>:"Add State(s) to Queue__jki_lib_state_machine.vi"("State(s) in (\"\")"=w956) -> ("States Out"=w955:string)  [unwired: 14 in]
          }
          frame "detected" {
            n431 = Unbundle By Name(w964) -> ("Offset X"=w996:dbl[][], "Offset Y"=w995:dbl[][], "Size"=w994:dbl[][], "Mean Size"=w993:dbl[][], "Time"=w990:timestamp[][], "Motor X"=w973:dbl[][], "active axis refs 2"=w972:T11, "Motor Y"=w971:dbl[][])
            n432 = Spreadsheet String To Array(format string="%s", spreadsheet string=w976, array type (2D Dbl)=string[] []) -> (array=w967:string[])  [unwired: 1 in]
            n433 = for {
              tunnel: w968 -> [w1009] mode=indexing
              tunnel: w967 -> [w1008]
              tunnel: [w1007] -> w966 mode=indexing
              n434 = for {
                tunnel: w1009 -> [w1012]
                tunnel: [w1011] -> w1006 mode=indexing
                tunnel: w1008 -> [w1010] mode=indexing
                n435 = Equal?(x=w1012, y=w1010) -> (x = y?=w1011:bool)
              }
              n436 = Or Array Elements(Boolean array=w1006) -> (logical OR=w1007:bool)
            }
            n437 = Unbundle By Name(w964) -> ("Mean Centroid X"=w1000:dbl[][], "Mean Centroid Y"=w999:dbl[][], "Centroid X"=w1002:dbl[][], "Centroid Y"=w1001:dbl[][])
            n438 = call <vilib>:"Add State(s) to Queue__jki_lib_state_machine.vi"("State(s) in (\"\")"=w975) -> ("States Out"=w974:string)  [unwired: 14 in]
            n439 = for {
              tunnel: w1002 -> [w1062]
              tunnel: w1001 -> [w1061]
              tunnel: w1000 -> [w1060]
              tunnel: w999 -> [w1059]
              tunnel: [w1058] -> w987 mode=indexing
              tunnel: [w1057] -> w998 mode=indexing
              tunnel: w997 -> [w1056] mode=indexing
              tunnel: w996 -> [w1055]
              tunnel: w995 -> [w1054]
              tunnel: [w1053] -> w965 mode=indexing
              tunnel: [w1052] -> w988 mode=indexing
              tunnel: w994 -> [w1051]
              tunnel: w993 -> [w1050]
              tunnel: [w1049] -> w992 mode=indexing
              tunnel: w990 -> [w1048]
              tunnel: [w1047] -> w989 mode=indexing
              tunnel: w973 -> [w1039]
              tunnel: w972 -> [w1038]
              tunnel: w971 -> [w1037]
              tunnel: [w1017] -> w970 mode=indexing
              tunnel: [w1016] -> w969 mode=indexing
              tunnel: w966 -> [w1015]
              i -> [w1014]
              n440 = Unbundle By Name(w1056) -> ("Target.X::12"=w1021:refnum<vi>, "Target.Y::12"=w1020:refnum<vi>)
              n441 = Index Array(array=w1039, index (row)=w1014) -> (element=w1042:dbl[])  [unwired: 1 in]
              n442 = Index Array(array=w1038, index=w1014) -> (element=w1041:cluster{"Ref X":refnum<vi>, "Ref Y":refnum<vi>})
              n443 = Index Array(array=w1037, index (row)=w1014) -> (element=w1046:dbl[])  [unwired: 1 in]
              n444 = Index Array(array=w1015, index=w1014) -> (element=w1013:bool)
              n445 = Index Array(array=w1060, index (row)=w1014) -> (element=w1033:dbl[])  [unwired: 1 in]
              n446 = Index Array(array=w1059, index (row)=w1014) -> (element=w1034:dbl[])  [unwired: 1 in]
              n447 = Index Array(array=w1062, index (row)=w1014) -> (element=w1036:dbl[])  [unwired: 1 in]
              n448 = Index Array(array=w1061, index (row)=w1014) -> (element=w1035:dbl[])  [unwired: 1 in]
              n449 = Index Array(array=w1055, index (row)=w1014) -> (element=w1029:dbl[])  [unwired: 1 in]
              n450 = Index Array(array=w1054, index (row)=w1014) -> (element=w1028:dbl[])  [unwired: 1 in]
              n451 = Index Array(array=w1051, index (row)=w1014) -> (element=w1026:dbl[])  [unwired: 1 in]
              n452 = Index Array(array=w1050, index (row)=w1014) -> (element=w1025:dbl[])  [unwired: 1 in]
              n453 = Index Array(array=w1048, index (row)=w1014) -> (element=w1022:timestamp[])  [unwired: 1 in]
              n454 = Unbundle By Name(w1041) -> ("Ref X"=w1040:refnum<vi>, "Ref Y"=w1044:refnum<vi>)
              n455 = property class="DigNum (strict)"(reference=w1021) -> ("Value"=w1019:dbl)  [unwired: 1 in, 2 out]
              n456 = property class="DigNum (strict)"(reference=w1020) -> ("Value"=w1018:dbl)  [unwired: 1 in, 2 out]
              n457 = call <vilib>:"Std Deviation and Variance.vi"("X"=w1036) -> ("mean"=w1032:dbl)  [unwired: 1 in, 2 out]
              n458 = call <vilib>:"Std Deviation and Variance.vi"("X"=w1035) -> ("mean"=w1031:dbl)  [unwired: 1 in, 2 out]
              n459 = call <vilib>:"Std Deviation and Variance.vi"("X"=w1026) -> ("mean"=w1024:dbl)  [unwired: 1 in, 2 out]
              n460 = Get Date/Time In Seconds() -> (seconds since 1Jan1904=w1023:timestamp)
              n461 = property class="DigNum (strict)"(reference=w1040) -> ("Value"=w1043:dbl)  [unwired: 1 in, 2 out]
              n462 = property class="DigNum (strict)"(reference=w1044) -> ("Value"=w1045:dbl)  [unwired: 1 in, 2 out]
              n463 = Subtract(x=w1019, y=w1032) -> (x-y=w1030:dbl)
              n464 = Subtract(x=w1018, y=w1031) -> (x-y=w1027:dbl)
              n465 = case shown="True" w1013 {
                tunnel: [w1075 w1094] -> w1058
                tunnel: [w1063 w1093] -> w1057
                tunnel: [w1064 w1092] -> w1053
                tunnel: [w1065 w1091] -> w1052
                tunnel: [w1066 w1090] -> w1049
                tunnel: [w1067 w1089] -> w1047
                tunnel: w1034 -> [w1073 w1088]
                tunnel: w1033 -> [w1074 w1087]
                tunnel: w1032 -> [_ w1086]
                tunnel: w1031 -> [_ w1085]
                tunnel: w1030 -> [_ w1084]
                tunnel: w1029 -> [w1072 w1083]
                tunnel: w1028 -> [w1071 w1082]
                tunnel: w1027 -> [_ w1081]
                tunnel: w1025 -> [w1070 w1080]
                tunnel: w1024 -> [_ w1079]
                tunnel: w1023 -> [w1068 w1078]
                tunnel: w1022 -> [w1069 w1077]
                frame False {
                  w1076 = 0.0
                  n466 = Build Array (concatenate)(w1074, w1076) -> (w1075:dbl[])
                  n467 = Build Array (concatenate)(w1073, w1076) -> (w1063:dbl[])
                  n468 = Build Array (concatenate)(w1072, w1076) -> (w1064:dbl[])
                  n469 = Build Array (concatenate)(w1071, w1076) -> (w1065:dbl[])
                  n470 = Build Array (concatenate)(w1070, w1076) -> (w1066:dbl[])
                  n471 = Build Array (concatenate)(w1069, w1068) -> (w1067:timestamp[])
                }
                frame True {
                  n472 = Build Array (concatenate)(w1087, w1086) -> (w1094:dbl[])
                  n473 = Build Array (concatenate)(w1088, w1085) -> (w1093:dbl[])
                  n474 = Build Array (concatenate)(w1083, w1084) -> (w1092:dbl[])
                  n475 = Build Array (concatenate)(w1082, w1081) -> (w1091:dbl[])
                  n476 = Build Array (concatenate)(w1080, w1079) -> (w1090:dbl[])
                  n477 = Build Array (concatenate)(w1077, w1078) -> (w1089:timestamp[])
                }
              }
              n478 = Build Array (concatenate)(w1042, w1043) -> (w1017:dbl[])
              n479 = Build Array (concatenate)(w1046, w1045) -> (w1016:dbl[])
            }
            n480 = local write "Numeric"(0.0 ("Numeric")) -> ()
            n481 = Array Size(array=w965) -> (size(s)=w986:i32[])
            n482 = Index Array(array=w986, index=1) -> (element=w984:i32)
            "History Index" <- w984
            n483 = call <vilib>:"Add State(s) to Queue__jki_lib_state_machine.vi"("State(s) in (\"\")"=w974, "State(s) at Back (\"\")"="Check Move\ntdms" ("State(s) at Back (\"\")")) -> ("States Out"=w978:string)  [unwired: 13 in]
            n484 = Unbundle By Name(w964) -> ("img to avg"=w961:i32)
            n485 = Initialize Array(0.0 ("element"), 12 ("dimension size"), w961) -> (w960:dbl[][])
            n486 = Greater?(x=w984, y="History Size") -> (0:w982:bool)
            n487 = Bundle By Name(cluster=w964, "Centroid X"=w960, "Centroid Y"=w960, "Mean Centroid X"=w987, "Mean Centroid Y"=w998, "Offset X"=w965, "Offset Y"=w988, "Mean Size"=w992, "Size"=w960, "Time"=w989, "Motor X"=w970, "Motor Y"=w969) -> (w957:T35)
            n488 = Select(t="history" ("State(s) at Back (\"\")"), s=w982, f="") -> (s? t:f=w979:string)
            n489 = call <vilib>:"Add State(s) to Queue__jki_lib_state_machine.vi"("State(s) in (\"\")"=w978, "State(s) at Back (\"\")"=w979) -> ("States Out"=w959:string)  [unwired: 13 in]
            n490 = call <vilib>:"Add State(s) to Queue__jki_lib_state_machine.vi"("State(s) in (\"\")"=w959) -> ("States Out"=w958:string)  [unwired: 14 in]
          }
          frame "Check Move" {
            (unwired) "Device Ini" ("State(s) in Front (\"\")")
            n491 = Unbundle By Name(w1103) -> ("move properties"=w1113:T2[], "Mean Size"=w1112:dbl[][], "move properties"=w1111:T2[], "Offset X"=w1110:dbl[][], "Offset Y"=w1109:dbl[][], "active cams"=w1108:string[])
            n492 = Unbundle By Name(w1103) -> ("steps speed X"=w1102:dbl[], "steps speed Y"=w1101:dbl[])
            n493 = for {
              tunnel: w1111 -> [w1151]
              tunnel: w1110 -> [w1149]
              tunnel: w1109 -> [w1147]
              tunnel: w1112 -> [w1155]
              tunnel: [w1166] -> w1097 mode=indexing
              tunnel: [w1162] -> w1095 mode=indexing
              tunnel: w1108 -> [w1156] mode=indexing
              tunnel: [w1184] -> w1114 mode=indexing
              tunnel: [w1183] -> w1106 mode=indexing
              tunnel: w1113 -> [w1154]
              tunnel: [w1145] -> w1098 mode=indexing
              tunnel: [w1144] -> w1096 mode=indexing
              tunnel: "Speedmode" -> [w1159]
              tunnel: w1105 -> [w1157]
              shift-right: [w1137] -> w1100
              shift-left: w1102 -> [w1142]
              shift-right: [w1136] -> w1099
              shift-left: w1101 -> [w1141]
              n494 = call-poly <userlib>:"Filter 1D Array__ogtk.vi"("items to filter"=w1156, "array"=w1157) -> ("filtered item indices"=w1158:i32[])  [unwired: 4 in, 1 out]
              n495 = Index Array(array=w1158) -> (element=w1140:i32)  [unwired: 1 in]
              n496 = Index Array(array=w1154, index=w1140) -> (element=w1153:T2)
              n497 = Index Array(array=w1155, index (row)=w1140) -> (element=w1152:dbl[])  [unwired: 1 in]
              n498 = Index Array(array=w1151, index=w1140) -> (element=w1150:T2)
              n499 = Index Array(array=w1149, index (row)=w1140) -> (element=w1148:dbl[])  [unwired: 1 in]
              n500 = Index Array(array=w1147, index (row)=w1140) -> (element=w1146:dbl[])  [unwired: 1 in]
              n501 = Unbundle By Name(w1150) -> ("Tolerance [%]"=w1177:dbl)
              n502 = Reverse 1D Array(array=w1148) -> (reversed array=w1182:dbl[])
              n503 = Reverse 1D Array(array=w1146) -> (reversed array=w1181:dbl[])
              n504 = Reverse 1D Array(array=w1152) -> (reversed array=w1176:dbl[])
              n505 = Unbundle By Name(w1153) -> ("Stepsize"=w1135:dbl, "enable feedback"=w1165:bool)
              n506 = Index Array(array=w1182) -> (element=w1180:dbl)  [unwired: 1 in]
              n507 = Index Array(array=w1181) -> (element=w1179:dbl)  [unwired: 1 in]
              n508 = Index Array(array=w1176) -> (element=w1175:dbl)  [unwired: 1 in]
              n509 = Absolute Value(x=w1180) -> (abs(x)=w1143:dbl)
              n510 = Absolute Value(x=w1179) -> (abs(x)=w1161:dbl)
              n511 = Square Root(x=w1175) -> (sqrt(x)=w1174:dbl)
              n512 = Divide(x=w1177, y=100.0) -> (x/y=w1173:dbl)
              n513 = Multiply(x=w1174, y=w1173) -> (x*y=w1160:dbl)
              n514 = Not Equal To 0?(x=w1161) -> (x != 0?=w1163:bool)
              n515 = Not Equal To 0?(x=w1143) -> (x != 0?=w1168:bool)
              n516 = Greater Or Equal?(x=w1143, y=w1160) -> (x >= y?=w1167:bool)
              n517 = Greater Or Equal?(x=w1161, y=w1160) -> (x >= y?=w1164:bool)
              n518 = call "speedmode.vi"("offset X"=w1143, "offset Y"=w1161, "beamsize x tolerance"=w1160, "Speedmode @"=w1159, "step size"=w1135) -> ("steps speed Y"=w1138:dbl, "steps speed X"=w1139:dbl, "speedmode X"=w1145:bool, "speedmode Y"=w1144:bool)  [unwired: 3 in]
              n519 = Compound Arithmetic op=AND(w1165, w1168, w1167) -> (w1166:bool)
              n520 = Compound Arithmetic op=AND(w1165, w1164, w1163) -> (w1162:bool)
              n521 = Boolean To (0,1)(Boolean=w1162) -> (0, 1=w1169:i16)
              n522 = Multiply(x=w1169, y=w1161) -> (x*y=w1170:dbl)
              n523 = Boolean To (0,1)(Boolean=w1166) -> (0, 1=w1172:i16)
              n524 = Replace Array Subset(array=w1142, new element=w1139, index=w1140) -> (w1137:dbl[])
              n525 = Replace Array Subset(array=w1141, new element=w1138, index=w1140) -> (w1136:dbl[])
              n526 = Multiply(x=w1172, y=w1143) -> (x*y=w1171:dbl)
              n527 = Bundle(w1170, "GUIdevice 8"=w1156) -> (w1183:cluster{dbl, "GUIdevice 8":string})  [unwired: 1 in]
              n528 = Bundle(w1171, "GUIdevice 8"=w1156) -> (w1184:cluster{dbl, "GUIdevice 8":string})  [unwired: 1 in]
            }
            "required X" <- w1097
            "required Y" <- w1095
            "speedmode X" <- w1098
            "speedmode Y" <- w1096
            n529 = case shown="False" "Align" {
              tunnel: w1114 -> [w1190 w1195]
              tunnel: w1106 -> [w1189 w1192]
              tunnel: [w1188 w1194] -> w1117
              tunnel: [w1187 w1191] -> w1116
              frame False {
                n530 = Sort 1D Array(array=w1189) -> (sorted array=w1186:cluster{dbl, "GUIdevice 8":string}[])
                n531 = Sort 1D Array(array=w1190) -> (sorted array=w1185:cluster{dbl, "GUIdevice 8":string}[])
                n532 = Reverse 1D Array(array=w1186) -> (reversed array=w1187:cluster{dbl, "GUIdevice 8":string}[])
                n533 = Reverse 1D Array(array=w1185) -> (reversed array=w1188:cluster{dbl, "GUIdevice 8":string}[])
              }
              frame True {
                w1193 = cluster{dbl, "GUIdevice 8":string}[] [] ("Array")
                n534 = for {
                  shift-right: [w1205] -> w1194
                  shift-left: w1193 -> [w1207]
                  tunnel: w1195 -> [w1206] mode=indexing
                  n535 = Unbundle(w1206) -> (w1209:dbl)  [unwired: 1 out]
                  n536 = Not Equal To 0?(x=w1209) -> (x != 0?=w1208:bool)
                  n537 = case shown="True" w1208 {
                    tunnel: w1207 -> [w1210 w1213]
                    tunnel: w1206 -> [_ w1212]
                    tunnel: [w1210 w1211] -> w1205
                    frame False {
                    }
                    frame True {
                      n538 = Build Array (concatenate)(w1213, w1212) -> (w1211:cluster{dbl, "GUIdevice 8":string}[])
                    }
                  }
                }
                n539 = for {
                  shift-right: [w1196] -> w1191
                  shift-left: w1193 -> [w1198]
                  tunnel: w1192 -> [w1197] mode=indexing
                  n540 = Unbundle(w1197) -> (w1200:dbl)  [unwired: 1 out]
                  n541 = Not Equal To 0?(x=w1200) -> (x != 0?=w1199:bool)
                  n542 = case shown="True" w1199 {
                    tunnel: w1198 -> [w1201 w1204]
                    tunnel: w1197 -> [_ w1203]
                    tunnel: [w1201 w1202] -> w1196
                    frame False {
                    }
                    frame True {
                      n543 = Build Array (concatenate)(w1204, w1203) -> (w1202:cluster{dbl, "GUIdevice 8":string}[])
                    }
                  }
                }
              }
            }
            n544 = call <vilib>:"Add State(s) to Queue__jki_lib_state_machine.vi"("State(s) in (\"\")"=w1120) -> ("States Out"=w1119:string)  [unwired: 14 in]
            n545 = Bundle By Name(cluster=w1103, "speedmode X"=w1098, "speedmode Y"=w1096, "steps speed X"=w1100, "steps speed Y"=w1099) -> (w1104:T35)
            n546 = Index Array(array=w1116) -> (element=w1121:cluster{dbl, "GUIdevice 8":string})  [unwired: 1 in]
            n547 = Index Array(array=w1117) -> (element=w1122:cluster{dbl, "GUIdevice 8":string})  [unwired: 1 in]
            n548 = Empty Array?(array=w1116) -> (empty?=w1124:bool)
            n549 = Unbundle(w1122) -> (w1130:dbl)  [unwired: 1 out]
            n550 = Unbundle(w1121) -> (w1126:dbl)  [unwired: 1 out]
            n551 = Unbundle By Name(w1104) -> ("Feedback global"=w1131:bool)
            n552 = Empty Array?(array=w1117) -> (empty?=w1128:bool)
            n553 = property on="autodetect" class="Bool (strict)"("Value"=FALSE ("autodetect")) -> ()  [unwired: 2 in, 2 out]
            n554 = Equal To 0?(x=w1130) -> (x = 0?=w1129:bool)
            n555 = Equal To 0?(x=w1126) -> (x = 0?=w1125:bool)
            n556 = Or(x=w1129, y=w1128) -> (x .or. y?=w1127:bool)
            n557 = Or(x=w1125, y=w1124) -> (x .or. y?=w1123:bool)
            n558 = case shown="True" w1131 {
              tunnel: w1127 -> [_ w1232]
              tunnel: w1117 -> [_ w1231]
              tunnel: w1123 -> [_ w1229]
              tunnel: w1116 -> [_ w1228]
              tunnel: w1119 -> [w1214 w1227]
              tunnel: [w1214 w1226] -> w1132
              tunnel: w1098 -> [_ w1225]
              tunnel: w1097 -> [_ w1224]
              tunnel: w1096 -> [_ w1223]
              tunnel: w1095 -> [_ w1222]
              frame False {
              }
              frame True {
                n559 = case shown="False" w1232 {
                  tunnel: w1231 -> [w1256 _]
                  tunnel: w1227 -> [w1252 w1257]
                  tunnel: [w1250 w1257] -> w1230
                  frame False {
                    n560 = Index Array(array=w1256) -> (element=w1255:cluster{dbl, "GUIdevice 8":string})  [unwired: 1 in]
                    n561 = Unbundle By Name(w1255) -> ("GUIdevice 8"=w1254:string)
                    n562 = call <vilib>:"Build State String with Arguments__jki_lib_state_machine.vi"("Arguments (\"\")"=w1254, "State"="Move X") -> ("State with Arguments"=w1251:string)  [unwired: 4 in]
                    n563 = call <vilib>:"Add State(s) to Queue__jki_lib_state_machine.vi"("State(s) in (\"\")"=w1252, "State(s) at Back (\"\")"=w1251) -> ("States Out"=w1250:string)  [unwired: 13 in]
                  }
                  frame True {
                  }
                }
                n564 = case shown="False" w1229 {
                  tunnel: w1228 -> [w1248 _]
                  tunnel: w1230 -> [w1244 w1249]
                  tunnel: [w1242 w1249] -> w1226
                  frame False {
                    n565 = Index Array(array=w1248) -> (element=w1247:cluster{dbl, "GUIdevice 8":string})  [unwired: 1 in]
                    n566 = Unbundle By Name(w1247) -> ("GUIdevice 8"=w1246:string)
                    n567 = call <vilib>:"Build State String with Arguments__jki_lib_state_machine.vi"("Arguments (\"\")"=w1246, "State"="Move Y") -> ("State with Arguments"=w1243:string)  [unwired: 4 in]
                    n568 = call <vilib>:"Add State(s) to Queue__jki_lib_state_machine.vi"("State(s) in (\"\")"=w1244, "State(s) at Back (\"\")"=w1243) -> ("States Out"=w1242:string)  [unwired: 13 in]
                  }
                  frame True {
                  }
                }
                n569 = for {
                  tunnel: w1225 -> [w1241] mode=indexing
                  tunnel: w1224 -> [w1240] mode=indexing
                  tunnel: [w1239] -> w1221 mode=indexing
                  n570 = And(x=w1241, y=w1240) -> (x .and. y?=w1239:bool)
                }
                n571 = for {
                  tunnel: w1223 -> [w1238] mode=indexing
                  tunnel: w1222 -> [w1237] mode=indexing
                  tunnel: [w1236] -> w1220 mode=indexing
                  n572 = And(x=w1238, y=w1237) -> (x .and. y?=w1236:bool)
                }
                n573 = Or Array Elements(Boolean array=w1221) -> (logical OR=w1219:bool)
                n574 = Or Array Elements(Boolean array=w1220) -> (logical OR=w1218:bool)
                n575 = Or(x=w1219, y=w1218) -> (x .or. y?=w1217:bool)
                n576 = property on="alarms" class="Bool (strict)"() -> ("Value"=w1216:bool)  [unwired: 2 in, 2 out]
                n577 = And(x=w1216, y=w1217) -> (x .and. y?=w1215:bool)
                n578 = case shown="True" w1215 {
                  frame False {
                  }
                  frame True {
                    n579 = call <vilib>:"Beep.vi"("use system alert? (T)"=FALSE, "duration (msec)"=u32 750, "frequency (Hz)"=u32 750) -> ()  [unwired: 9 in]
                  }
                }
              }
            }
            n580 = call <vilib>:"Add State(s) to Queue__jki_lib_state_machine.vi"("State(s) in (\"\")"=w1119, "State(s) at Back (\"\")"=w1132) -> ("States Out"=w1134:string)  [unwired: 13 in]
          }
          frame "Move X" {
            # "Your code here.\n(You can make a copy of, or modify, this frame)"
            n581 = Unbundle By Name(w1264) -> ("Offset X"=w1281:dbl[][])
            n582 = call-poly <userlib>:"Filter 1D Array__ogtk.vi"("items to filter"=w1268, "array"=w1285) -> ("filtered item indices"=w1272:i32[])  [unwired: 4 in, 1 out]
            n583 = Unbundle By Name(w1264) -> ("active axis refs 2"=w1284:T11, "move properties"=w1266:T2[])
            n584 = for {
              tunnel: w1272 -> [w1290] mode=indexing
              tunnel: w1266 -> [w1294]
              shift-right: [w1289] -> w1270
              shift-left: i32[] [] ("filtered item indices") -> [w1292]
              n585 = Index Array(array=w1294, index=w1290) -> (element=w1293:T2)
              n586 = Unbundle By Name(w1293) -> ("enable feedback"=w1291:bool)
              n587 = case shown="True" w1291 {
                tunnel: w1292 -> [w1295 w1298]
                tunnel: w1290 -> [_ w1297]
                tunnel: [w1295 w1296] -> w1289
                frame False {
                }
                frame True {
                  n588 = Build Array (concatenate)(w1298, w1297) -> (w1296:i32[])
                }
              }
            }
            n589 = Index Array(array=w1270) -> (element=w1261:i32)  [unwired: 1 in]
            n590 = Index Array(array=w1281, index (row)=w1261) -> (element=w1280:dbl[])  [unwired: 1 in]
            n591 = Reverse 1D Array(array=w1280) -> (reversed array=w1279:dbl[])
            n592 = Index Array(array=w1284, index=w1261) -> (element=w1283:cluster{"Ref X":refnum<vi>, "Ref Y":refnum<vi>})
            n593 = Index Array(array=w1279) -> (element=w1278:dbl)  [unwired: 1 in]
            n594 = Index Array(array=w1266, index=w1261) -> (element=w1282:T2)
            n595 = Unbundle By Name(w1283) -> ("Ref X"=w1275:refnum<vi>, "Ref Y"=w1274:refnum<vi>)
            n596 = Unbundle By Name(w1282) -> ("Invert Direction X"=w1276:bool, "Invert Axis"=w1265:bool, "enable feedback"=w1273:bool)
            n597 = Greater Or Equal To 0?(x=w1278) -> (x >= 0?=w1277:bool)
            n598 = Unbundle By Name(w1264) -> ("steps speed Y"=w1263:dbl[], "steps speed X"=w1262:dbl[])
            n599 = Index Array(array=w1262, index=w1261) -> (element=w1259:dbl)
            n600 = Index Array(array=w1263, index=w1261) -> (element=w1260:dbl)
            n601 = Select(t=w1260, s=w1265, f=w1259) -> (s? t:f=w1258:dbl)
            n602 = case shown="True" w1273 {
              tunnel: w1265 -> [_ w1304]
              tunnel: w1277 -> [_ w1303]
              tunnel: w1258 -> [_ w1302]
              tunnel: w1276 -> [_ w1301]
              tunnel: w1275 -> [_ w1300]
              tunnel: w1274 -> [_ w1299]
              frame False {
              }
              frame True {
                n603 = case shown="True" w1303 {
                  tunnel: w1301 -> [w1312 w1334]
                  tunnel: w1302 -> [w1310 w1332]
                  tunnel: w1304 -> [w1309 w1331]
                  tunnel: w1304 -> [w1308 w1330]
                  tunnel: w1300 -> [w1306 w1328]
                  tunnel: w1299 -> [w1305 w1327]
                  frame True {
                    n604 = case shown="True" w1309 {
                      tunnel: [w1323 w1325] -> w1311
                      tunnel: w1306 -> [w1324 _]
                      tunnel: w1305 -> [_ w1326]
                      frame False {
                        n605 = property class="DigNum (strict)"(reference=w1324) -> ("Value"=w1323:dbl)  [unwired: 1 in, 2 out]
                      }
                      frame True {
                        n606 = property class="DigNum (strict)"(reference=w1326) -> ("Value"=w1325:dbl)  [unwired: 1 in, 2 out]
                      }
                    }
                    n607 = case shown="True" w1312 {
                      tunnel: w1311 -> [w1319 w1322]
                      tunnel: w1310 -> [w1318 w1321]
                      tunnel: [w1317 w1320] -> w1307
                      frame False {
                        n608 = Add(x=w1319, y=w1318) -> (x+y=w1317:dbl)
                      }
                      frame True {
                        n609 = Subtract(x=w1322, y=w1321) -> (x-y=w1320:dbl)
                      }
                    }
                    n610 = case shown="True" w1308 {
                      tunnel: w1307 -> [w1313 w1315]
                      tunnel: w1306 -> [w1314 _]
                      tunnel: w1305 -> [_ w1316]
                      frame False {
                        n611 = property class="DigNum (strict)"(reference=w1314, "Val(Sgnl)"=w1313) -> ()  [unwired: 1 in, 2 out]
                      }
                      frame True {
                        n612 = property class="DigNum (strict)"(reference=w1316, "Val(Sgnl)"=w1315) -> ()  [unwired: 1 in, 2 out]
                      }
                    }
                  }
                  frame False {
                    n613 = case shown="False" w1331 {
                      tunnel: [w1345 w1347] -> w1333
                      tunnel: w1328 -> [w1346 _]
                      tunnel: w1327 -> [_ w1348]
                      frame False {
                        n614 = property class="DigNum (strict)"(reference=w1346) -> ("Value"=w1345:dbl)  [unwired: 1 in, 2 out]
                      }
                      frame True {
                        n615 = property class="DigNum (strict)"(reference=w1348) -> ("Value"=w1347:dbl)  [unwired: 1 in, 2 out]
                      }
                    }
                    n616 = case shown="False" w1334 {
                      tunnel: w1333 -> [w1341 w1344]
                      tunnel: w1332 -> [w1340 w1343]
                      tunnel: [w1339 w1342] -> w1329
                      frame False {
                        n617 = Subtract(x=w1341, y=w1340) -> (x-y=w1339:dbl)
                      }
                      frame True {
                        n618 = Add(x=w1344, y=w1343) -> (x+y=w1342:dbl)
                      }
                    }
                    n619 = case shown="False" w1330 {
                      tunnel: w1329 -> [w1335 w1337]
                      tunnel: w1328 -> [w1336 _]
                      tunnel: w1327 -> [_ w1338]
                      frame False {
                        n620 = property class="DigNum (strict)"(reference=w1336, "Val(Sgnl)"=w1335) -> ()  [unwired: 1 in, 2 out]
                      }
                      frame True {
                        n621 = property class="DigNum (strict)"(reference=w1338, "Val(Sgnl)"=w1337) -> ()  [unwired: 1 in, 2 out]
                      }
                    }
                  }
                }
              }
            }
            n622 = call <vilib>:"Build State String with Arguments__jki_lib_state_machine.vi"("Arguments (\"\")"=w1268, "State"="Wait" ("State(s) in Front (\"\")")) -> ("State with Arguments"=w1267:string)  [unwired: 4 in]
            n623 = call <vilib>:"Add State(s) to Queue__jki_lib_state_machine.vi"("State(s) in Front (\"\")"=w1267, "State(s) in (\"\")"=w1288) -> ("States Out"=w1287:string)  [unwired: 13 in]
            "Moving X" <- w1268
          }
          frame "ManMove X" {
            # "Your code here.\n(You can make a copy of, or modify, this frame)"
            n624 = Equal?(x=w1354, y="Right") -> (x = y?=w1355:bool)
            n625 = Unbundle By Name(w1364) -> ("move properties"=w1359:T2[], "active ccd"=w1352:i32, "active man refs"=w1357:cluster{"Ref X":refnum<vi>, "Ref Y":refnum<vi>}, "active cams"=w1353:string[])
            n626 = Index Array(array=w1353, index=w1352) -> (element=w1350:string)
            n627 = Index Array(array=w1359, index=w1352) -> (element=w1365:T2)
            n628 = Unbundle By Name(w1357) -> ("Ref X"=w1361:refnum<vi>, "Ref Y"=w1360:refnum<vi>)
            n629 = Unbundle By Name(w1365) -> ("Invert Direction X"=w1362:bool, "Invert Axis"=w1363:bool)
            n630 = call <vilib>:"Build State String with Arguments__jki_lib_state_machine.vi"("Arguments (\"\")"=w1350, "State"="Wait" ("State(s) in Front (\"\")")) -> ("State with Arguments"=w1349:string)  [unwired: 4 in]
            n631 = call <vilib>:"Add State(s) to Queue__jki_lib_state_machine.vi"("State(s) in Front (\"\")"=w1349, "State(s) in (\"\")"=w1368) -> ("States Out"=w1367:string)  [unwired: 13 in]
            n632 = case shown="False" w1355 {
              tunnel: w1362 -> [w1376 w1398]
              tunnel: "StepSize" -> [w1374 w1396]
              tunnel: w1363 -> [w1373 w1395]
              tunnel: w1363 -> [w1372 w1394]
              tunnel: w1361 -> [w1370 w1392]
              tunnel: w1360 -> [w1369 w1391]
              frame True {
                n633 = case shown="False" w1373 {
                  tunnel: [w1387 w1389] -> w1375
                  tunnel: w1370 -> [w1388 _]
                  tunnel: w1369 -> [_ w1390]
                  frame False {
                    n634 = property class="DigNum (strict)"(reference=w1388) -> ("Value"=w1387:dbl)  [unwired: 1 in, 2 out]
                  }
                  frame True {
                    n635 = property class="DigNum (strict)"(reference=w1390) -> ("Value"=w1389:dbl)  [unwired: 1 in, 2 out]
                  }
                }
                n636 = case shown="False" w1376 {
                  tunnel: w1375 -> [w1383 w1386]
                  tunnel: w1374 -> [w1382 w1385]
                  tunnel: [w1381 w1384] -> w1371
                  frame False {
                    n637 = Add(x=w1383, y=w1382) -> (x+y=w1381:dbl)
                  }
                  frame True {
                    n638 = Subtract(x=w1386, y=w1385) -> (x-y=w1384:dbl)
                  }
                }
                n639 = case shown="False" w1372 {
                  tunnel: w1371 -> [w1377 w1379]
                  tunnel: w1370 -> [w1378 _]
                  tunnel: w1369 -> [_ w1380]
                  frame False {
                    n640 = property class="DigNum (strict)"(reference=w1378, "Val(Sgnl)"=w1377) -> ()  [unwired: 1 in, 2 out]
                  }
                  frame True {
                    n641 = property class="DigNum (strict)"(reference=w1380, "Val(Sgnl)"=w1379) -> ()  [unwired: 1 in, 2 out]
                  }
                }
              }
              frame False {
                n642 = case shown="True" w1395 {
                  tunnel: [w1409 w1411] -> w1397
                  tunnel: w1392 -> [w1410 _]
                  tunnel: w1391 -> [_ w1412]
                  frame False {
                    n643 = property class="DigNum (strict)"(reference=w1410) -> ("Value"=w1409:dbl)  [unwired: 1 in, 2 out]
                  }
                  frame True {
                    n644 = property class="DigNum (strict)"(reference=w1412) -> ("Value"=w1411:dbl)  [unwired: 1 in, 2 out]
                  }
                }
                n645 = case shown="True" w1398 {
                  tunnel: w1397 -> [w1405 w1408]
                  tunnel: w1396 -> [w1404 w1407]
                  tunnel: [w1403 w1406] -> w1393
                  frame False {
                    n646 = Subtract(x=w1405, y=w1404) -> (x-y=w1403:dbl)
                  }
                  frame True {
                    n647 = Add(x=w1408, y=w1407) -> (x+y=w1406:dbl)
                  }
                }
                n648 = case shown="False" w1394 {
                  tunnel: w1393 -> [w1399 w1401]
                  tunnel: w1392 -> [w1400 _]
                  tunnel: w1391 -> [_ w1402]
                  frame False {
                    n649 = property class="DigNum (strict)"(reference=w1400, "Val(Sgnl)"=w1399) -> ()  [unwired: 1 in, 2 out]
                  }
                  frame True {
                    n650 = property class="DigNum (strict)"(reference=w1402, "Val(Sgnl)"=w1401) -> ()  [unwired: 1 in, 2 out]
                  }
                }
              }
            }
          }
          frame "ManMove Y" {
            # "Your code here.\n(You can make a copy of, or modify, this frame)"
            n651 = Equal?(x=w1418, y="Down") -> (x = y?=w1422:bool)
            n652 = Unbundle By Name(w1428) -> ("active cams"=w1417:string[], "move properties"=w1427:T2[], "active ccd"=w1416:i32, "active man refs"=w1426:cluster{"Ref X":refnum<vi>, "Ref Y":refnum<vi>})
            n653 = Index Array(array=w1417, index=w1416) -> (element=w1414:string)
            n654 = property on="StepSize" class="DigNum (strict)"() -> ("Value"=w1419:dbl)  [unwired: 2 in, 2 out]
            n655 = Index Array(array=w1427, index=w1416) -> (element=w1429:T2)
            n656 = Unbundle By Name(w1426) -> ("Ref Y"=w1421:refnum<vi>, "Ref X"=w1420:refnum<vi>)
            n657 = Unbundle By Name(w1429) -> ("Invert Direction Y"=w1424:bool, "Invert Axis"=w1423:bool)
            n658 = call <vilib>:"Build State String with Arguments__jki_lib_state_machine.vi"("Arguments (\"\")"=w1414, "State"="Wait" ("State(s) in Front (\"\")")) -> ("State with Arguments"=w1413:string)  [unwired: 4 in]
            n659 = call <vilib>:"Add State(s) to Queue__jki_lib_state_machine.vi"("State(s) in Front (\"\")"=w1413, "State(s) in (\"\")"=w1432) -> ("States Out"=w1431:string)  [unwired: 13 in]
            n660 = case shown="True" w1422 {
              tunnel: w1424 -> [w1440 w1462]
              tunnel: w1419 -> [w1438 w1460]
              tunnel: w1423 -> [w1437 w1459]
              tunnel: w1423 -> [w1436 w1458]
              tunnel: w1421 -> [w1434 w1456]
              tunnel: w1420 -> [w1433 w1455]
              frame True {
                n661 = case shown="True" w1437 {
                  tunnel: [w1451 w1453] -> w1439
                  tunnel: w1434 -> [w1452 _]
                  tunnel: w1433 -> [_ w1454]
                  frame False {
                    n662 = property class="DigNum (strict)"(reference=w1452) -> ("Value"=w1451:dbl)  [unwired: 1 in, 2 out]
                  }
                  frame True {
                    n663 = property class="DigNum (strict)"(reference=w1454) -> ("Value"=w1453:dbl)  [unwired: 1 in, 2 out]
                  }
                }
                n664 = case shown="False" w1440 {
                  tunnel: w1439 -> [w1447 w1450]
                  tunnel: w1438 -> [w1446 w1449]
                  tunnel: [w1445 w1448] -> w1435
                  frame False {
                    n665 = Add(x=w1447, y=w1446) -> (x+y=w1445:dbl)
                  }
                  frame True {
                    n666 = Subtract(x=w1450, y=w1449) -> (x-y=w1448:dbl)
                  }
                }
                n667 = case shown="True" w1436 {
                  tunnel: w1435 -> [w1441 w1443]
                  tunnel: w1434 -> [w1442 _]
                  tunnel: w1433 -> [_ w1444]
                  frame False {
                    n668 = property class="DigNum (strict)"(reference=w1442, "Val(Sgnl)"=w1441) -> ()  [unwired: 1 in, 2 out]
                  }
                  frame True {
                    n669 = property class="DigNum (strict)"(reference=w1444, "Val(Sgnl)"=w1443) -> ()  [unwired: 1 in, 2 out]
                  }
                }
              }
              frame False {
                n670 = case shown="False" w1459 {
                  tunnel: [w1473 w1475] -> w1461
                  tunnel: w1456 -> [w1474 _]
                  tunnel: w1455 -> [_ w1476]
                  frame False {
                    n671 = property class="DigNum (strict)"(reference=w1474) -> ("Value"=w1473:dbl)  [unwired: 1 in, 2 out]
                  }
                  frame True {
                    n672 = property class="DigNum (strict)"(reference=w1476) -> ("Value"=w1475:dbl)  [unwired: 1 in, 2 out]
                  }
                }
                n673 = case shown="False" w1462 {
                  tunnel: w1461 -> [w1469 w1472]
                  tunnel: w1460 -> [w1468 w1471]
                  tunnel: [w1467 w1470] -> w1457
                  frame False {
                    n674 = Subtract(x=w1469, y=w1468) -> (x-y=w1467:dbl)
                  }
                  frame True {
                    n675 = Add(x=w1472, y=w1471) -> (x+y=w1470:dbl)
                  }
                }
                n676 = case shown="False" w1458 {
                  tunnel: w1457 -> [w1463 w1465]
                  tunnel: w1456 -> [w1464 _]
                  tunnel: w1455 -> [_ w1466]
                  frame False {
                    n677 = property class="DigNum (strict)"(reference=w1464, "Val(Sgnl)"=w1463) -> ()  [unwired: 1 in, 2 out]
                  }
                  frame True {
                    n678 = property class="DigNum (strict)"(reference=w1466, "Val(Sgnl)"=w1465) -> ()  [unwired: 1 in, 2 out]
                  }
                }
              }
            }
          }
          frame "Move Y" {
            # "Your code here.\n(You can make a copy of, or modify, this frame)"
            n679 = Unbundle By Name(w1478) -> ("Offset Y"=w1500:dbl[][])
            n680 = call-poly <userlib>:"Filter 1D Array__ogtk.vi"("items to filter"=w1487, "array"=w1504) -> ("filtered item indices"=w1492:i32[])  [unwired: 4 in, 1 out]
            n681 = Unbundle By Name(w1478) -> ("active axis refs 2"=w1503:T11, "move properties"=w1490:T2[])
            n682 = for {
              tunnel: w1492 -> [w1509] mode=indexing
              tunnel: w1490 -> [w1513]
              shift-right: [w1508] -> w1491
              shift-left: i32[] [] ("filtered item indices") -> [w1511]
              n683 = Index Array(array=w1513, index=w1509) -> (element=w1512:T2)
              n684 = Unbundle By Name(w1512) -> ("enable feedback"=w1510:bool)
              n685 = case shown="True" w1510 {
                tunnel: w1511 -> [w1514 w1517]
                tunnel: w1509 -> [_ w1516]
                tunnel: [w1514 w1515] -> w1508
                frame False {
                }
                frame True {
                  n686 = Build Array (concatenate)(w1517, w1516) -> (w1515:i32[])
                }
              }
            }
            n687 = Index Array(array=w1491) -> (element=w1480:i32)  [unwired: 1 in]
            n688 = Index Array(array=w1500, index (row)=w1480) -> (element=w1499:dbl[])  [unwired: 1 in]
            n689 = Reverse 1D Array(array=w1499) -> (reversed array=w1498:dbl[])
            n690 = Index Array(array=w1503, index=w1480) -> (element=w1502:cluster{"Ref X":refnum<vi>, "Ref Y":refnum<vi>})
            n691 = Index Array(array=w1498) -> (element=w1497:dbl)  [unwired: 1 in]
            n692 = Index Array(array=w1490, index=w1480) -> (element=w1501:T2)
            n693 = Unbundle By Name(w1502) -> ("Ref Y"=w1495:refnum<vi>, "Ref X"=w1494:refnum<vi>)
            n694 = Unbundle By Name(w1501) -> ("Invert Direction Y"=w1479:bool, "Invert Axis"=w1485:bool, "enable feedback"=w1493:bool)
            n695 = Greater Or Equal To 0?(x=w1497) -> (x >= 0?=w1496:bool)
            n696 = Unbundle By Name(w1478) -> ("steps speed X"=w1484:dbl[], "steps speed Y"=w1483:dbl[])
            n697 = Index Array(array=w1483, index=w1480) -> (element=w1481:dbl)
            n698 = Index Array(array=w1484, index=w1480) -> (element=w1482:dbl)
            n699 = Select(t=w1482, s=w1479, f=w1481) -> (s? t:f=w1477:dbl)
            n700 = case shown="True" w1493 {
              tunnel: w1485 -> [_ w1523]
              tunnel: w1496 -> [_ w1522]
              tunnel: w1477 -> [_ w1521]
              tunnel: w1479 -> [_ w1520]
              tunnel: w1495 -> [_ w1519]
              tunnel: w1494 -> [_ w1518]
              frame False {
              }
              frame True {
                n701 = case shown="False" w1522 {
                  tunnel: w1520 -> [w1531 w1553]
                  tunnel: w1521 -> [w1529 w1551]
                  tunnel: w1523 -> [w1528 w1550]
                  tunnel: w1523 -> [w1527 w1549]
                  tunnel: w1519 -> [w1525 w1547]
                  tunnel: w1518 -> [w1524 w1546]
                  frame True {
                    n702 = case shown="False" w1528 {
                      tunnel: [w1542 w1544] -> w1530
                      tunnel: w1525 -> [w1543 _]
                      tunnel: w1524 -> [_ w1545]
                      frame False {
                        n703 = property class="DigNum (strict)"(reference=w1543) -> ("Value"=w1542:dbl)  [unwired: 1 in, 2 out]
                      }
                      frame True {
                        n704 = property class="DigNum (strict)"(reference=w1545) -> ("Value"=w1544:dbl)  [unwired: 1 in, 2 out]
                      }
                    }
                    n705 = case shown="False" w1531 {
                      tunnel: w1530 -> [w1538 w1541]
                      tunnel: w1529 -> [w1537 w1540]
                      tunnel: [w1536 w1539] -> w1526
                      frame False {
                        n706 = Add(x=w1538, y=w1537) -> (x+y=w1536:dbl)
                      }
                      frame True {
                        n707 = Subtract(x=w1541, y=w1540) -> (x-y=w1539:dbl)
                      }
                    }
                    n708 = case shown="False" w1527 {
                      tunnel: w1526 -> [w1532 w1534]
                      tunnel: w1525 -> [w1533 _]
                      tunnel: w1524 -> [_ w1535]
                      frame False {
                        n709 = property class="DigNum (strict)"(reference=w1533, "Val(Sgnl)"=w1532) -> ()  [unwired: 1 in, 2 out]
                      }
                      frame True {
                        n710 = property class="DigNum (strict)"(reference=w1535, "Val(Sgnl)"=w1534) -> ()  [unwired: 1 in, 2 out]
                      }
                    }
                  }
                  frame False {
                    n711 = case shown="False" w1550 {
                      tunnel: [w1564 w1566] -> w1552
                      tunnel: w1547 -> [w1565 _]
                      tunnel: w1546 -> [_ w1567]
                      frame False {
                        n712 = property class="DigNum (strict)"(reference=w1565) -> ("Value"=w1564:dbl)  [unwired: 1 in, 2 out]
                      }
                      frame True {
                        n713 = property class="DigNum (strict)"(reference=w1567) -> ("Value"=w1566:dbl)  [unwired: 1 in, 2 out]
                      }
                    }
                    n714 = case shown="False" w1553 {
                      tunnel: w1552 -> [w1560 w1563]
                      tunnel: w1551 -> [w1559 w1562]
                      tunnel: [w1558 w1561] -> w1548
                      frame False {
                        n715 = Subtract(x=w1560, y=w1559) -> (x-y=w1558:dbl)
                      }
                      frame True {
                        n716 = Add(x=w1563, y=w1562) -> (x+y=w1561:dbl)
                      }
                    }
                    n717 = case shown="True" w1549 {
                      tunnel: w1548 -> [w1554 w1556]
                      tunnel: w1547 -> [w1555 _]
                      tunnel: w1546 -> [_ w1557]
                      frame False {
                        n718 = property class="DigNum (strict)"(reference=w1555, "Val(Sgnl)"=w1554) -> ()  [unwired: 1 in, 2 out]
                      }
                      frame True {
                        n719 = property class="DigNum (strict)"(reference=w1557, "Val(Sgnl)"=w1556) -> ()  [unwired: 1 in, 2 out]
                      }
                    }
                  }
                }
              }
            }
            n720 = call <vilib>:"Build State String with Arguments__jki_lib_state_machine.vi"("Arguments (\"\")"=w1487, "State"="Wait" ("State(s) in Front (\"\")")) -> ("State with Arguments"=w1486:string)  [unwired: 4 in]
            n721 = call <vilib>:"Add State(s) to Queue__jki_lib_state_machine.vi"("State(s) in Front (\"\")"=w1486, "State(s) in (\"\")"=w1507) -> ("States Out"=w1506:string)  [unwired: 13 in]
            "Moving Y" <- w1487
          }
          frame "Wait" {
            # "Your code here.\n(You can make a copy of, or modify, this frame)"
            n722 = flat-sequence {
              tunnel: T18."Disabled and Grayed Out" ("Disabled") -> [w1584]
              tunnel: w1574 -> [w1593]
              tunnel: w1573 -> [w1592]
              tunnel: [w1591] -> w1572
              tunnel: w1571 -> [w1590]
              tunnel: w1570 -> [w1589]
              tunnel: T18."Enabled" ("Disabled") -> [w1603]
              frame #0 {
                n723 = property on="Right" class="Bool (strict)"("DisabledEnum"=w1584) -> ()  [unwired: 2 in, 2 out]
                n724 = property on="Up" class="Bool (strict)"("DisabledEnum"=w1584) -> ()  [unwired: 2 in, 2 out]
                n725 = property on="Left" class="Bool (strict)"("DisabledEnum"=w1584) -> ()  [unwired: 2 in, 2 out]
                n726 = property on="Down" class="Bool (strict)"("DisabledEnum"=w1584) -> ()  [unwired: 2 in, 2 out]
                n727 = property on="StepSize" class="DigNum (strict)"("DisabledEnum"=w1584) -> ()  [unwired: 2 in, 2 out]
              }
              frame #1 {
                n728 = Wait (ms)(milliseconds to wait=u32 1500) -> ()  [unwired: 1 out]
              }
              frame #2 {
                n729 = property on="Moving Y" class="Str"("Value"="") -> ()  [unwired: 2 in, 2 out]
                n730 = property on="Moving X" class="Str"("Value"="") -> ()  [unwired: 2 in, 2 out]
              }
              frame #3 {
                n731 = Equal?(x=w1589, y=w1590) -> (x = y?=w1588:bool)
                n732 = case shown="True" w1588 {
                  tunnel: w1593 -> [_ w1600]
                  tunnel: w1592 -> [w1594 w1597]
                  tunnel: [w1594 w1595] -> w1591
                  frame False {
                  }
                  frame True {
                    n733 = Unbundle By Name(w1600) -> ("Ref X"=w1599:refnum<vi>, "Ref Y"=w1598:refnum<vi>)
                    n734 = property class="DigNum (strict)"(reference=w1599, error in=w1597) -> (error out=w1596:errorcluster, "Value"=w1602:dbl)  [unwired: 1 out]
                    n735 = property class="DigNum (strict)"(reference=w1598, error in=w1596) -> (error out=w1595:errorcluster, "Value"=w1601:dbl)  [unwired: 1 out]
                    n736 = property on="Position 1" class="DigNum (strict)"("Value"=w1602) -> ()  [unwired: 2 in, 2 out]
                    n737 = property on="Position 2" class="DigNum (strict)"("Value"=w1601) -> ()  [unwired: 2 in, 2 out]
                  }
                }
              }
              frame #4 {
                n738 = property on="Right" class="Bool (strict)"("DisabledEnum"=w1603) -> ()  [unwired: 2 in, 2 out]
                n739 = property on="Up" class="Bool (strict)"("DisabledEnum"=w1603) -> ()  [unwired: 2 in, 2 out]
                n740 = property on="Left" class="Bool (strict)"("DisabledEnum"=w1603) -> ()  [unwired: 2 in, 2 out]
                n741 = property on="Down" class="Bool (strict)"("DisabledEnum"=w1603) -> ()  [unwired: 2 in, 2 out]
                n742 = property on="StepSize" class="DigNum (strict)"("DisabledEnum"=w1603) -> ()  [unwired: 2 in, 2 out]
              }
            }
            n743 = call-poly <userlib>:"Filter 1D Array__ogtk.vi"("items to filter"=w1577, "array"=w1578) -> ("filtered item indices"=w1576:i32[])  [unwired: 4 in, 1 out]
            n744 = Index Array(array=w1576) -> (element=w1571:i32)  [unwired: 1 in]
            n745 = Unbundle By Name(w1579) -> ("active axis refs 2"=w1575:T11, "active ccd"=w1570:i32)
            n746 = Index Array(array=w1575, index=w1571) -> (element=w1574:cluster{"Ref X":refnum<vi>, "Ref Y":refnum<vi>})
            n747 = call <vilib>:"Add State(s) to Queue__jki_lib_state_machine.vi"("State(s) in (\"\")"=w1583) -> ("States Out"=w1582:string)  [unwired: 14 in]
            n748 = local read "Mean Centroid X"() -> (w1580:dbl[][])
            n749 = Bundle By Name(cluster=w1579, "Mean Centroid X"=w1580, "Mean Centroid Y"=w1580) -> (w1581:T35)
          }
          frame "---------------Statistics--------------" {
            # "Template Separator\n(You can make a copy of, or modify, this frame)"
            n750 = call <vilib>:"Add State(s) to Queue__jki_lib_state_machine.vi"("State(s) in (\"\")"=w1607) -> ("States Out"=w1606:string)  [unwired: 14 in]
          }
          frame "Save Stats" {
            # "Your code here.\n(You can make a copy of, or modify, this frame)"
            n751 = property on="CCD 1" class="XYGraph (strict)"() -> ("Value"=w1618:cluster{timestamp[], dbl[]}[])  [unwired: 2 in, 2 out]
            n752 = property on="CCD 2" class="XYGraph (strict)"() -> ("Value"=w1617:cluster{timestamp[], dbl[]}[])  [unwired: 2 in, 2 out]
            n753 = property on="CCD 3" class="XYGraph (strict)"() -> ("Value"=w1616:cluster{timestamp[], dbl[]}[])  [unwired: 2 in, 2 out]
            n754 = property on="CCD 4" class="XYGraph (strict)"() -> ("Value"=w1615:cluster{timestamp[], dbl[]}[])  [unwired: 2 in, 2 out]
            n755 = property on="CCD 5" class="XYGraph (strict)"() -> ("Value"=w1614:cluster{timestamp[], dbl[]}[])  [unwired: 2 in, 2 out]
            n756 = property on="CCD 6" class="XYGraph (strict)"() -> ("Value"=w1613:cluster{timestamp[], dbl[]}[])  [unwired: 2 in, 2 out]
            n757 = property on="CCD 7" class="XYGraph (strict)"() -> ("Value"=w1612:cluster{timestamp[], dbl[]}[])  [unwired: 2 in, 2 out]
            n758 = property on="CCD 8" class="XYGraph (strict)"() -> ("Value"=w1611:cluster{timestamp[], dbl[]}[])  [unwired: 2 in, 2 out]
            n759 = Build Array(w1618, w1617, w1616, w1615, w1614, w1613, w1612, w1611) -> (w1610:cluster{timestamp[], dbl[]}[][])
            n760 = disable-structure shown="Disabled" {
              disable-tunnel: w1622 -> [w1626 _]
              disable-tunnel: [w1625 _] -> w1621
              disable-tunnel: w1610 -> [w1624 _]
              disable-tunnel: w1609 -> [w1623 _]
              frame Disabled {
                n761 = for {
                  tunnel: w1624 -> [w1629] mode=indexing
                  tunnel: w1623 -> [w1628] mode=indexing
                  n762 = Empty String/Path?(string/path=w1628) -> (empty?=w1627:bool)
                  n763 = case shown="False" w1627 {
                    tunnel: w1629 -> [w1635 _]
                    tunnel: w1628 -> [w1633 _]
                    frame False {
                      n764 = Index Array(array=w1635, index #1=0 ("index"), index #2=1 ("index"), index #3=2 ("index"), index #4=3 ("index")) -> (element #1=w1670:cluster{timestamp[], dbl[]}, element #2=w1664:cluster{timestamp[], dbl[]}, element #3=w1663:cluster{timestamp[], dbl[]}, element #4=w1662:cluster{timestamp[], dbl[]})  [unwired: 1 in, 1 out]
                      n765 = Concatenate Strings(w1633, ".dat" ("string")) -> (w1631:string)
                      n766 = Unbundle(w1670) -> (w1669:timestamp[], w1647:dbl[])
                      n767 = Unbundle(w1664) -> (w1638:dbl[])  [unwired: 1 out]
                      n768 = Unbundle(w1663) -> (w1637:dbl[])  [unwired: 1 out]
                      n769 = Unbundle(w1662) -> (w1636:dbl[])  [unwired: 1 out]
                      n770 = Build Path(base path="save path", name or relative path=w1631) -> (appended path=w1630:path)
                      n771 = for {
                        tunnel: w1669 -> [w1672] mode=indexing
                        tunnel: [w1671] -> w1645 mode=indexing
                        n772 = Format Date/Time String(time format string (%c)="%Y%m%d%H%M%S", seconds (now)=w1672) -> (date/time string=w1671:string)  [unwired: 1 in]
                      }
                      n773 = Array Size(array=w1647) -> (size(s)=w1648:i32)
                      n774 = Number To Fractional String(number=w1647) -> (F-format string=w1644:string[])  [unwired: 3 in]
                      n775 = Number To Fractional String(number=w1638) -> (F-format string=w1641:string[])  [unwired: 3 in]
                      n776 = Number To Fractional String(number=w1637) -> (F-format string=w1640:string[])  [unwired: 3 in]
                      n777 = Number To Fractional String(number=w1636) -> (F-format string=w1639:string[])  [unwired: 3 in]
                      n778 = Initialize Array("", w1648, 5 ("dimension size")) -> (w1646:string[][])
                      n779 = Insert Into Array(array=w1646, index (col)=0 ("disabled index (col)"), new element=w1645) -> (w1656:string[][])  [unwired: 1 in]
                      n780 = Insert Into Array(array=w1656, index (col)=1 ("disabled index (col)"), new element=w1644) -> (w1655:string[][])  [unwired: 1 in]
                      n781 = Insert Into Array(array=w1655, index (col)=2 ("disabled index (col)"), new element=w1641) -> (w1659:string[][])  [unwired: 1 in]
                      n782 = Insert Into Array(array=w1659, index (col)=3 ("disabled index (col)"), new element=w1640) -> (w1660:string[][])  [unwired: 1 in]
                      n783 = Insert Into Array(array=w1660, index (col)=4 ("disabled index (col)"), new element=w1639) -> (w1661:string[][])  [unwired: 1 in]
                      n784 = Insert Into Array(array=w1661, index (row)=0, new element=string[] ["time", "Centroid X", "Centroid Y", "Motor Axis 1", "Motor Axis 2"] ("new element/subarray 2")) -> (w1643:string[][])  [unwired: 1 in]
                      n785 = call-poly <vilib>:"Write To Spreadsheet File.vi"("2D data"=w1643, "file path (dialog if empty)"=w1630) -> ()  [unwired: 6 in, 1 out]
                    }
                    frame True {
                    }
                  }
                }
                n786 = call <vilib>:"Add State(s) to Queue__jki_lib_state_machine.vi"("State(s) in (\"\")"=w1626) -> ("States Out"=w1625:string)  [unwired: 14 in]
              }
              frame Enabled {
              }
            }
            n787 = property on="Save Stats" class="Bool (strict)"("Value"=FALSE ("Save Stats")) -> ()  [unwired: 2 in, 2 out]
          }
          frame "tdms" {
            w1684 = 21600.0 ("new tdms")
            # "Your code here.\n(You can make a copy of, or modify, this frame)"
            n788 = Unbundle By Name(w1692) -> ("active cams"=w1677:string[], "Data Value Reference out"=w1674:refnum<k34>, "Offset X"=w1691:dbl[][], "Offset Y"=w1690:dbl[][], "active axis refs 2"=w1689:T11)
            n789 = for {
              tunnel: w1691 -> [w1739]
              tunnel: w1690 -> [w1738]
              tunnel: w1677 -> [w1702] mode=indexing
              tunnel: w1674 -> [w1703]
              tunnel: w1689 -> [w1724]
              tunnel: w1694 -> [w1708]
              tunnel: [w1706] -> w1693
              i -> [w1725]
              n790 = Index Array(array=w1739, index (row)=w1725) -> (element=w1737:dbl[])  [unwired: 1 in]
              n791 = Index Array(array=w1738, index (row)=w1725) -> (element=w1736:dbl[])  [unwired: 1 in]
              n792 = Index Array(array=w1724, index=w1725) -> (element=w1723:cluster{"Ref X":refnum<vi>, "Ref Y":refnum<vi>})
              n793 = Reverse 1D Array(array=w1736) -> (reversed array=w1734:dbl[])
              n794 = Reverse 1D Array(array=w1737) -> (reversed array=w1735:dbl[])
              n795 = Unbundle By Name(w1723) -> ("Ref X"=w1722:refnum<vi>, "Ref Y"=w1721:refnum<vi>)
              n796 = Index Array(array=w1735) -> (element=w1733:dbl)  [unwired: 1 in]
              n797 = Index Array(array=w1734) -> (element=w1732:dbl)  [unwired: 1 in]
              n798 = property class="DigNum (strict)"(reference=w1722, error in=w1708) -> (error out=w1707:errorcluster, "Value"=w1716:dbl)  [unwired: 1 out]
              n799 = Build Array(w1733) -> (w1705:dbl[])
              n800 = Build Array(w1732) -> (w1727:dbl[])
              n801 = Get Date/Time In Seconds() -> (seconds since 1Jan1904=w1704:timestamp)
              n802 = Build Array(w1704) -> (w1700:timestamp[])
              n803 = property class="DigNum (strict)"(reference=w1721, error in=w1707) -> (error out=w1698:errorcluster, "Value"=w1710:dbl)  [unwired: 1 out]
              n804 = Build Array(w1716) -> (w1715:dbl[])
              n805 = TDMS Write(0:w1703, 5:w1702, 7:"time", 9:w1700, 11:w1698) -> (4:w1699:refnum<k34>, 15:w1697:errorcluster)  [unwired: 1 in, 2 out]
              n806 = Build Array(w1710) -> (w1709:dbl[])
              n807 = TDMS Write(0:w1699, 5:w1702, 7:"centroid X", 9:w1705, 11:w1697) -> (4:w1730:refnum<k34>, 6:w1729:string, 15:w1728:errorcluster)  [unwired: 1 in, 1 out]
              n808 = TDMS Write(0:w1730, 5:w1729, 7:"centroid Y", 9:w1727, 11:w1728) -> (4:w1719:refnum<k34>, 6:w1718:string, 15:w1720:errorcluster)  [unwired: 1 in, 1 out]
              n809 = TDMS Write(0:w1719, 5:w1718, 7:"Motor Axis 1", 9:w1715, 11:w1720) -> (4:w1714:refnum<k34>, 6:w1713:string, 15:w1711:errorcluster)  [unwired: 1 in, 1 out]
              n810 = TDMS Write(0:w1714, 5:w1713, 7:"Motor Axis 2", 9:w1709, 11:w1711) -> (15:w1706:errorcluster)  [unwired: 1 in, 3 out]
            }
            n811 = property on="millisecond timer value" class="DigNum (strict)"() -> ("Value"=w1676:u32)  [unwired: 2 in, 2 out]
            n812 = Tick Count (ms)() -> (millisecond timer value=w1675:u32)
            n813 = Unbundle By Name(w1692) -> ()  [unwired: 1 out]
            n814 = Subtract(x=w1675, y=w1676) -> (x-y=w1679:u32)
            n815 = Divide(x=w1679, y=u32 1000) -> (x/y=w1681:dbl)
            n816 = Quotient & Remainder(x=w1681, y=w1684) -> (x-y*floor(x/y)=w1682:dbl)  [unwired: 1 out]
            n817 = Subtract(x=w1684, y=20.0) -> (x-y=w1686:dbl)
            n818 = Greater?(x=w1682, y=w1686) -> (0:w1683:bool)
            n819 = Select(t="newtdms", s=w1683, f="") -> (s? t:f=w1678:string)
            n820 = call <vilib>:"Add State(s) to Queue__jki_lib_state_machine.vi"("State(s) in (\"\")"=w1696, "State(s) at Back (\"\")"=w1678) -> ("States Out"=w1695:string)  [unwired: 13 in]
          }
          frame "Reset History" {
            # "Your code here.\n(You can make a copy of, or modify, this frame)"
            n821 = for {
              N: 1 -> [_]
              shift-right: [w1749] -> w1741
              shift-left: timestamp[][] [] ("Time") -> [w1751]
              n822 = for {
                N: 12 -> [_]
                tunnel: w1751 -> [w1754] mode=indexing
                tunnel: [w1752] -> w1749 mode=indexing
                n823 = Get Date/Time In Seconds() -> (seconds since 1Jan1904=w1753:timestamp)
                n824 = Build Array (concatenate)(w1754, w1753) -> (w1752:timestamp[])
              }
            }
            n825 = local read "Offset X"() -> (w1740:dbl[][])
            n826 = Bundle By Name(cluster=w1745, "Offset X"=w1740, "Offset Y"=w1740, "Time"=w1741, "Motor X"=w1740) -> (w1744:T35)
            n827 = call <vilib>:"Add State(s) to Queue__jki_lib_state_machine.vi"("State(s) in (\"\")"=w1748) -> ("States Out"=w1747:string)  [unwired: 14 in]
          }
          frame "New Category: 2" {
            # "Your code here.\n(You can make a copy of, or modify, this frame)"
            n828 = call <vilib>:"Add State(s) to Queue__jki_lib_state_machine.vi"("State(s) in (\"\")"=w1758) -> ("States Out"=w1757:string)  [unwired: 14 in]
          }
          frame "stats" {
            # "Your code here.\n(You can make a copy of, or modify, this frame)"
            n829 = Unbundle By Name(w1773) -> ("Offset X"=w1764:dbl[][], "Offset Y"=w1763:dbl[][], "Time"=w1762:timestamp[][], "Motor X"=w1761:dbl[][], "Motor Y"=w1760:dbl[][], "Data Value Reference out"=w1768:refnum<k34>)
            n830 = TDMS List Contents(4:w1767, 7:w1768) -> (0:w1759:errorcluster, 2:w1771:string[], 3:w1770:refnum<k34>)  [unwired: 1 in, 1 out]
            n831 = call <vilib>:"ClearError.vi"("error in (no error)"=w1759) -> ("error out"=w1769:errorcluster)
            n832 = for {
              tunnel: w1769 -> [w1840]
              tunnel: [w1826] -> w1765 mode=indexing
              tunnel: [w1825] -> w1766
              tunnel: [w1824] -> _
              tunnel: w1770 -> [w1823]
              tunnel: w1771 -> [w1822] mode=indexing
              w1841 = dbl[] [] ("appended array")
              n833 = TDMS Read(0:w1823, 5:w1822, 7:"time", 11:w1840, 12:timestamp[] [] ("appended array")) -> (4:w1855:refnum<k34>, 6:w1851:string, 10:w1832:timestamp[], 15:w1839:errorcluster)  [unwired: 3 in, 2 out]
              n834 = TDMS Read(0:w1855, 5:w1851, 7:"centroid X", 11:w1839, 12:w1841) -> (4:w1854:refnum<k34>, 6:w1850:string, 10:w1835:dbl[], 15:w1838:errorcluster)  [unwired: 3 in, 2 out]
              n835 = TDMS Read(0:w1854, 5:w1850, 7:"centroid Y", 11:w1838, 12:w1841) -> (4:w1853:refnum<k34>, 6:w1849:string, 10:w1834:dbl[], 15:w1837:errorcluster)  [unwired: 3 in, 2 out]
              n836 = TDMS Read(0:w1853, 5:w1849, 7:"Motor Axis 1", 11:w1837, 12:w1841) -> (4:w1852:refnum<k34>, 6:w1848:string, 10:w1833:dbl[], 15:w1836:errorcluster)  [unwired: 3 in, 2 out]
              n837 = TDMS Read(0:w1852, 5:w1848, 7:"Motor Axis 2", 11:w1836, 12:w1841) -> (4:w1824:refnum<k34>, 10:w1831:dbl[], 15:w1825:errorcluster)  [unwired: 3 in, 3 out]
              n838 = Bundle("appended array"=w1832, "appended array"=w1835) -> (w1830:T37)  [unwired: 1 in]
              n839 = Bundle("appended array"=w1832, "appended array"=w1834) -> (w1829:T37)  [unwired: 1 in]
              n840 = Bundle("appended array"=w1832, "appended array"=w1833) -> (w1828:T37)  [unwired: 1 in]
              n841 = Bundle("appended array"=w1832, "appended array"=w1831) -> (w1827:T37)  [unwired: 1 in]
              n842 = Build Array(w1830, w1829, w1828, w1827) -> (w1826:T38)
            }
            n843 = disable-structure shown="Disabled" {
              disable-tunnel: w1772 -> [w1805 _]
              disable-tunnel: w1764 -> [w1804 _]
              disable-tunnel: w1763 -> [w1803 _]
              disable-tunnel: w1762 -> [w1802 _]
              disable-tunnel: w1761 -> [w1801 _]
              disable-tunnel: w1760 -> [w1800 _]
              frame Disabled {
                n844 = for {
                  tunnel: w1805 -> [_] mode=indexing
                  tunnel: w1804 -> [w1815]
                  tunnel: w1803 -> [w1814]
                  tunnel: w1802 -> [w1813]
                  tunnel: w1801 -> [w1809]
                  tunnel: w1800 -> [w1808]
                  tunnel: [w1817] -> _ mode=indexing
                  i -> [w1816]
                  n845 = Index Array(array=w1814, index (row)=w1816) -> (element=w1810:dbl[])  [unwired: 1 in]
                  n846 = Index Array(array=w1809, index (row)=w1816) -> (element=w1807:dbl[])  [unwired: 1 in]
                  n847 = Index Array(array=w1808, index (row)=w1816) -> (element=w1806:dbl[])  [unwired: 1 in]
                  n848 = Index Array(array=w1815, index (row)=w1816) -> (element=w1811:dbl[])  [unwired: 1 in]
                  n849 = Index Array(array=w1813, index (row)=w1816) -> (element=w1812:timestamp[])  [unwired: 1 in]
                  n850 = Bundle("Time"=w1812, "Motor X"=w1807) -> (w1820:cluster{"Time":timestamp[], "Motor X":dbl[]})  [unwired: 1 in]
                  n851 = Bundle("Time"=w1812, "Motor Y"=w1806) -> (w1821:cluster{"Time":timestamp[], "Motor Y":dbl[]})  [unwired: 1 in]
                  n852 = Bundle("Time"=w1812, "Offset X"=w1811) -> (w1819:cluster{"Time":timestamp[], "Offset X":dbl[]})  [unwired: 1 in]
                  n853 = Bundle("Time"=w1812, "Offset Y"=w1810) -> (w1818:cluster{"Time":timestamp[], "Offset Y":dbl[]})  [unwired: 1 in]
                  n854 = Build Array(w1818, w1819, w1820, w1821) -> (w1817:cluster{"Time":timestamp[], "Motor Y":dbl[]}[])
                }
              }
              frame Enabled {
              }
            }
            n855 = Index Array(array=w1765, index (row) #1=0 ("index (row)"), index (row) #2=1 ("index (row)"), index (row) #3=2 ("index (row)"), index (row) #4=3 ("index (row)"), index (row) #5=4 ("index (row)"), index (row) #6=5 ("index (row)"), index (row) #7=6 ("index (row)"), index (row) #8=7 ("index (row)"), index (row) #9=8 ("index (row)"), index (row) #10=9 ("index (row)"), index (row) #11=10 ("index (row)"), index (row) #12=11 ("index (row)")) -> (element #1=→"CCD 1":T38, element #2=→"CCD 2":T38, element #3=→"CCD 3":T38, element #4=→"CCD 4":T38, element #5=→"CCD 5":T38, element #6=→"CCD 6":T38, element #7=→"CCD 7":T38, element #8=→"CCD 8":T38, element #9=→"CCD 9":T38, element #10=→"CCD 10":T38, element #11=→"CCD 11":T38, element #12=→"CCD 12":T38)  [unwired: 12 in]
            n856 = call <vilib>:"Add State(s) to Queue__jki_lib_state_machine.vi"("State(s) in (\"\")"=w1799) -> ("States Out"=w1798:string)  [unwired: 14 in]
          }
          frame "newtdms" {
            # "Your code here.\n(You can make a copy of, or modify, this frame)"
            n857 = Unbundle By Name(w1892) -> ("Data Value Reference out"=w1880:refnum<k34>, "active cams"=w1875:string[])
            n858 = TDMS Close(8:w1890, 11:w1880) -> (0:w1874:errorcluster)  [unwired: 1 out]
            n859 = Get Date/Time In Seconds() -> (seconds since 1Jan1904=w1868:timestamp)
            n860 = call <vilib>:"Clear Errors.vi"("error in (no error)"=w1874) -> ("error out"=w1861:errorcluster)  [unwired: 5 in, 1 out]
            n861 = Format Date/Time String(time format string (%c)="%Y%m%d", seconds (now)=w1868) -> (date/time string=w1869:string)  [unwired: 1 in]
            n862 = Format Date/Time String(time format string (%c)="%Y%m%d%H%M", seconds (now)=w1868) -> (date/time string=w1866:string)  [unwired: 1 in]
            n863 = property on="new tdms" class="Bool (strict)"("Value"=FALSE ("new tdms")) -> ()  [unwired: 2 in, 2 out]
            n864 = Get Date/Time In Seconds() -> (seconds since 1Jan1904=w1889:timestamp)
            n865 = Format Date/Time String(time format string (%c)="%Y%m%d%H%M", seconds (now)=w1889) -> (date/time string=w1881:string)  [unwired: 1 in]
            n866 = Build Path(base path=w1862, name or relative path=w1869) -> (appended path=w1870:path)
            n867 = Concatenate Strings(w1881, "BeampointingBELLABTL_TRA.tdms" ("string")) -> (w1887:string)
            n868 = String To Path(string=w1887) -> ()  [unwired: 1 out]
            n869 = Concatenate Strings(w1866, "BeampointingBELLABTL_TRA.tdms" ("string")) -> (w1864:string)
            n870 = String To Path(string=w1864) -> (path=w1859:path)
            n871 = call <vilib>:"Check if File or Folder Exists.vi"("error in (no error)"=w1861, "path"=w1870) -> ("error out"=w1873:errorcluster, "file or folder exists?"=w1871:bool, "dup path"=w1872:path)  [unwired: 7 in]
            n872 = case shown="False" w1871 {
              tunnel: w1872 -> [w1898 w1900]
              tunnel: [w1897 w1900] -> w1858
              tunnel: w1873 -> [w1896 w1899]
              tunnel: [w1895 w1899] -> w1860
              frame False {
                n873 = Create Folder(path (use dialog)=w1898, error in=w1896) -> (created path=w1897:path, error out=w1895:errorcluster)  [unwired: 1 in, 1 out]
              }
              frame True {
              }
            }
            n874 = call <vilib>:"Add State(s) to Queue__jki_lib_state_machine.vi"("State(s) in (\"\")"=w1894) -> ("States Out"=w1893:string)  [unwired: 14 in]
            n875 = Build Path(base path=w1858, name or relative path=w1859) -> (appended path=w1882:path)
            n876 = TDMS Open(6:FALSE ("disable buffering (T)"), 7:enum16{"1.0", "2.0"}."2.0" ("file format version (2.0)"), 8:w1860, 10:T15."create or replace" ("operation"), 11:w1882) -> (0:w1878:errorcluster, 3:w1877:refnum<k34>)  [unwired: 2 in]
            n877 = call "TDMSbuffersize.vi"("error in (no error)"=w1878, "group names"=w1875, "Data Value Reference in"=w1877) -> ("error out"=w1857:errorcluster, "Data Value Reference out"=w1876:refnum<k34>)  [unwired: 7 in]
            n878 = Bundle By Name(cluster=w1892, "Data Value Reference out"=w1876) -> (w1891:T35)
            n879 = call <vilib>:"Clear Errors.vi"("error in (no error)"=w1857) -> ("error out"=w1856:errorcluster)  [unwired: 5 in, 1 out]
          }
          frame "Center" {
            # "Your code here.\n(You can make a copy of, or modify, this frame)"
            n880 = control-ref of="image::1"() -> (w1915:refnum<vi>)
            n881 = control-ref of="image::2"() -> (w1914:refnum<vi>)
            n882 = control-ref of="image::3"() -> (w1913:refnum<vi>)
            n883 = control-ref of="image::4"() -> (w1912:refnum<vi>)
            n884 = control-ref of="image::5"() -> (w1911:refnum<vi>)
            n885 = control-ref of="image::6"() -> (w1910:refnum<vi>)
            n886 = control-ref of="image::7"() -> (w1909:refnum<vi>)
            n887 = control-ref of="image::8"() -> (w1908:refnum<vi>)
            n888 = control-ref of="image::9"() -> (w1907:refnum<vi>)
            n889 = control-ref of="image::10"() -> (w1906:refnum<vi>)
            n890 = control-ref of="image::11"() -> (w1905:refnum<vi>)
            n891 = control-ref of="image::12"() -> (w1904:refnum<vi>)
            n892 = for {
              tunnel: [w1924] -> w1903 mode=indexing
              tunnel: w1902 -> [w1923] mode=indexing
              n893 = Unbundle By Name(w1923) -> ("Target.X::12"=w1922:refnum<vi>, "Target.Y::12"=w1921:refnum<vi>)
              n894 = property class="DigNum (strict)"(reference=w1922) -> ("Value"=w1925:dbl)  [unwired: 1 in, 2 out]
              n895 = property class="DigNum (strict)"(reference=w1921) -> ("Value"=w1926:dbl)  [unwired: 1 in, 2 out]
              n896 = Bundle("Value"=w1925, "Value"=w1926) -> (w1924:cluster{"Value":dbl, "Value":dbl})  [unwired: 1 in]
            }
            n897 = call <vilib>:"Add State(s) to Queue__jki_lib_state_machine.vi"("State(s) in (\"\")"=w1920) -> ("States Out"=w1919:string)  [unwired: 14 in]
            n898 = Build Array(w1915, w1914, w1913, w1912, w1911, w1910, w1909, w1908, w1907, w1906, w1905, w1904) -> (w1916:refnum<vi>[])
            n899 = for {
              tunnel: w1916 -> [w1928] mode=indexing
              tunnel: w1903 -> [w1927] mode=indexing
              n900 = property class="ImageControl"(reference=w1928, "Image Center Position"=w1927) -> ()  [unwired: 1 in, 2 out]
            }
            n901 = property on="Center" class="Bool (strict)"("Value"=FALSE ("Center")) -> ()  [unwired: 2 in, 2 out]
          }
          frame "ImgToAvg" {
            n902 = Decimal String To Number(string=w1938) -> (number=w1935:i32)  [unwired: 2 in, 1 out]
            n903 = Bundle By Name(cluster=w1937, "img to avg"=w1935) -> (w1936:T35)
            n904 = call <vilib>:"Build State String with Arguments__jki_lib_state_machine.vi"("Arguments (\"\")"="T" ("Arguments (\"\")"), "State"=" Device Ini") -> ("State with Arguments"=w1929:string)  [unwired: 4 in]
            n905 = call <vilib>:"Add State(s) to Queue__jki_lib_state_machine.vi"("State(s) in Front (\"\")"=w1929, "State(s) in (\"\")"=w1934) -> ("States Out"=w1933:string)  [unwired: 13 in]
          }
          frame "history" {
            # "Your code here.\n(You can make a copy of, or modify, this frame)"
            n906 = Unbundle By Name(w1948) -> ("Offset X"=w1954:dbl[][], "Offset Y"=w1953:dbl[][], "Mean Centroid X"=w1952:dbl[][], "Mean Centroid Y"=w1951:dbl[][], "Motor X"=w1950:dbl[][], "Motor Y"=w1949:dbl[][], "Time"=w1940:timestamp[][])
            n907 = for {
              tunnel: w1954 -> [w1972] mode=indexing
              tunnel: w1953 -> [w1970] mode=indexing
              tunnel: w1952 -> [w1969] mode=indexing
              tunnel: w1951 -> [w1968] mode=indexing
              tunnel: w1950 -> [w1967] mode=indexing
              tunnel: w1949 -> [w1966] mode=indexing
              tunnel: [w1971] -> w1946 mode=indexing
              tunnel: [w1965] -> w1945 mode=indexing
              tunnel: [w1961] -> w1944 mode=indexing
              tunnel: [w1964] -> w1943 mode=indexing
              tunnel: [w1963] -> w1942 mode=indexing
              tunnel: [w1962] -> w1941 mode=indexing
              tunnel: w1940 -> [w1960] mode=indexing
              tunnel: [w1958] -> w1939 mode=indexing
              w1959 = 0
              n908 = Delete From Array(array=w1967, index=w1959) -> (array with subset deleted=w1963:dbl[])  [unwired: 1 in, 1 out]
              n909 = Delete From Array(array=w1966, index=w1959) -> (array with subset deleted=w1962:dbl[])  [unwired: 1 in, 1 out]
              n910 = Delete From Array(array=w1960, index=w1959) -> (array with subset deleted=w1958:timestamp[])  [unwired: 1 in, 1 out]
              n911 = Delete From Array(array=w1969, index=w1959) -> (array with subset deleted=w1961:dbl[])  [unwired: 1 in, 1 out]
              n912 = Delete From Array(array=w1968, index=w1959) -> (array with subset deleted=w1964:dbl[])  [unwired: 1 in, 1 out]
              n913 = Delete From Array(array=w1970, index=w1959) -> (array with subset deleted=w1965:dbl[])  [unwired: 1 in, 1 out]
              n914 = Delete From Array(array=w1972, index=w1959) -> (array with subset deleted=w1971:dbl[])  [unwired: 1 in, 1 out]
            }
            n915 = call <vilib>:"Add State(s) to Queue__jki_lib_state_machine.vi"("State(s) in (\"\")"=w1957) -> ("States Out"=w1956:string)  [unwired: 14 in]
            n916 = Bundle By Name(cluster=w1948, "Offset X"=w1946, "Offset Y"=w1945, "Mean Centroid X"=w1944, "Mean Centroid Y"=w1943, "Motor X"=w1942, "Motor Y"=w1941, "Time"=w1939) -> (w1947:T35)
          }
        }
        n917 = property on="Box" class="Arr (strict)"() -> ("Value"=w142:T6)  [unwired: 2 in, 2 out]
        n918 = for {
          tunnel: w144 -> [w189]
          tunnel: w143 -> [w198]
          tunnel: w140 -> [w196] mode=indexing
          tunnel: w142 -> [w157] mode=indexing
          tunnel: w137 -> [w187]
          tunnel: w136 -> [w186]
          tunnel: w135 -> [w168]
          i -> [w167]
          w182 = T39 {"Draw"=TRUE, "Target"={"x"=20.0, "y"=20.0}, "Size"={"x"=20.0, "y"=20.0}, "Angle"=1250067.0, "Color"=1250067, "Thickness"=0, "CrosshairLabel"=""} ("Crosshair")
          w176 = T40 {"Left"=0, "Top"=0, "Right"=0, "Bottom"=0} ("Bounding Rectangle")
          n919 = call-poly <userlib>:"Filter 1D Array__ogtk.vi"("items to filter"=w196, "array"=w198) -> ("filtered item indices"=w199:i32[])  [unwired: 4 in, 1 out]
          n920 = Index Array(array=w199) -> (element=w188:i32)  [unwired: 1 in]
          n921 = Index Array(array=w168, index (row)=w167) -> (element=w165:dbl[])  [unwired: 1 in]
          n922 = Index Array(array=w187, index (row)=w167) -> (element=w175:dbl[])  [unwired: 1 in]
          n923 = Index Array(array=w186, index (row)=w167) -> (element=w173:dbl[])  [unwired: 1 in]
          n924 = Index Array(array=w189, index=w188) -> (element=w197:T29)
          n925 = Reverse 1D Array(array=w165) -> (reversed array=w164:dbl[])
          n926 = Unbundle By Name(w197) -> ("Target.X::12"=w201:refnum<vi>, "Target.Y::12"=w200:refnum<vi>)
          n927 = Reverse 1D Array(array=w175) -> (reversed array=w174:dbl[])
          n928 = Reverse 1D Array(array=w173) -> (reversed array=w172:dbl[])
          n929 = Index Array(array=w164) -> (element=w162:dbl)  [unwired: 1 in]
          n930 = Square Root(x=w162) -> (sqrt(x)=w161:dbl)
          n931 = Index Array(array=w172) -> (element=w169:dbl)  [unwired: 1 in]
          n932 = Index Array(array=w174) -> (element=w170:dbl)  [unwired: 1 in]
          n933 = Divide(x=w161, y=2.0) -> (x/y=w159:dbl)
          n934 = property class="DigNum (strict)"(reference=w201) -> ("Value"=w193:dbl)  [unwired: 1 in, 2 out]
          n935 = property class="DigNum (strict)"(reference=w200) -> ("Value"=w192:dbl)  [unwired: 1 in, 2 out]
          n936 = Bundle(cluster=cluster{"xhair size":dbl, "xhair size 2":dbl} {"xhair size"=25.0, "xhair size 2"=25.0} ("size"), "xhair size"=w159, "xhair size 2"=w159) -> (w163:cluster{"xhair size":dbl, "xhair size 2":dbl})
          n937 = Bundle By Name(cluster=w182, "Draw"=TRUE, "Target.x"=w193, "Target.y"=w192, "Size"=w163, "Color"=u32 16774656, "Angle"=0.0, "Thickness"=u8 1) -> (w195:T39)
          n938 = call "draw crosshair imaq.vi"("clear overlay"=TRUE, "Crosshair"=w195, "Bounding Rectangle"=w176, "image in"=w196) -> ("error out"=w179:errorcluster, "image out"=w178:T9)  [unwired: 6 in]
          n939 = Bundle By Name(cluster=w182, "Draw"=TRUE, "Target.x"=w170, "Target.y"=w169, "Size"=w163, "Color"=u32 8322834, "Angle"=0.0, "Thickness"=u8 1) -> (w180:T39)
          n940 = case shown="True" "average centroid" {
            tunnel: w180 -> [_ w206]
            tunnel: w179 -> [_ w211]
            tunnel: w178 -> [w203 w210]
            tunnel: w176 -> [_ w209]
            tunnel: w157 -> [w204 _]
            tunnel: [w202 w208] -> w156
            frame False {
              n941 = call "draw box imaq.vi"("Color"=u32 1244928, "Rectangle"=w204, "image in"=w203) -> ("error out"=w202:errorcluster)  [unwired: 7 in, 1 out]
            }
            frame True {
              n942 = call "draw crosshair imaq.vi"("clear overlay"=FALSE, "error in (no error)"=w211, "Crosshair"=w206, "Bounding Rectangle"=w209, "image in"=w210) -> ("error out"=w208:errorcluster)  [unwired: 5 in, 1 out]
            }
          }
          "error out 3" <- w156
        }
      }
      n943 = control-ref of="This Application"() -> (w126:refnum<vi>)
      n944 = control-ref of="This VI"() -> (w130:refnum<vi>)
      n945 = Current VI's Menubar() -> (w129:refnum<k9>)
      n946 = call "supergui create stop queue.vi"() -> ("STOP Queue out"=w32:refnum<queue>)  [unwired: 11 in]
      n947 = call "GUI_Master_subvi_reentrant_queues.vi"("STOP Queue in"=w32, "This Application"=w126, "error in (no error)"=w127, "tcp data event"=w125, "Caller menu reference"=w129, "Caller VI ref"=w130) -> ("error out"=→"error IO 2":errorcluster)  [unwired: 5 in]
      n948 = Unbundle By Name(w73) -> ("Data Value Reference out"=w72:refnum<k34>)
      n949 = for {
        tunnel: w102 -> [w134] mode=indexing
        tunnel: w101 -> [w133]
        tunnel: [w132] -> w71
        n950 = call "IMAQ Dispose"("Image"=w134, "error in (no error)"=w133) -> ("error out"=w132:errorcluster)  [unwired: 4 in]
      }
      n951 = TDMS Close(8:w71, 11:w72) -> (0:w33:errorcluster)  [unwired: 1 out]
      "error out 2" <- w33
      n952 = Release Queue(queue=w32, error in (no error)=w33) -> ()  [unwired: 1 in, 3 out]
      "Names" <- w42
    }
  }
